vi "EM9636M系列_主VI.vi"() -> ()   [LabVIEW 2016]
uses:
  <vilib>/Modbus/subvis/Modbus API/Modbus API.lvclass/Modbus API.ctl
  <vilib>/Modbus/subvis/Transmission Data Unit (ADU)/Transmission Data Unit/Transmission Data Unit.lvclass/Transmission Data Unit.ctl
  <vilib>/Modbus/master/Data Access/Unit ID/Set Unit ID Property.vi
  <vilib>/Modbus/subvis/Transmission Data Unit (ADU)/Transmission Data Unit/Data Access/Unit ID/Write Unit ID.vi
  <vilib>/Modbus/subvis/Modbus API/Read Transmission Data Unit.vi
  <vilib>/Modbus/subvis/Modbus API/Write Transmission Data Unit.vi
  <vilib>/Modbus/master/Modbus Master.lvclass
  <vilib>/Utility/NIReport.llb/Append Text Table to Report (wrap).vi
  <vilib>/Modbus/master/Create Master Instance (Serial).vi
  <vilib>/Modbus/subvis/Transmission Data Unit (ADU)/Transmission Data Unit/Transmission Data Unit.lvclass
  <vilib>/Utility/NIReport.llb/NI_report.lvclass
  <vilib>/ptbypt/NI_PtbyPt.lvlib
  <vilib>/Utility/miscctls.llb/LVRectTypeDef.ctl
panel:
  out "ini_R3":bool
  out "ini_D6":bool
  out "ini_D5":bool
  out "表格名称":string
  out "车型":string
  in  "簇 3":T1
  out "R3":dbl format="%#.2g"
  out "R2":dbl format="%#.2g"
  out "R1":dbl format="%#.2g"
  out "D6":dbl format="%#.2g"
  out "D5":dbl format="%#.2g"
  out "D4":dbl format="%#.2g"
  out "D3":dbl format="%#.2g"
  out "D2":dbl format="%#.2g"
  out "D1":dbl format="%#.2g"
  in  "簇":T1
  out "数据":T2(array[cluster])
  out "comcnt":u16
  out "对话框":bool
  out "到期了":bool
  out "变频6":bool
  out "变频5":bool
  out "变频4":bool
  out "变频3":bool
  out "变频2":bool
  out "变频1":bool
  in  "加载电机右下正反转":bool
  out "加载右下转矩监控":i16 format="%#.0f"
  in  "加载电机右下启动":bool caption="停止"
  out "加载电机右下母线电流":dbl
  out "加载电机右下母线电压":dbl
  out "加载转速右下监控":dbl
  in  "加载电机右下转速给定":i32
  in  "加载电机右下停机":bool caption="停止"
  out "加载电机右下运行？":bool
  in  "加载电机右下转矩给定":i16
  out "加载电机左下运行？":bool
  in  "加载电机左下转速给定":i32
  out "加载左下转速监控":dbl
  out "加载电机左下母线电压":dbl
  out "加载电机左下母线电流":dbl
  out "加载左下转矩监控":i16
  in  "加载电机左下停机":bool caption="停止"
  in  "加载电机左下启动":bool caption="停止"
  in  "加载电机左下正反转":bool
  in  "加载电机左下转矩给定":i16
  in  "加载电机右上正反转":bool
  out "加载转矩右上监控":i16 format="%#.0f"
  in  "加载电机右上启动":bool caption="停止"
  out "加载电机右上母线电流":dbl
  out "加载电机右上母线电压":dbl
  out "加载右上转速监控":dbl
  in  "加载电机右上转速给定":i32
  in  "加载电机右上停机":bool caption="停止"
  out "加载电机右上运行？":bool
  in  "加载电机右上转矩给定":i16
  out "加载电机左上运行？":bool
  in  "加载电机左上转速给定":i32
  out "加载左上转速监控":dbl
  out "加载电机左上母线电压":dbl
  out "加载电机左上母线电流":dbl
  out "加载左上转矩监控":i16
  in  "加载电机左上停机":bool caption="停止"
  in  "加载电机左上启动":bool caption="停止"
  in  "加载电机左上正反转":bool
  in  "加载电机左上转矩给定":i16
  in  "驱动电机上正反转":bool
  out "驱动转矩上监控":i16 format="%#.0f"
  in  "驱动电机上转矩给定":i16
  in  "驱动电机上启动":bool caption="停止"
  out "驱动电机上母线电流":dbl
  out "驱动电机上母线电压":dbl
  out "驱动上转速监控":dbl
  in  "驱动电机上转速给定":i16
  in  "驱动电机上停机":bool caption="停止"
  out "驱动电机上运行？":bool
  in  "驱动电机下正反转":bool
  out "驱动转矩下监控":i16 format="%#.0f"
  in  "驱动电机下转矩给定":i16
  in  "驱动电机下启动":bool caption="停止"
  out "驱动电机下母线电流":dbl
  out "驱动电机下母线电压":dbl
  out "驱动转速下监控":dbl
  in  "驱动电机转速下给定":i16
  in  "驱动电机下停机":bool caption="停止"
  out "驱动电机下运行？":bool
  out "轮询耗时":u32
  out "数值":i32
  out "对话框传递":bool
  out "超温报警":bool
  out "遥控器通讯":bool
  out "变频串口":bool
  in  "加载电机复位":bool caption="停止"
  out "变频器":bool
  out "前右":bool[](array[boolean])
  out "前左":bool[](array[boolean])
  out "中右":bool[](array[boolean])
  out "中左":bool[](array[boolean])
  out "后右":bool[](array[boolean])
  out "后左":bool[](array[boolean])
  in  "倒计时间S":dbl=600.0
  out "错误输出 7":errorcluster caption="错误输出"
  out "确认输入布尔":bool
  out "等待进车布尔":bool
  out "Config":T9={"DevType"=2, "DevIndex"=0, "CanIndex"=0, "VCI_INIT_CONFIG"={"AccCode"=0, "AccMask"=0, "InitFlag"=0, "Fliter"=0, "Timing0"=0, "Timing1"=0, "Mode"=0}} {"DevType" items=["USB-CAN"=3, "USB-CAN2"=4]; "CanIndex" items=["通道1", "通道2"]; "VCI_INIT_CONFIG"."Fliter" items=["接收所有类型"=3, "只接收标准帧"=4, "只接收扩展帧"=7]; "VCI_INIT_CONFIG"."Mode" items=["正常工作", "自测模式（环回）", "仅侦听模式"]; "VCI_INIT_CONFIG"."InitFlag" items=["使用Flash参数", "使用界面设置参数"]}
  in  "D1扭矩给定":i16=500
  in  "D2扭矩给定":i16=1000
  in  "D3扭矩给定":i16=1500
  in  "D4扭矩给定":i16=2000
  in  "D5扭矩给定":i16=3500
  in  "D6扭矩给定":i16=4000
  in  "R1扭矩给定":i16=500
  in  "R2扭矩给定":i16=1000
  in  "R3扭矩给定":i16=1500
  out "发送左侧字符":bool
  in  "Close":bool
  in  "Open 2":bool
  in  "AD开始采集 2":bool
  in  "AD开始采集":bool
  out "输出数组右":dbl[][](array[numeric])
  out "输出数组左":dbl[][](array[numeric])
  out "采集卡右":bool
  out "采集卡左":bool
  out "Open":bool
  out "close2":bool
  out "close":bool
  out "当前实验时间":string
  out "元素 2":bool
  out "元素":bool
  out "元素 4":bool
  out "元素 3":bool
  in  "速度温度":string[][](array[string]) caption="文本数据"
  out "实验基本信息":string[][](array[string])
  out "字符布尔":bool
  in  "Reset 9":bool caption="重置"
  in  "Reset 8":bool caption="重置"
  in  "Reset 7":bool caption="重置"
  in  "Reset 6":bool caption="重置"
  in  "Reset 5":bool caption="重置"
  in  "Reset 4":bool caption="重置"
  in  "Reset 3":bool caption="重置"
  in  "Reset 2":bool caption="重置"
  in  "Reset":bool caption="重置"
  out "R3平均速度":dbl
  out "R2平均速度":dbl
  out "R1平均速度":dbl
  out "D6平均速度":dbl
  out "D5平均速度":dbl
  out "D4平均速度":dbl
  out "D3平均速度":dbl
  out "D2平均速度":dbl
  out "平均速度数组":dbl[](array[numeric])
  out "D1平均速度":dbl
  out "停止布尔 2":bool
  out "停止布尔":bool
  out "启动布尔":bool
  out "485启动给遥控器布尔":bool
  in  "左5字符":u8=85 format="%x"
  in  "左4字符":u8=85 format="%x"
  in  "左3字符":u8=85 format="%x"
  in  "左2字符":u8=85 format="%x"
  in  "左1字符":u8=85 format="%x"
  out "布尔数组 2":bool[](array[boolean])
  out "布尔数组":bool[](array[boolean])
  in  "kBaudRate":u8(ring)=10 caption="波特率" items=["5k bps"=1, "10k bps"=2, "20k bps"=3, "40k bps"=4, "50k bps"=5, "80k bps"=6, "100k bps"=7, "125k bps"=8, "200k bps"=9, "250k bps"=10, "400k bps"=11, "500k bps"=12, "666k bps"=13, "800k bps"=14, "1000k bps"=15, "33.33k bps"=16, "66.66k bps"=17, "83.33k bps"=18]
  in  "Channel":T4 caption="CAN通道" items=["通道1", "通道2"]
  in  "DevType":T3=2 caption="设备类型" items=["USB-CAN"=2, "USB-CAN2"=3]
  out "中间数组":string[](array[string])
  in  "数值 2":dbl
  out "系统时间 2":string="系统时间"
  in  "ID_VCU_MCU_1 8":u32=522 format="0x%x"
  in  "ID_VCU_MCU_2 5":u32=522 format="0x%x"
  in  "ID_VCU_MCU_33 4":u32=522 format="0x%x"
  in  "ID_VCU_MCU_1 7":u32=522 format="0x%x"
  in  "0byte 13":u8=64 format="%x"
  in  "1byte 13":u8=6 format="%x"
  in  "2byte 13":u8=80 format="%x"
  in  "3byte 13":u8=111 format="%x"
  in  "4byte 13":u8=119 format="%x"
  in  "5byte 13":u8=101 format="%x"
  in  "6byte 13":u8=114 format="%x"
  in  "7byte 13":u8=32 format="%x"
  in  "0byte 14":u8=70 format="%x"
  in  "1byte 14":u8=2 format="%x"
  in  "2byte 14":u8=32 format="%x"
  in  "3byte 14":u8=32 format="%x"
  in  "4byte 14":u8 format="%x"
  in  "5byte 14":u8 format="%x"
  in  "6byte 14":u8 format="%x"
  in  "7byte 14":u8 format="%x"
  in  "0byte 15":u8=96 format="%x"
  in  "1byte 15":u8=6 format="%x"
  in  "2byte 15":u8=84 format="%x"
  in  "3byte 15":u8=85 format="%x"
  in  "4byte 15":u8=114 format="%x"
  in  "5byte 15":u8=113 format="%x"
  in  "6byte 15":u8=117 format="%x"
  in  "7byte 15":u8=101 format="%x"
  in  "0byte 16":u8=102 format="%x"
  in  "1byte 16":u8=2 format="%x"
  in  "2byte 16":u8=32 format="%x"
  in  "3byte 16":u8=32 format="%x"
  in  "4byte 16":u8 format="%x"
  in  "5byte 16":u8 format="%x"
  in  "6byte 16":u8 format="%x"
  in  "7byte 16":u8 format="%x"
  in  "ID_VCU_MCU_1 6":u32=522 format="0x%x"
  in  "ID_VCU_MCU_2 4":u32=522 format="0x%x"
  in  "ID_VCU_MCU_33 3":u32=522 format="0x%x"
  in  "ID_VCU_MCU_1 5":u32=522 format="0x%x"
  in  "0byte 5":u8=16 format="%x"
  in  "1byte 5":u8=6 format="%x"
  in  "2byte 5":u8=85 format="%x"
  in  "3byte 5":u8=85 format="%x"
  in  "4byte 5":u8=85 format="%x"
  in  "5byte 5":u8=85 format="%x"
  in  "6byte 5":u8=85 format="%x"
  in  "7byte 5":u8=85 format="%x"
  in  "0byte 6":u8=86 format="%x"
  in  "1byte 6":u8=2 format="%x"
  in  "2byte 6":u8=75 format="%x"
  in  "3byte 6":u8=119 format="%x"
  in  "4byte 6":u8 format="%x"
  in  "5byte 6":u8 format="%x"
  in  "6byte 6":u8 format="%x"
  in  "7byte 6":u8 format="%x"
  in  "0byte 7":u8=48 format="%x"
  in  "1byte 7":u8=6 format="%x"
  in  "2byte 7":u8=85 format="%x"
  in  "3byte 7":u8=85 format="%x"
  in  "4byte 7":u8=85 format="%x"
  in  "5byte 7":u8=85 format="%x"
  in  "6byte 7":u8=85 format="%x"
  in  "7byte 7":u8=85 format="%x"
  in  "0byte 8":u8=118 format="%x"
  in  "1byte 8":u8=2 format="%x"
  in  "2byte 8":u8=78 format="%x"
  in  "3byte 8":u8=109 format="%x"
  in  "4byte 8":u8 format="%x"
  in  "5byte 8":u8 format="%x"
  in  "6byte 8":u8 format="%x"
  in  "7byte 8":u8 format="%x"
  in  "ID_VCU_MCU_1 2":u32=522 format="0x%x"
  in  "ID_VCU_MCU_33":u32=522 format="0x%x"
  in  "ID_VCU_MCU_2 2":u32=522 format="0x%x"
  in  "ID_VCU_MCU_1":u32=522 format="0x%x"
  in  "ID_VCU_MCU_1 4":u32=522 format="0x%x"
  in  "ID_VCU_MCU_2 3":u32=522 format="0x%x"
  in  "ID_VCU_MCU_33 2":u32=522 format="0x%x"
  in  "ID_VCU_MCU_1 3":u32=522 format="0x%x"
  in  "0byte 9":u8 format="%x"
  in  "1byte 9":u8=6 format="%x"
  in  "2byte 9":u8=71 format="%x"
  in  "3byte 9":u8=101 format="%x"
  in  "4byte 9":u8=97 format="%x"
  in  "5byte 9":u8=114 format="%x"
  in  "6byte 9":u8=32 format="%x"
  in  "7byte 9":u8=32 format="%x"
  in  "0byte 10":u8=6 format="%x"
  in  "1byte 10":u8=2 format="%x"
  in  "2byte 10":u8=32 format="%x"
  in  "3byte 10":u8=32 format="%x"
  in  "4byte 10":u8 format="%x"
  in  "5byte 10":u8 format="%x"
  in  "6byte 10":u8 format="%x"
  in  "7byte 10":u8 format="%x"
  in  "0byte 11":u8=32 format="%x"
  in  "1byte 11":u8=6 format="%x"
  in  "2byte 11":u8=83 format="%x"
  in  "3byte 11":u8=112 format="%x"
  in  "4byte 11":u8=101 format="%x"
  in  "5byte 11":u8=101 format="%x"
  in  "6byte 11":u8=100 format="%x"
  in  "7byte 11":u8=32 format="%x"
  in  "0byte 12":u8=38 format="%x"
  in  "1byte 12":u8=2 format="%x"
  in  "2byte 12":u8=32 format="%x"
  in  "3byte 12":u8=32 format="%x"
  in  "4byte 12":u8 format="%x"
  in  "5byte 12":u8 format="%x"
  in  "6byte 12":u8 format="%x"
  in  "7byte 12":u8 format="%x"
  in  "0byte 4":u8=54 format="%x"
  in  "1byte 4":u8=2 format="%x"
  in  "2byte 4":u8=80 format="%x"
  in  "3byte 4":u8=109 format="%x"
  in  "4byte 4":u8 format="%x"
  in  "5byte 4":u8 format="%x"
  in  "6byte 4":u8 format="%x"
  in  "7byte 4":u8 format="%x"
  in  "0byte 3":u8=48 format="%x"
  in  "1byte 3":u8=6 format="%x"
  in  "2byte 3":u8=85 format="%x"
  in  "3byte 3":u8=85 format="%x"
  in  "4byte 3":u8=85 format="%x"
  in  "5byte 3":u8=85 format="%x"
  in  "6byte 3":u8=85 format="%x"
  in  "7byte 3":u8=82 format="%x"
  in  "0byte 2":u8=22 format="%x"
  in  "1byte 2":u8=2 format="%x"
  in  "2byte 2":u8=32 format="%x"
  in  "3byte 2":u8=32 format="%x"
  in  "4byte 2":u8 format="%x"
  in  "5byte 2":u8 format="%x"
  in  "6byte 2":u8 format="%x"
  in  "7byte 2":u8 format="%x"
  out "选项卡控件 4":enum32{"VCU控制", "CAN基本操作"}(tab)
  in  "Clear":bool
  in  "Mode":T8 caption="工作模式" items=["正常工作", "仅侦听模式", "自测模式（环回）"]
  in  "Fliter":T7=1 items=["接收所有类型"=1, "只接收标准帧"=2, "只接收扩展帧"=3]
  in  "AccMask":u32=4294967295 caption="接收屏蔽码" format="%08x"
  in  "AccCode":u32 caption="接收过滤码" format="%08x"
  out "SendCnt":u32 caption="发送统计"
  out "RecvCnt":u32 caption="接收统计"
  in  "RcvEnable":bool=TRUE
  in  "list":i32(listbox)
  in  "Send":bool
  in  "ID":u32 format="0x%x"
  in  "Type":u8(ring) items=["数据帧", "远程帧"]
  in  "Format":u8(ring) items=["标准帧", "扩展帧"]
  in  "Data":string="01 00"
  in  "0byte":u8=16 format="%x"
  in  "1byte":u8=6 format="%x"
  in  "2byte":u8=85 format="%x"
  in  "3byte":u8=85 format="%x"
  in  "4byte":u8=85 format="%x"
  in  "5byte":u8=85 format="%x"
  in  "6byte":u8=85 format="%x"
  in  "7byte":u8=85 format="%x"
  in  "InitFlag":T6=1 caption="初始化参数" items=["使用Flash参数", "使用界面设置参数"]
  in  "选项卡控件 3":enum32{"数据监视", "查看数据"}(tab)
  in  "具体车型":string
  in  "确认换挡":bool
  in  "重新选档档位":T10(ring)
  out "前右":bool
  out "中右":bool
  out "后右":bool
  out "前左":bool
  out "中左":bool
  out "后左":bool
  out "R3S":dbl format="%#.2g"
  out "R2S":dbl format="%#.2g"
  out "R1S":dbl format="%#.2g"
  out "D6S":dbl format="%#.2g"
  out "D5S":dbl format="%#.2g"
  out "D4S":dbl format="%#.2g"
  out "D3S":dbl format="%#.2g"
  out "D2S":dbl format="%#.2g"
  out "D1S":dbl format="%#.2g"
  in  "刷新参数":bool
  out "LED屏幕信息":string
  in  "高级参数":bool
  in  "重新实验":bool
  in  "生成报表":bool
  in  "确认输入":bool
  in  "遥控器按钮确认":bool
  out "总实验时间":string
  out "前右":dbl format="%#.2g"
  out "前左":dbl format="%#.2g"
  out "中右":dbl
  out "中左":dbl format="%#.2g"
  out "后右":dbl format="%#.2g"
  out "后左":dbl format="%#.2g"
  out "后右":dbl format="%#.2g"
  out "后左":dbl format="%#.2g"
  out "中右":dbl format="%#.2g"
  out "中左":dbl format="%#.2g"
  out "前右":dbl format="%#.2g"
  out "前左":dbl format="%#.2g"
  out "环境温度标定":dbl format="%#.2g"
  out "波形图表":dynamicdata(graph)
  in  "操作者":string
  out "加载扭矩N.M(单个）":dbl
  out "当前试验档位":string
  in  "试验车型":u16(ring) items=["SG21", "SG14", "SG16", "SG18"]
  out "车速":dbl(knob) scale=-30.0..30.0
  in  "试验车编号":string
  in  "发动机编号":string
  out "加载功率":dbl(knob) scale=0.0..30.0
  in  "试验开始":bool caption="停止"
  in  "停止":bool
  out "液压油箱温度标定":dbl format="%#.2g"
  out "变矩器出口温度标定":dbl format="%#.2g"
  out "右前轮轴承温度标定":dbl format="%#.2g"
  out "左前轮轴承温度标定":dbl format="%#.2g"
  out "振动泵压力":dbl format="%#.2g"
  out "转向泵压力":dbl format="%#.2g"
  in  "密码输入":string
  out "SG14百分比":dbl
  out "SG16-3百分比":dbl
  out "SG18-3百分比":dbl
  out "D1 act":dbl format="%#.2g"
  out "D2 act":dbl format="%#.2g"
  out "R3 act":dbl format="%#.2g"
  out "R2 act":dbl format="%#.2g"
  out "R1 act":dbl format="%#.2g"
  out "D6 act":dbl format="%#.2g"
  out "D5 act":dbl format="%#.2g"
  out "D4 act":dbl format="%#.2g"
  out "D3 act":dbl format="%#.2g"
  out "数值 3":i32
  out "前右电机右轴承振动":dbl
  out "前右电机左轴承振动":dbl
  out "前右滚筒右轴承振动":dbl
  out "前右滚筒左轴承振动":dbl
  out "后左滚筒右振动":dbl
  out "后左滚筒左振动":dbl
  out "中右电机右振动":dbl
  out "中右电机左振动":dbl
  out "中右滚筒右振动":dbl
  out "中右滚筒左振动":dbl
  out "中左电机右轴承振动":dbl
  out "中左电机左轴承振动":dbl
  out "中左滚筒右轴承振动":dbl
  out "中左滚筒左轴承振动":dbl
  out "前左电机右轴承振动":dbl
  out "前左电机左轴承振动":dbl
  out "前左滚筒右轴承振动":dbl
  out "前左滚筒左轴承振动":dbl
  out "后右电机右振动":dbl
  out "后右电机左振动":dbl
  out "后右滚筒右振动":dbl
  out "后右滚筒左振动":dbl
  out "后左电机右振动":dbl
  out "后左电机左振动":dbl
  out "后右电机绕组":dbl
  out "后右电机右轴承":dbl
  out "后右滚筒左轴承":dbl
  out "后左滚筒右轴承":dbl
  out "后右滚筒左轴承":dbl
  out "后左电机绕组":dbl
  out "后左电机右轴承":dbl
  out "后左电机左轴承":dbl
  out "后左滚筒右轴承":dbl
  out "后左滚筒左轴承":dbl
  out "中右电机绕组":dbl
  out "中右电机右轴承":dbl
  out "中右电机左轴承":dbl
  out "中右滚筒右轴承":dbl
  out "中右滚筒左轴承":dbl
  out "中左电机绕组":dbl
  out "中左电机右轴承":dbl
  out "中左电机左轴承":dbl
  out "中左滚筒右轴承":dbl
  out "中左滚筒左轴承":dbl
  out "前右电机绕组":dbl
  out "前右电机右轴承":dbl
  out "前右滚筒左轴承":dbl
  out "前左滚筒右轴承":dbl
  out "前右滚筒左轴承":dbl
  out "前左电机绕组":dbl
  out "前左电机右轴承":dbl
  out "前左电机左轴承":dbl
  out "前左滚筒右轴承":dbl
  out "前左滚筒左轴承":dbl
  out "错误输出 6":errorcluster caption="错误输出"
  out "AD均值数据 2":dbl[](array[numeric])
  in  "M系列PWM停止 2":bool
  in  "编码器清零 2":bool
  in  "DA输出 2":bool
  in  "DA输出范围 2":i32(ring) items=["±10V", "±5V", "0~10V（默认）", "0~5V", "0~20mA"]
  in  "CH1 2":i16(slide) scale=0.0..10000.0
  in  "CH3 2":i16(slide) scale=0.0..10000.0
  in  "CH4 2":i16(slide) scale=0.0..10000.0
  in  "CH2 2":i16(slide) scale=0.0..10000.0
  in  "设定输出脉冲个数 2":u32
  in  "M系列PWM输出 2":bool
  in  "AD停止采集 2":bool
  out "布尔 2":bool
  in  "通道频率Hz 2":dbl=10000.0 min=1000.0 max=100000.0 step=10.0
  in  "组频率Hz 2":dbl=500.0
  in  "单双端 2":i32(ring) items=["单端", "双端"]
  in  "AD终止通道 2":i32=32
  in  "AD起始通道 2":i32=1
  in  "增益 2":i32(ring) items=["无增益", "2倍增益", "5倍增益", "10倍增益"]
  in  "伪同步 2":i32(ring) items=["非伪同步", "伪同步"]
  in  "时钟源 2":i32(ring) items=["内时钟", "外时钟"]
  out "每次总数据量 2":i32
  out "通道数量 2":i32
  in  "AD范围 2":enum16{"-10~+10V", "-5V~+5V", "0~10V", "0~5V"}(ring)=enum."0~10V"
  out "每通道数据量 2":i32
  out "编码器AB值 2":i32[](array[numeric])
  out "编码器过零值 2":i16[](array[numeric])
  out "错误输出 5":errorcluster caption="错误输出3"
  out "错误输出 4":errorcluster caption="错误输出2"
  out "设备句柄 2":i32=1
  in  "选项卡控件 2":enum32{"AD数值显示", "数字量I/O", "(标准)PWM", "计数器（测频）"}(tab)
  in  "设置开关量方向 3":bool
  out "数组 5":dbl[](array[numeric])=[1.0, 2.0, 3.0, 4.0, 5.0, 6.0, 7.0, 8.0]
  out "数组 6":dbl[](array[numeric])=[1.0, 2.0, 3.0, 4.0, 5.0, 6.0, 7.0, 8.0]
  in  "光隔离输出 2":bool[](array[boolean])=[FALSE, FALSE, FALSE, FALSE, FALSE, FALSE, FALSE, FALSE]
  out "光隔离输入 2":bool[](array[boolean])
  in  "设置开关量方向 2":cluster{"IO1~IO8":i8, "IO9~IO16":i8}={"IO1~IO8"=1, "IO9~IO16"=1} {"IO9~IO16" items=["输入", "输出"]; "IO1~IO8" items=["输入", "输出"]}
  out "数组 7":i8[](array[numeric])
  in  "可编程数字量I/O 2":T11
  out "可编程数字量I/O(映射控件)--得到所有通道开关量值 2":T11
  in  "PWM输出 2":bool
  in  "PWM停止 2":bool
  in  "频率1 2":dbl=1000.0
  in  "占空比(0~1) 6":dbl=0.5
  out "实际频率 6":dbl
  out "实际占空比 6":dbl
  in  "频率2 2":dbl=5000.0
  in  "占空比(0~1) 5":dbl=0.5
  out "实际频率 5":dbl
  out "实际占空比 5":dbl
  in  "频率3 2":dbl=100000.0
  in  "占空比(0~1) 4":dbl=0.5
  out "实际频率 4":dbl
  out "实际占空比 4":dbl
  in  "开启计数 2":bool
  in  "计数器清零 2":bool
  in  "工作方式 2":u16(ring)=1 items=["计数", "测频"]
  out "计数/测频（Hz）值 2":dbl[](array[numeric])
  in  "编码器清零":bool
  out "编码器AB值":i32[](array[numeric])
  out "编码器过零值":i16[](array[numeric])
  in  "设定输出脉冲个数":u32
  in  "M系列PWM输出":bool
  in  "M系列PWM停止":bool
  in  "CH4":i16(slide) scale=0.0..10000.0
  in  "CH3":i16(slide) scale=0.0..10000.0
  in  "CH2":i16(slide) scale=0.0..10000.0
  in  "CH1":i16(slide) scale=0.0..10000.0
  in  "DA输出":bool
  in  "DA输出范围":i32(ring) items=["±10V", "±5V", "0~10V（默认）", "0~5V", "0~20mA"]
  out "每通道数据量":i32
  out "AD均值数据":dbl[](array[numeric])
  out "布尔":bool
  in  "AD停止采集":bool
  out "错误输出 3":errorcluster caption="错误输出3"
  out "错误输出 2":errorcluster caption="错误输出2"
  in  "选项卡控件":enum32{"AD数值显示", "数字量I/O", "(标准)PWM", "计数器（测频）"}(tab)
  out "变频故障1":bool
  out "变频故障2":bool
  out "变频故障 3":bool
  out "变频故障 4":bool
  out "变频故障5":bool
  out "变频故障 6":bool
  in  "设置开关量方向":bool
  out "数组 3":dbl[](array[numeric])=[1.0, 2.0, 3.0, 4.0, 5.0, 6.0, 7.0, 8.0]
  out "数组 2":dbl[](array[numeric])=[1.0, 2.0, 3.0, 4.0, 5.0, 6.0, 7.0, 8.0]
  in  "光隔离输出":bool[](array[boolean])=[FALSE, FALSE, FALSE, FALSE, FALSE, FALSE, FALSE, FALSE]
  out "光隔离输入":bool[](array[boolean])
  in  "设置开关量方向":cluster{"IO1~IO8":i8, "IO9~IO16":i8}={"IO1~IO8"=1, "IO9~IO16"=1} {"IO9~IO16" items=["输入", "输出"]; "IO1~IO8" items=["输入", "输出"]}
  out "数组 4":i8[](array[numeric])
  in  "可编程数字量I/O":T11
  out "可编程数字量I/O(映射控件)--得到所有通道开关量值":T11
  in  "PWM输出":bool
  in  "PWM停止":bool
  in  "频率1":dbl=1000.0
  in  "占空比(0~1)":dbl=0.5
  out "实际频率":dbl
  out "实际占空比":dbl
  in  "频率2":dbl=5000.0
  in  "占空比(0~1) 2":dbl=0.5
  out "实际频率 2":dbl
  out "实际占空比 2":dbl
  in  "频率3":dbl=100000.0
  in  "占空比(0~1) 3":dbl=0.5
  out "实际频率 3":dbl
  out "实际占空比 3":dbl
  in  "开启计数":bool
  in  "计数器清零":bool
  in  "工作方式":u16(ring)=1 items=["计数", "测频"]
  out "计数/测频（Hz）值":dbl[](array[numeric])
  in  "AD范围":enum16{"-10~+10V", "-5V~+5V", "0~10V", "0~5V"}(ring)=enum."0~10V"
  out "通道数量":i32
  out "设备句柄":i32=1
  out "错误输出":errorcluster
  out "每次总数据量":i32
  in  "时钟源":i32(ring) items=["内时钟", "外时钟"]
  in  "伪同步":i32(ring) items=["非伪同步", "伪同步"]
  in  "增益":i32(ring) items=["无增益", "2倍增益", "5倍增益", "10倍增益"]
  in  "AD起始通道":i32=1
  in  "AD终止通道":i32=32
  in  "单双端":i32(ring) items=["单端", "双端"]
  in  "组频率Hz":dbl=500.0
  in  "通道频率Hz":dbl=10000.0 min=1000.0 max=100000.0 step=10.0
  in  "数据端口":i32=8001
  in  "命令端口":i32=8000
  in  "IP地址":string="192.168.1.125"
  # "加载电机右上"
  # "驱动电机上"
  # "加载电机左上"
  # "r/min"
  # "r/min"
  # "r/min"
  # "转速"
  # "给定"
  # "转速"
  # "给定"
  # "转速"
  # "给定"
  # "给定"
  # "Nm"
  # "Nm"
  # "Nm"
  # "转矩"
  # "转矩"
  # "给定"
  # "转矩"
  # "给定"
  # "山推平地机实验台"
  # "电压"
  # "电流"
  # "电压"
  # "电流"
  # "电压"
  # "V"
  # "电流"
  # "A"
  # "A"
  # "V"
  # "A"
  # "V"
  # "遥控器"
  # "变频器"
  # "采集卡左"
  # "采集卡右"
  # "超温报警"
  # "正转"
  # "反转"
  # "正转"
  # "正转"
  # "反转"
  # "反转"
  # "加载电机右下"
  # "驱动电机下"
  # "加载电机左下"
  # "r/min"
  # "r/min"
  # "r/min"
  # "转速"
  # "给定"
  # "转速"
  # "给定"
  # "转速"
  # "给定"
  # "给定"
  # "Nm"
  # "Nm"
  # "Nm"
  # "转矩"
  # "转矩"
  # "给定"
  # "转矩"
  # "给定"
  # "电压"
  # "电流"
  # "电压"
  # "电流"
  # "电压"
  # "V"
  # "电流"
  # "A"
  # "V"
  # "A"
  # "V"
  # "A"
  # "正转"
  # "反转"
  # "正转"
  # "正转"
  # "反转"
  # "反转"
  # "D1"
  # "D6扭矩给定"
  # "~"
  # "R1"
  # "R3扭矩给定"
  # "~"
  # "EM9636M系列--LabView例程"
  # "CH1"
  # "CH2"
  # "如果设为0，则表示连续输出"
  # "CH1"
  # "CH2"
  # "位置传感器故障"
  # "过流"
  # "控制器过温"
  # "电机过温"
  # "欠压报警"
  # "过压报警"
  # "通讯故障"
  # "控制器高温"
  # "短路保护"
  # "严重欠压"
  # "超过峰值功率"
  # "超过最高限速"
  # "VCU故障"
  # "跛行状态"
  # "堵转保护"
  # "致命故障"
  # "车辆参数"
  # "设备参数"
  # "环境温度"
  # "前左"
  # "℃"
  # "℃"
  # "r/min"
  # "r/min"
  # "r/min"
  # "液压油箱温度"
  # "℃"
  # "前右"
  # "℃"
  # "r/min"
  # "r/min"
  # "r/min"
  # "变速箱温度"
  # "℃"
  # "中左"
  # "℃"
  # "右前轮轴承温度"
  # "中右"
  # "℃"
  # "℃"
  # "左前轮轴承温度"
  # "~"
  # "D1   R3/%"
  # "℃"
  # "后左"
  # "℃"
  # "~"
  # "D1   R3/S"
  # "Mp"
  # "工作泵压力"
  # "后右"
  # "℃"
  # "转向泵压力"
  # "Mp"
  # "前左滚筒左轴承"
  # "后左滚筒左轴承"
  # "℃"
  # "℃"
  # "后左电机左振动"
  # "前右滚筒左振动"
  # "前左滚筒右轴承"
  # "后左滚筒右轴承"
  # "℃"
  # "℃"
  # "后左电机右振动"
  # "前右滚筒右振动"
  # "前左电机左轴承"
  # "后左电机左轴承"
  # "℃"
  # "后右滚筒左振动"
  # "℃"
  # "前右电机左振动"
  # "前左电机右轴承"
  # "后左电机右轴承"
  # "℃"
  # "℃"
  # "后右滚筒右振动"
  # "前右电机右振动"
  # "前左电机绕组"
  # "后左电机绕组"
  # "后右电机左振动"
  # "℃"
  # "℃"
  # "前右滚筒左轴承"
  # "后右滚筒左轴承"
  # "后右电机右振动"
  # "℃"
  # "℃"
  # "前右滚筒右轴承"
  # "后右滚筒右轴承"
  # "前左滚筒左振动"
  # "℃"
  # "℃"
  # "前右电机左轴承"
  # "后右电机左轴承"
  # "前右滚筒右振动"
  # "℃"
  # "℃"
  # "前右电机右轴承"
  # "后右电机右轴承"
  # "前左电机左振动"
  # "℃"
  # "℃"
  # "前右电机绕组"
  # "后右电机绕组"
  # "℃"
  # "℃"
  # "前左电机右振动"
  # "中左滚筒左轴承"
  # "℃"
  # "中左滚筒左振动"
  # "中左滚筒右轴承"
  # "℃"
  # "中左滚筒右振动"
  # "中左电机左轴承"
  # "中左电机左振动"
  # "℃"
  # "中左电机右轴承"
  # "℃"
  # "中左电机右振动"
  # "中左电机绕组"
  # "℃"
  # "中右滚筒左振动"
  # "中右滚筒左轴承"
  # "中右滚筒右振动"
  # "℃"
  # "中右滚筒右轴承"
  # "中右电机左振动"
  # "℃"
  # "中右电机左轴承"
  # "中右电机右振动"
  # "℃"
  # "中右电机右轴承"
  # "后左滚筒左振动"
  # "℃"
  # "中右电机绕组"
  # "℃"
  # "后左滚筒右振动"
  # "通道3"
  # "通道1"
  # "通道2"
  # "频率，250Hz~500KHz\n占空比，0~1"
  # "通道3"
  # "通道1"
  # "通道2"
  # "频率，250Hz~500KHz\n占空比，0~1"
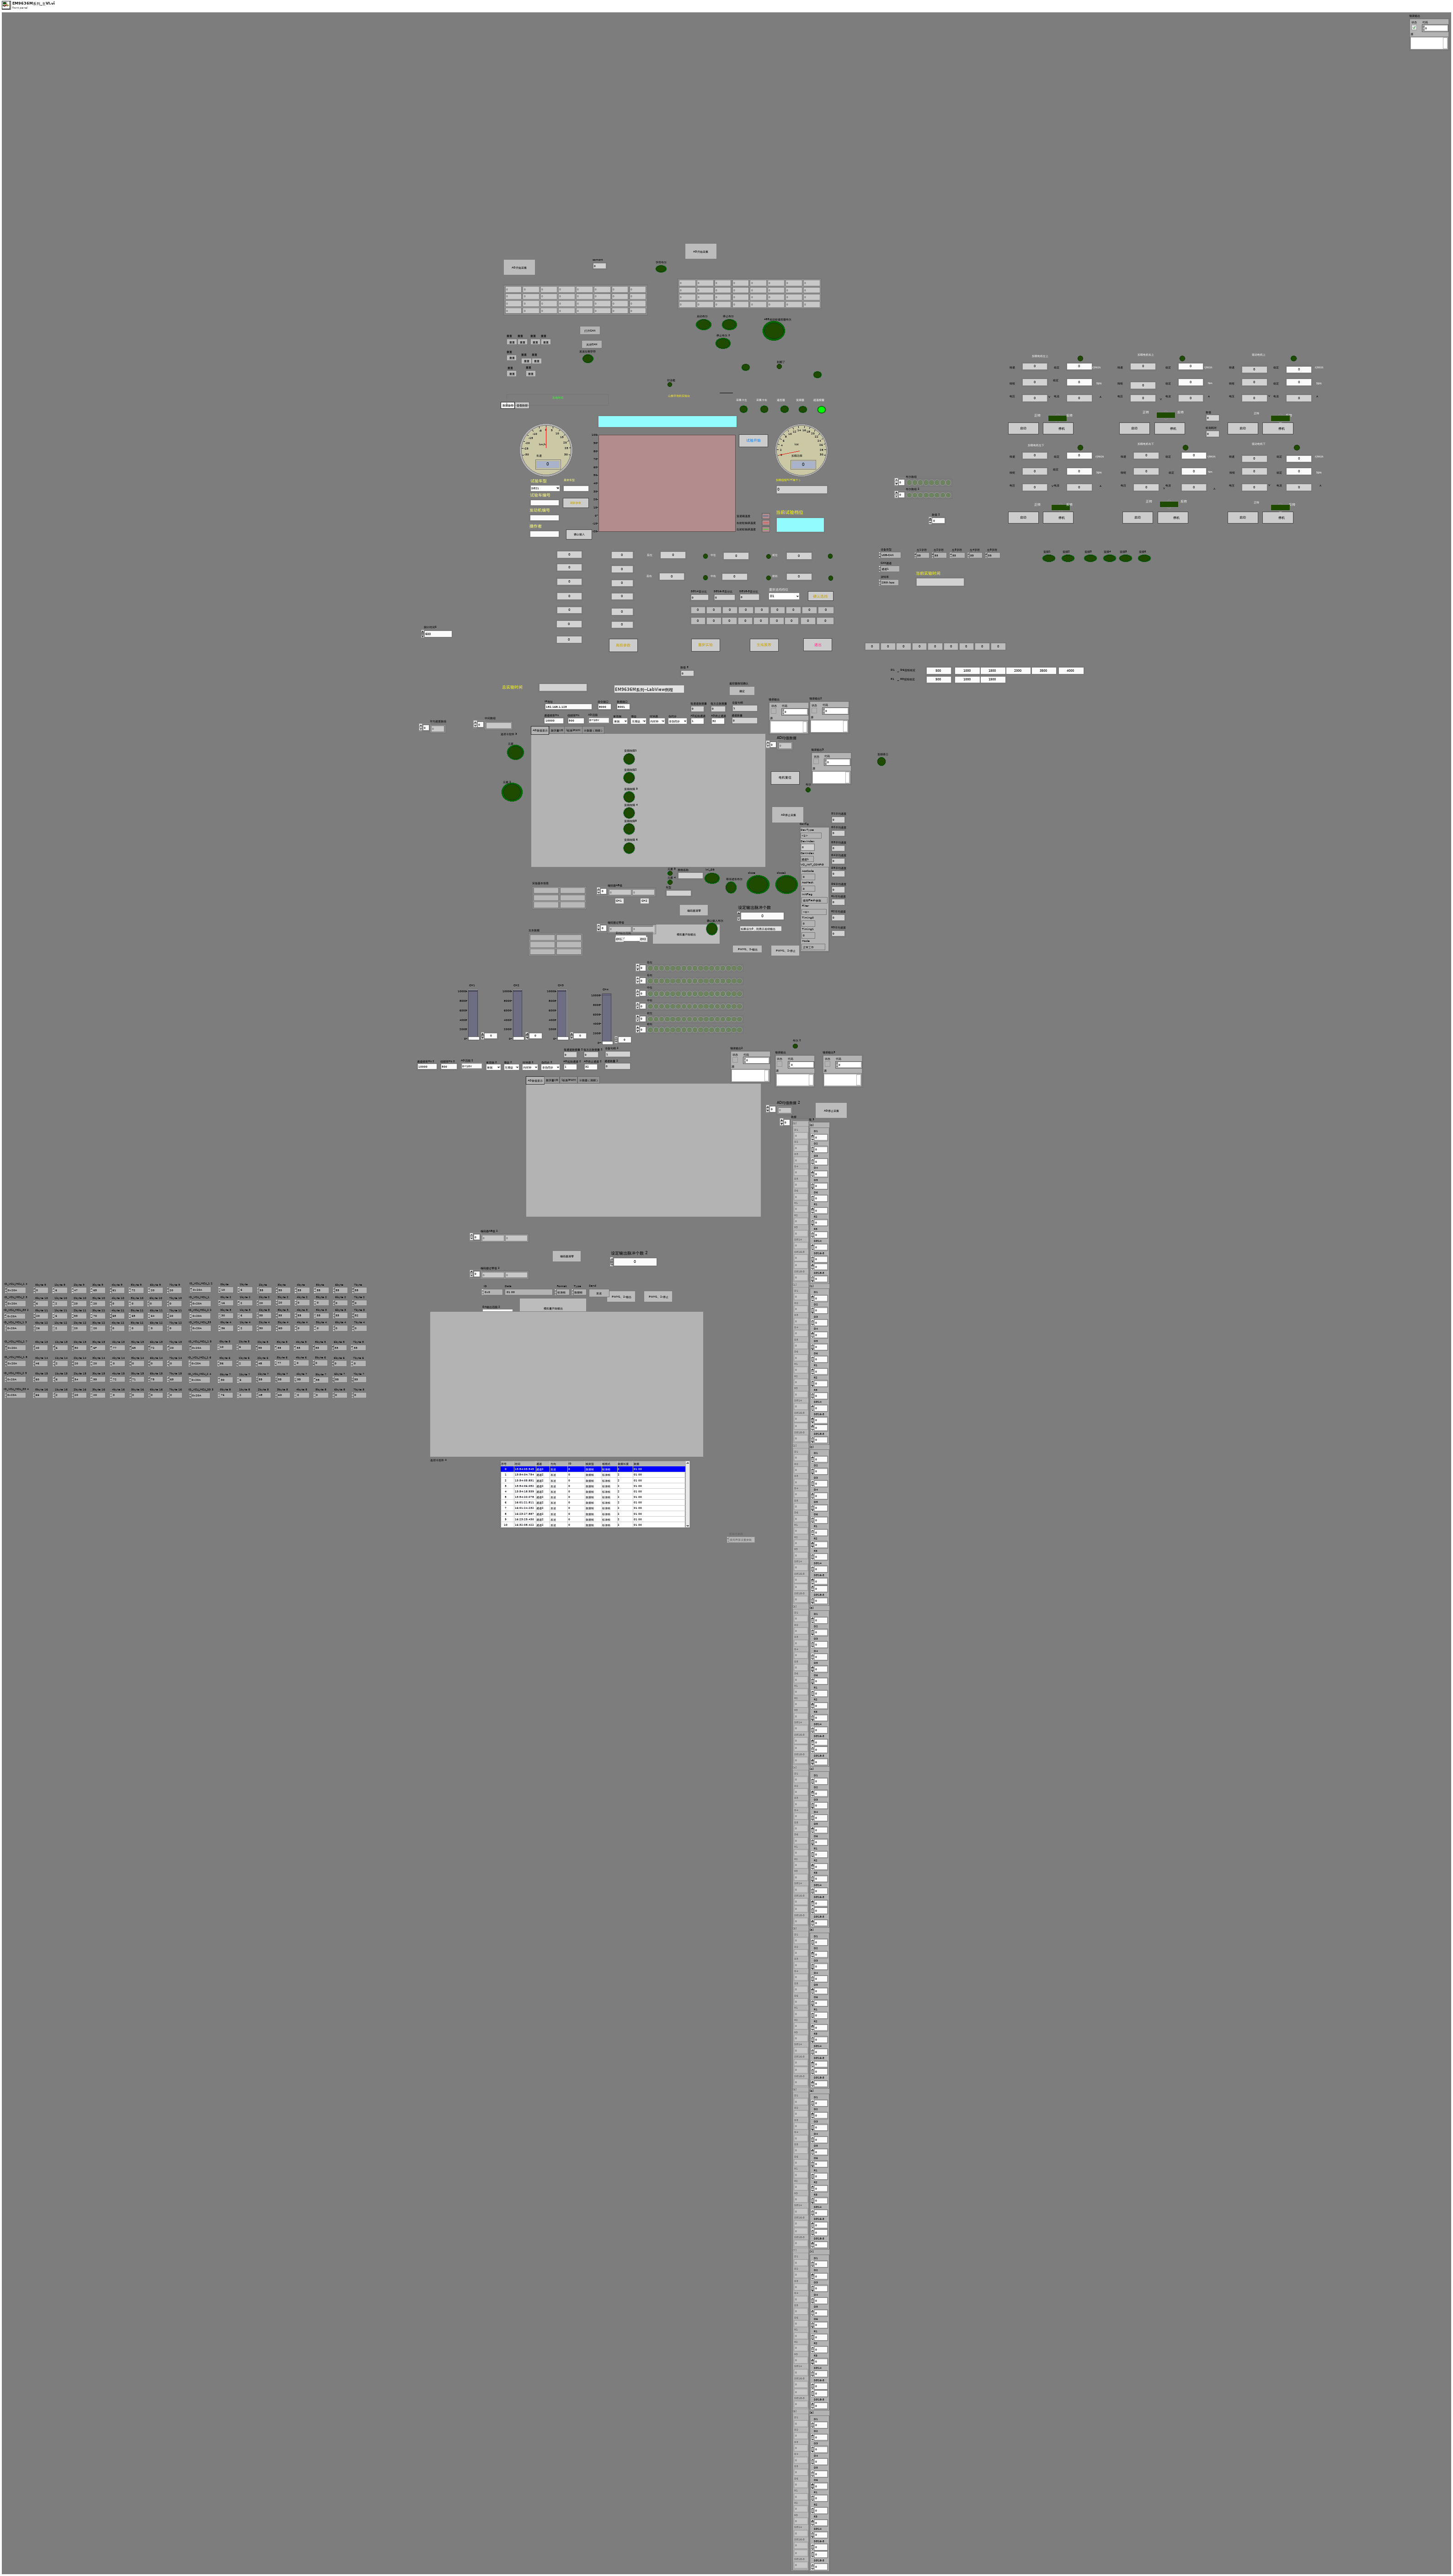
[diagram p1: front panel]
types:
  T1 = cluster{"[0]":cluster{"D1":dbl, "D2":dbl, "D3":dbl, "D4":dbl, "D5":dbl, "D6":dbl, "R1":dbl, "R2":dbl, "R3":dbl, "SG14":dbl, "SG16-3":dbl, dbl, "SG18-3 ":dbl}, "[1]":cluster{"D1":dbl, "D2":dbl, "D3":dbl, "D4":dbl, "D5":dbl, "D6":dbl, "R1":dbl, "R2":dbl, "R3":dbl, "SG14":dbl, "SG16-3":dbl, dbl, "SG18-3 ":dbl}, "[2]":cluster{"D1":dbl, "D2":dbl, "D3":dbl, "D4":dbl, "D5":dbl, "D6":dbl, "R1":dbl, "R2":dbl, "R3":dbl, "SG14":dbl, "SG16-3":dbl, dbl, "SG18-3 ":dbl}, "[3]":cluster{"D1":dbl, "D2":dbl, "D3":dbl, "D4":dbl, "D5":dbl, "D6":dbl, "R1":dbl, "R2":dbl, "R3":dbl, "SG14":dbl, "SG16-3":dbl, dbl, "SG18-3 ":dbl}, "[4]":cluster{"D1":dbl, "D2":dbl, "D3":dbl, "D4":dbl, "D5":dbl, "D6":dbl, "R1":dbl, "R2":dbl, "R3":dbl, "SG14":dbl, "SG16-3":dbl, dbl, "SG18-3 ":dbl}, "[5]":cluster{"D1":dbl, "D2":dbl, "D3":dbl, "D4":dbl, "D5":dbl, "D6":dbl, "R1":dbl, "R2":dbl, "R3":dbl, "SG14":dbl, "SG16-3":dbl, dbl, "SG18-3 ":dbl}, "[6]":cluster{"D1":dbl, "D2":dbl, "D3":dbl, "D4":dbl, "D5":dbl, "D6":dbl, "R1":dbl, "R2":dbl, "R3":dbl, "SG14":dbl, "SG16-3":dbl, dbl, "SG18-3 ":dbl}, "[7]":cluster{"D1":dbl, "D2":dbl, "D3":dbl, "D4":dbl, "D5":dbl, "D6":dbl, "R1":dbl, "R2":dbl, "R3":dbl, "SG14":dbl, "SG16-3":dbl, dbl, "SG18-3 ":dbl}, "[8]":cluster{"D1":dbl, "D2":dbl, "D3":dbl, "D4":dbl, "D5":dbl, "D6":dbl, "R1":dbl, "R2":dbl, "R3":dbl, "SG14":dbl, "SG16-3":dbl, dbl, "SG18-3 ":dbl}}
  T2 = cluster{"[0]":cluster{"D1":dbl, "D2":dbl, "D3":dbl, "D4":dbl, "D5":dbl, "D6":dbl, "R1":dbl, "R2":dbl, "R3":dbl, "SG14":dbl, "SG16-3":dbl, dbl, "SG18-3 ":dbl}, "[1]":cluster{"D1":dbl, "D2":dbl, "D3":dbl, "D4":dbl, "D5":dbl, "D6":dbl, "R1":dbl, "R2":dbl, "R3":dbl, "SG14":dbl, "SG16-3":dbl, dbl, "SG18-3 ":dbl}, "[2]":cluster{"D1":dbl, "D2":dbl, "D3":dbl, "D4":dbl, "D5":dbl, "D6":dbl, "R1":dbl, "R2":dbl, "R3":dbl, "SG14":dbl, "SG16-3":dbl, dbl, "SG18-3 ":dbl}, "[3]":cluster{"D1":dbl, "D2":dbl, "D3":dbl, "D4":dbl, "D5":dbl, "D6":dbl, "R1":dbl, "R2":dbl, "R3":dbl, "SG14":dbl, "SG16-3":dbl, dbl, "SG18-3 ":dbl}, "[4]":cluster{"D1":dbl, "D2":dbl, "D3":dbl, "D4":dbl, "D5":dbl, "D6":dbl, "R1":dbl, "R2":dbl, "R3":dbl, "SG14":dbl, "SG16-3":dbl, dbl, "SG18-3 ":dbl}, "[5]":cluster{"D1":dbl, "D2":dbl, "D3":dbl, "D4":dbl, "D5":dbl, "D6":dbl, "R1":dbl, "R2":dbl, "R3":dbl, "SG14":dbl, "SG16-3":dbl, dbl, "SG18-3 ":dbl}, "[6]":cluster{"D1":dbl, "D2":dbl, "D3":dbl, "D4":dbl, "D5":dbl, "D6":dbl, "R1":dbl, "R2":dbl, "R3":dbl, "SG14":dbl, "SG16-3":dbl, dbl, "SG18-3 ":dbl}, "[7]":cluster{"D1":dbl, "D2":dbl, "D3":dbl, "D4":dbl, "D5":dbl, "D6":dbl, "R1":dbl, "R2":dbl, "R3":dbl, "SG14":dbl, "SG16-3":dbl, dbl, "SG18-3 ":dbl}, "[8]":cluster{"D1":dbl, "D2":dbl, "D3":dbl, "D4":dbl, "D5":dbl, "D6":dbl, "R1":dbl, "R2":dbl, "R3":dbl, "SG14":dbl, "SG16-3":dbl, dbl, "SG18-3 ":dbl}}[]
  T3 = typedef "ControlCAN.lvlib/DevType.ctl" = u32
  T4 = typedef "ControlCAN.lvlib/CAN Channel.ctl" = u32
  T5 = typedef "ControlCAN.lvlib/VCI_INIT_CONFIG.ctl" = cluster{"AccCode":u32, "AccMask":u32, "InitFlag":T6, "Fliter":T7, "Timing0":u8, "Timing1":u8, "Mode":T8}
  T6 = typedef "ControlCAN.lvlib/InitFlag.ctl" = u32
  T7 = typedef "ControlCAN.lvlib/Fliter.ctl" = u8
  T8 = typedef "ControlCAN.lvlib/Mode.ctl" = u8
  T9 = cluster{"DevType":T3, "DevIndex":u32, "CanIndex":T4, "VCI_INIT_CONFIG":T5}
  T10 = enum16{"D1", "D2", "D3", "D4", "D5", "D6", "R1", "R2", "R3"}
  T11 = cluster{"CH1":bool, "CH2":bool, "CH3":bool, "CH4":bool, "CH5":bool, "CH6":bool, "CH7":bool, "CH8":bool, "CH9":bool, "CH10":bool, "CH11":bool, "CH12":bool, "CH13":bool, "CH14":bool, "CH15":bool, "CH16":bool}
  T12 = typedef "ControlCAN.lvlib/VCI_CAN_OBJ.ctl" = cluster{"ID":u32, "TimeStamp":u32, "TimeFlag":u8, "SendType":u8, "RemoteFlag":u8, "ExternFlag":u8, "DataLen":u8, "Data":u8[], "Reserved":u8[]}
  T13 = cluster{"Type":enum16{"接收", "发送"}, "Channel":T4, "Time":timestamp, "VCI_CAN_OBJ":T12}[]
  T14 = typedef "LVRectTypeDef.ctl" = cluster{"Left":i16, "Top":i16, "Right":i16, "Bottom":i16}
  T15 = cluster{"position (excel)":cluster{"row":i32, "column":i32}, "name (excel)":string, "bookmark (word)":string}
  T16 = enum16{"Standard Report", "HTML", "Word", "Excel"}
  T17 = enum32{"Invalid", "Standard", "Closed", "Hidden", "Minimized", "Maximized"}
  T18 = cluster{"D1":dbl, "D2":dbl, "D3":dbl, "D4":dbl, "D5":dbl, "D6":dbl, "R1":dbl, "R2":dbl, "R3":dbl, "SG14":dbl, "SG16-3":dbl, dbl, "SG18-3 ":dbl}
  T19 = enum32{"invalid app kind", "Development System", "Run Time System", "Student Edition", "Embedded LabVIEW", "Evaluation", "Custom"}
  T20 = cluster{"Type":enum16{"接收", "发送"}, "Channel":T4, "Time":timestamp, "VCI_CAN_OBJ":T12}
  T21 = typedef "ControlCAN.lvlib/Return Val.ctl" = i32
  T22 = cluster{"[0]":bool, "[1]":bool, "[2]":bool, "[3]":bool, "[4]":bool, "[5]":bool, "[6]":bool, "[7]":bool, "[8]":bool, "[9]":bool, "[10]":bool, "[11]":bool, "[12]":bool, "[13]":bool, "[14]":bool, "[15]":bool}
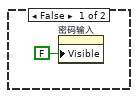
[diagram p4: hidden frame]
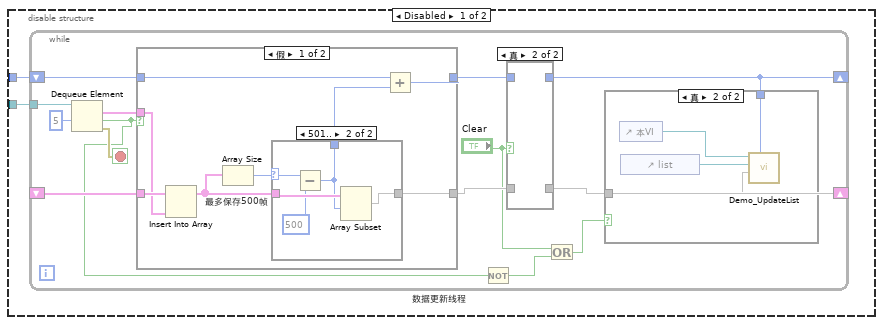
[diagram p8: hidden frame]
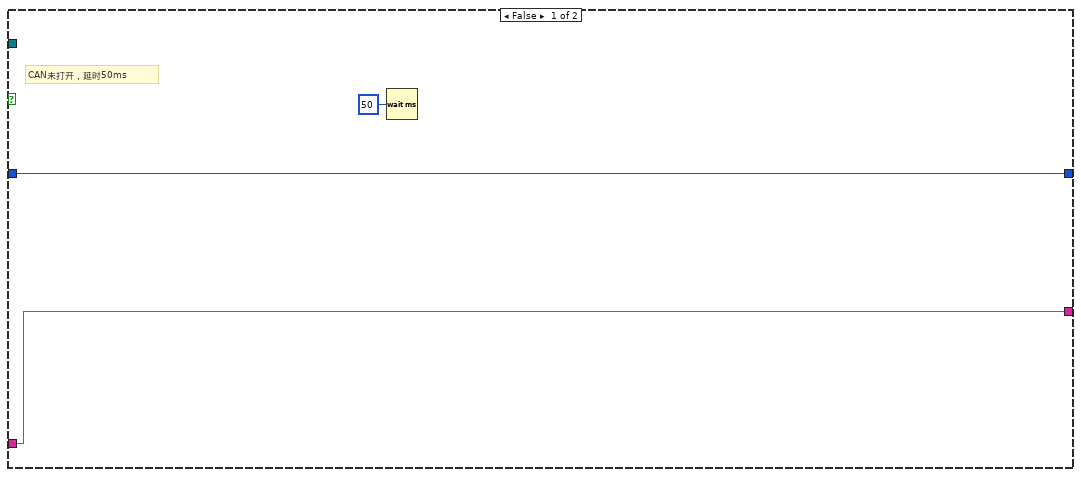
[diagram p13: hidden frame]
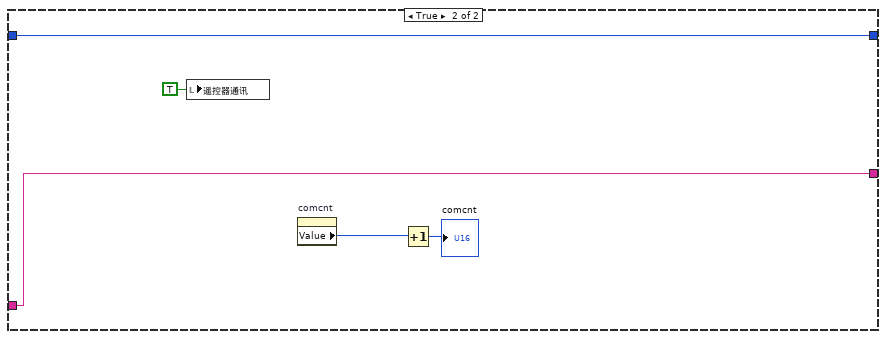
[diagram p16: hidden frame]
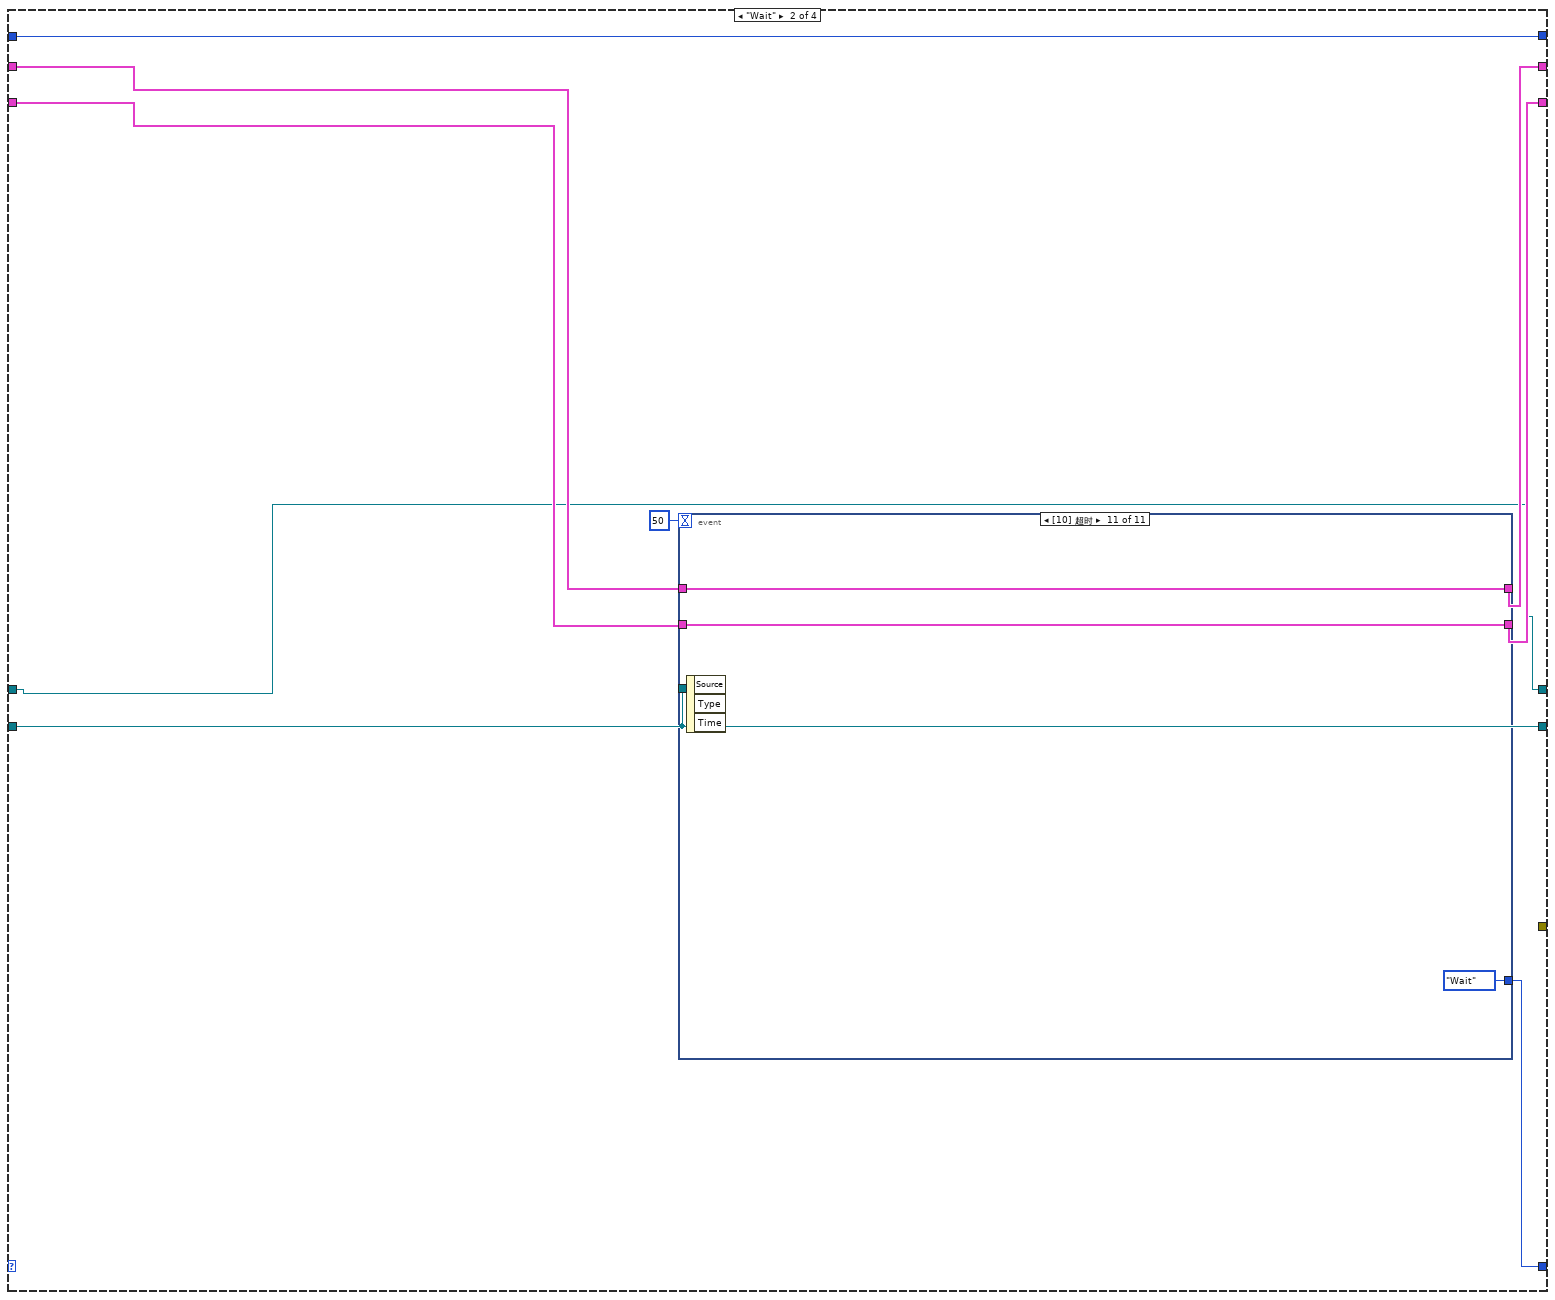
[diagram p17: hidden frame]
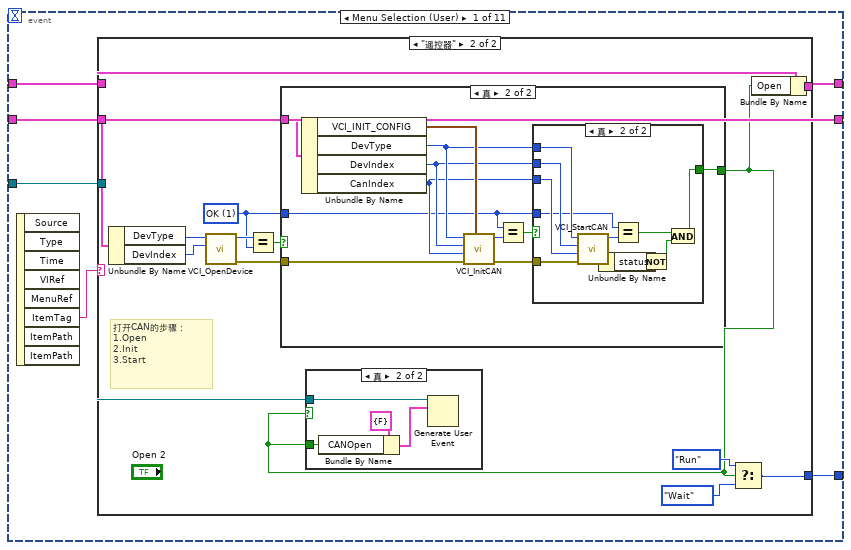
[diagram p18: hidden frame]
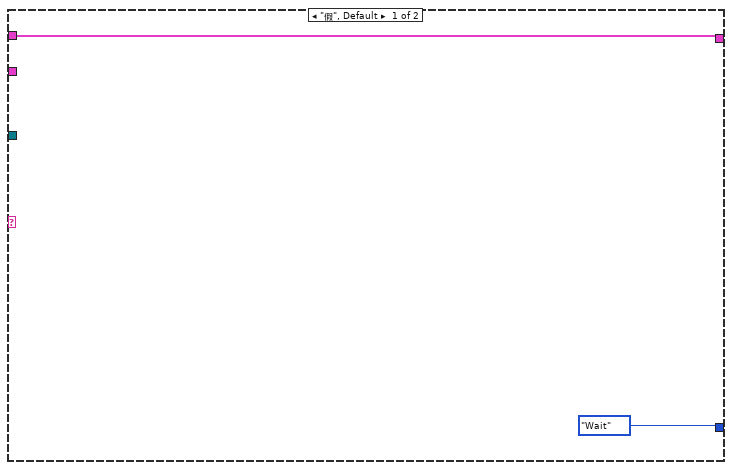
[diagram p19: hidden frame]
diagram:
  # "今天改了CAN"
  # "实验开始前平均速度要清零"
  n1 = disable-structure shown="启用" {
    disable-tunnel: [w29 _] -> w26
    frame Disabled {
      n2 = Obtain Queue(name (unnamed)="数据显示队列" ("名称（未命名）"), element data type=T13 []) -> (queue out=w29:refnum<queue>)  [unwired: 3 in, 2 out]
    }
    frame Enabled {
    }
  }
  n3 = disable-structure shown="禁用" {
    frame Disabled {
      n4 = property on="加载电机左下启动" class="Bool (严格)"("Val(Sgnl)"=FALSE ("值(信号)")) -> ()  [unwired: 2 in, 2 out]
      n5 = property on="驱动电机下启动" class="Bool (严格)"("Val(Sgnl)"=FALSE ("值(信号)")) -> ()  [unwired: 2 in, 2 out]
      n6 = property on="加载电机左上启动" class="Bool (严格)"("Val(Sgnl)"=FALSE ("值(信号)")) -> ()  [unwired: 2 in, 2 out]
      n7 = property on="加载电机右上启动" class="Bool (严格)"("Val(Sgnl)"=FALSE ("值(信号)")) -> ()  [unwired: 2 in, 2 out]
      n8 = property on="加载电机右下启动" class="Bool (严格)"("Val(Sgnl)"=FALSE ("值(信号)")) -> ()  [unwired: 2 in, 2 out]
      n9 = property on="驱动电机上启动" class="Bool (严格)"("Val(Sgnl)"=FALSE ("值(信号)")) -> ()  [unwired: 2 in, 2 out]
    }
    frame Enabled {
    }
  }
  n10 = flat-sequence {
    tunnel: [w45] -> w23
    tunnel: [w42] -> w22
    tunnel: [w49] -> w25
    tunnel: [w48] -> w24
    tunnel: w23 -> [w47]
    tunnel: w22 -> [w46]
    frame #0 {
      w37 = u16 0 items=["无", "奇", "偶"] ("parity (Even)")
      w44 = TRUE
      n11 = call-poly <vilib>:"Create Master Instance.vi"("serial type"=enum16{"RTU", "ASCII"}."RTU", "parity (Even)"=w37, "unit ID"=u8 1, "baud rate (9600)"=u32 9600, "VISA resource name"=refnum<visa-resource-name> "COM1") -> ("error out"=w42:errorcluster, "serial master instance"=w45:refnum<class "Modbus Master.lvclass">)  [unwired: 5 in]
      n12 = local write "停止"(FALSE ("停止")) -> ()
      n13 = Not(x=w42) -> (.not. x?=→"变频串口":bool)
      "变频1" <- w44
      "变频2" <- w44
      "变频3" <- w44
      "变频4" <- w44
      "变频5" <- w44
      "变频6" <- w44
    }
    frame #1 {
      n14 = while {
        shift-right: [w57] -> _
        shift-left: _ -> [w58]
        tunnel: [w55] -> w49
        shift-right: [w54] -> w48
        shift-left: w47 -> [w60]
        tunnel: w46 -> [w53]
        i -> [w52]
        stop <- w59 stop-if-true
        n15 = Tick Count (ms)() -> (millisecond timer value=w57:u32)
        n16 = Greater?(x=w52, y=2) -> (0:w50:bool)
        n17 = Subtract(x=w57, y=w58) -> (x-y=→"轮询耗时":u32)
        n18 = for {
          N: 6 -> [_]
          tunnel: w60 -> [w66]
          tunnel: [w65] -> w54
          shift-right: [w63] -> w55
          shift-left: w53 -> [w64]
          i -> [w68]
          n19 = Increment(x=w68) -> (x+1=w67:i32)
          n20 = case shown="1, 默认" w67 {
            tunnel: w66 -> [w145 w221 w326 w434 w547 w683]
            tunnel: [w111 w219 w324 w429 w548 w681] -> w65
            tunnel: w64 -> [w110 w220 w325 w433 w546 w682]
            tunnel: [w106 w214 w318 w428 w541 w676] -> w63
            frame 1, Default {
              w102 = 200 ("read operation timeout (ms)")
              n21 = local read "变频1"() -> (w140:bool)
              n22 = call <vilib>:"Set Unit ID.vi"("error in (no error)"=w110, "unit ID"=u8 1, "Modbus master in"=w145) -> ("error out"=w109:errorcluster, "Modbus master out"=w143:refnum<class "Modbus Master.lvclass">)  [unwired: 7 in]
              n23 = case shown="真" w140 {
                tunnel: w143 -> [w168 w173]
                tunnel: [w167 w172] -> w142
                tunnel: [w168 w171] -> w141
                tunnel: w109 -> [w167 _]
                frame False {
                }
                frame True {
                  n24 = for {
                    N: 2 -> [_]
                    tunnel: [w175] -> w172
                    shift-right: [w174] -> w171
                    shift-left: w173 -> [w178]
                    # "变频器初始化"
                    n25 = call-dynamic "Write Single Holding Register.vi"("holding register value"=u16 1142, "address"=u16 0, "Modbus master in"=w178) -> ("error out"=w175:errorcluster, "Modbus master out"=w174:refnum<class "Modbus Master.lvclass">)  [unwired: 7 in]
                  }
                  n26 = local write "变频1"(FALSE) -> ()
                }
              }
              n27 = flat-sequence {
                tunnel: w142 -> [w180]
                tunnel: [w180] -> w138
                tunnel: w141 -> [w179]
                tunnel: [w179] -> w139
                frame #0 {
                  n28 = Wait (ms)(milliseconds to wait=u32 10 ("等待时间（毫秒）")) -> ()  [unwired: 1 out]
                }
              }
              n29 = case shown="假" "加载电机左上启动" {
                tunnel: w139 -> [w156 w162]
                tunnel: [w155 w159] -> w87
                tunnel: [w151 w158] -> w89
                tunnel: w138 -> [w152 w157]
                frame False {
                  n30 = call-dynamic "Write Single Holding Register.vi"("error in (no error)"=w152, "holding register value"=u16 1143, "address"=u16 0, "Modbus master in"=w156) -> ("error out"=w151:errorcluster, "Modbus master out"=w155:refnum<class "Modbus Master.lvclass">)  [unwired: 6 in]
                }
                frame True {
                  n31 = call-dynamic "Write Single Holding Register.vi"("error in (no error)"=w157, "holding register value"=u16 1151, "address"=u16 0, "Modbus master in"=w162) -> ("error out"=w158:errorcluster, "Modbus master out"=w159:refnum<class "Modbus Master.lvclass">)  [unwired: 6 in]
                }
              }
              n32 = case shown="假" "加载电机左上正反转" {
                tunnel: [w163 w166] -> w135
                frame False {
                  n33 = local read "加载电机左上转矩给定"() -> (w163:i16)
                }
                frame True {
                  n34 = Multiply(x="加载电机左上转矩给定", y=i8 -1) -> (x*y=w166:i16)
                }
              }
              n35 = flat-sequence {
                tunnel: w89 -> [w147]
                tunnel: [w147] -> w88
                tunnel: w87 -> [w146]
                tunnel: [w146] -> _
                tunnel: [w146] -> w86
                frame #0 {
                  n36 = Wait (ms)(milliseconds to wait=u32 10 ("等待时间（毫秒）")) -> ()  [unwired: 1 out]
                }
              }
              n37 = call-dynamic "Write Single Holding Register.vi"("error in (no error)"=w88, "holding register value"=w135, "address"=u16 1, "Modbus master in"=w86) -> ("error out"=w104:errorcluster, "Modbus master out"=w105:refnum<class "Modbus Master.lvclass">)  [unwired: 6 in]
              n38 = local read "加载左上转矩监控"() -> (w69:i16)
              n39 = call-dynamic "Read Holding Registers.vi"("error in (no error)"=w104, "number of holding registers"=u16 2, "starting address"=u16 109, "Modbus master in"=w105) -> ("error out"=w108:errorcluster, "register values"=w123:u16[], "Modbus master out"=w116:refnum<class "Modbus Master.lvclass">)  [unwired: 5 in]
              n40 = Index Array(array=w123) -> (element #1=→"加载左上转矩监控":u16, element #2=w121:u16)  [unwired: 2 in]
              n41 = Divide(x=w121, y=u16 10) -> (x/y=→"加载电机左上母线电压":dbl)
              n42 = call-dynamic "Read Holding Registers.vi"("error in (no error)"=w108, "number of holding registers"=u16 1, "starting address"=u16 106, "Modbus master in"=w116) -> ("error out"=w103:errorcluster, "register values"=w115:u16[], "Modbus master out"=w90:refnum<class "Modbus Master.lvclass">)  [unwired: 5 in]
              n43 = Index Array(array=w115) -> (element #1=w114:u16)  [unwired: 2 in, 1 out]
              n44 = Multiply(x=w114, y=0.3) -> (x*y=→"加载电机左上母线电流":dbl)
              n45 = Divide(x=w69, y=u16 10000) -> (x/y=w72:dbl)
              n46 = Multiply(x=w72, y=800.0) -> (x*y=→"加载扭矩N.M(单个）":dbl)
              n47 = call-dynamic "Read Holding Registers.vi"("error in (no error)"=w103, "number of holding registers"=u16 2, "starting address"=u16 20200 ("address"), "Modbus master in"=w90) -> ("error out"=w85:errorcluster, "register values"=w132:u16[], "Modbus master out"=w98:refnum<class "Modbus Master.lvclass">)  [unwired: 5 in]
              n48 = Index Array(array=w132) -> (element #1=w129:u16, element #2=w131:u16)  [unwired: 2 in]
              n49 = Multiply(x=w131, y=u32 65536) -> (x*y=w128:u32)
              n50 = Add(x=w129, y=w128) -> (x+y=w127:u32)
              n51 = To Long Integer(number=w127) -> (32bit integer=w126:i32)
              n52 = Divide(x=w126, y=100) -> (x/y=→"加载左上转速监控" →"后左":dbl)
              n53 = call-dynamic "Read Holding Registers.vi"("error in (no error)"=w85, "number of holding registers"=u16 2, "starting address"=u16 420, "Modbus master in"=w98) -> ("error out"=w82:errorcluster, "register values"=w95:u16[], "Modbus master out"=w84:refnum<class "Modbus Master.lvclass">)  [unwired: 5 in]
              n54 = Index Array(array=w95) -> (element #1=w94:u16, element #2=w93:u16)  [unwired: 2 in]
              n55 = call-dynamic "Read Holding Registers.vi"("error in (no error)"=w82, "number of holding registers"=u16 1, "starting address"=u16 615, "Modbus master in"=w84) -> ("error out"=w81:errorcluster, "register values"=w79:u16[], "Modbus master out"=w83:refnum<class "Modbus Master.lvclass">)  [unwired: 5 in]
              n56 = Add(x=w94, y=w93) -> (x+y=w92:u16)
              n57 = Greater Than 0?(x=w92) -> (x > 0?=w91:bool)
              n58 = case shown="真" w91 {
                frame False {
                  n59 = local write "变频故障1"(FALSE ("变频故障1")) -> ()
                }
                frame True {
                  "变频故障1" <- TRUE ("变频故障1")
                }
              }
              n60 = call <vilib>:"Set Timeouts.vi"("error in (no error)"=w81, "write operation timeout (ms)"=w102, "read operation timeout (ms)"=w102, "Modbus master in"=w83) -> ("error out"=w106:errorcluster, "Modbus master out"=w111:refnum<class "Modbus Master.lvclass">)  [unwired: 6 in]
              n61 = Index Array(array=w79) -> (element=w78:u16)  [unwired: 1 in]
              n62 = Number To Boolean Array(number=w78) -> (Boolean array=w76:bool[])
              "后左" <- w76
              n63 = Index Array(array=w76, index=5 ("索引")) -> (element=→"后左":bool)
              n64 = Wait (ms)(milliseconds to wait=u32 50 ("等待时间（毫秒）")) -> ()  [unwired: 1 out]
            }
            frame 2 {
              w210 = 200 ("read operation timeout (ms)")
              n65 = local read "变频2"() -> (w249:bool)
              n66 = call <vilib>:"Set Unit ID.vi"("error in (no error)"=w220, "unit ID"=u8 2, "Modbus master in"=w221) -> ("error out"=w224:errorcluster, "Modbus master out"=w252:refnum<class "Modbus Master.lvclass">)  [unwired: 7 in]
              n67 = case shown="真" w249 {
                tunnel: w252 -> [w276 w282]
                tunnel: [w275 w279] -> w251
                tunnel: [w276 w278] -> w250
                tunnel: w224 -> [w275 _]
                frame False {
                }
                frame True {
                  # "变频器初始化"
                  n68 = call-dynamic "Write Single Holding Register.vi"("holding register value"=u16 1142, "address"=u16 0, "Modbus master in"=w282) -> ("error out"=w279:errorcluster, "Modbus master out"=w278:refnum<class "Modbus Master.lvclass">)  [unwired: 7 in]
                  n69 = local write "变频2"(FALSE) -> ()
                }
              }
              n70 = flat-sequence {
                tunnel: w251 -> [w284]
                tunnel: [w284] -> w247
                tunnel: w250 -> [w283]
                tunnel: [w283] -> w248
                frame #0 {
                  n71 = Wait (ms)(milliseconds to wait=u32 10 ("等待时间（毫秒）")) -> ()  [unwired: 1 out]
                }
              }
              n72 = case shown="假" "加载电机左下启动" {
                tunnel: w248 -> [w264 w270]
                tunnel: [w263 w267] -> w197
                tunnel: [w259 w266] -> w195
                tunnel: w247 -> [w260 w265]
                frame False {
                  n73 = call-dynamic "Write Single Holding Register.vi"("error in (no error)"=w260, "holding register value"=u16 1143, "address"=u16 0, "Modbus master in"=w264) -> ("error out"=w259:errorcluster, "Modbus master out"=w263:refnum<class "Modbus Master.lvclass">)  [unwired: 6 in]
                }
                frame True {
                  n74 = call-dynamic "Write Single Holding Register.vi"("error in (no error)"=w265, "holding register value"=u16 1151, "address"=u16 0, "Modbus master in"=w270) -> ("error out"=w266:errorcluster, "Modbus master out"=w267:refnum<class "Modbus Master.lvclass">)  [unwired: 6 in]
                }
              }
              n75 = flat-sequence {
                tunnel: w195 -> [w255]
                tunnel: [w255] -> w194
                tunnel: w197 -> [w254]
                tunnel: [w254] -> w196
                frame #0 {
                  n76 = Wait (ms)(milliseconds to wait=u32 10 ("等待时间（毫秒）")) -> ()  [unwired: 1 out]
                }
              }
              n77 = case shown="真" "加载电机左下正反转" {
                tunnel: [w271 w274] -> w245
                frame False {
                  n78 = local read "加载电机左下转矩给定"() -> (w271:i16)
                }
                frame True {
                  n79 = Multiply(x="加载电机左下转矩给定", y=i8 -1) -> (x*y=w274:i16)
                }
              }
              n80 = call-dynamic "Write Single Holding Register.vi"("error in (no error)"=w194, "holding register value"=w245, "address"=u16 1, "Modbus master in"=w196) -> ("error out"=w212:errorcluster, "Modbus master out"=w213:refnum<class "Modbus Master.lvclass">)  [unwired: 6 in]
              n81 = call-dynamic "Read Holding Registers.vi"("error in (no error)"=w212, "number of holding registers"=u16 2, "starting address"=u16 109, "Modbus master in"=w213) -> ("error out"=w223:errorcluster, "register values"=w233:u16[], "Modbus master out"=w228:refnum<class "Modbus Master.lvclass">)  [unwired: 5 in]
              n82 = Index Array(array=w233) -> (element #1=→"加载左下转矩监控":u16, element #2=w232:u16)  [unwired: 2 in]
              n83 = Divide(x=w232, y=u16 10) -> (x/y=→"加载电机左下母线电压":dbl)
              n84 = call-dynamic "Read Holding Registers.vi"("error in (no error)"=w223, "number of holding registers"=u16 1, "starting address"=u16 106, "Modbus master in"=w228) -> ("error out"=w211:errorcluster, "register values"=w227:u16[], "Modbus master out"=w198:refnum<class "Modbus Master.lvclass">)  [unwired: 5 in]
              n85 = Index Array(array=w227) -> (element #1=w226:u16)  [unwired: 2 in, 1 out]
              n86 = Multiply(x=w226, y=0.3) -> (x*y=→"加载电机左下母线电流":dbl)
              n87 = call-dynamic "Read Holding Registers.vi"("error in (no error)"=w211, "number of holding registers"=u16 2, "starting address"=u16 20200 ("address"), "Modbus master in"=w198) -> ("error out"=w193:errorcluster, "register values"=w242:u16[], "Modbus master out"=w199:refnum<class "Modbus Master.lvclass">)  [unwired: 5 in]
              n88 = Index Array(array=w242) -> (element #1=w239:u16, element #2=w241:u16)  [unwired: 2 in]
              n89 = Multiply(x=w241, y=u32 65536) -> (x*y=w238:u32)
              n90 = Add(x=w239, y=w238) -> (x+y=w237:u32)
              n91 = To Long Integer(number=w237) -> (32bit integer=w236:i32)
              n92 = Divide(x=w236, y=100) -> (x/y=→"加载左下转速监控" →"后右":dbl)
              n93 = call-dynamic "Read Holding Registers.vi"("error in (no error)"=w193, "number of holding registers"=u16 2, "starting address"=u16 420, "Modbus master in"=w199) -> ("error out"=w185:errorcluster, "register values"=w203:u16[], "Modbus master out"=w192:refnum<class "Modbus Master.lvclass">)  [unwired: 5 in]
              n94 = Index Array(array=w203) -> (element #1=w202:u16, element #2=w201:u16)  [unwired: 2 in]
              n95 = Add(x=w202, y=w201) -> (x+y=w206:u16)
              n96 = Greater Than 0?(x=w206) -> (x > 0?=w200:bool)
              n97 = case shown="真" w200 {
                frame False {
                  n98 = local write "变频故障2"(FALSE ("变频故障2")) -> ()
                }
                frame True {
                  "变频故障2" <- TRUE ("变频故障2")
                }
              }
              n99 = call-dynamic "Read Holding Registers.vi"("error in (no error)"=w185, "number of holding registers"=u16 1, "starting address"=u16 615, "Modbus master in"=w192) -> ("error out"=w188:errorcluster, "register values"=w187:u16[], "Modbus master out"=w191:refnum<class "Modbus Master.lvclass">)  [unwired: 5 in]
              n100 = Index Array(array=w187) -> (element=w186:u16)  [unwired: 1 in]
              n101 = call <vilib>:"Set Timeouts.vi"("error in (no error)"=w188, "write operation timeout (ms)"=w210, "read operation timeout (ms)"=w210, "Modbus master in"=w191) -> ("error out"=w214:errorcluster, "Modbus master out"=w219:refnum<class "Modbus Master.lvclass">)  [unwired: 6 in]
              n102 = Number To Boolean Array(number=w186) -> (Boolean array=w184:bool[])
              "后右" <- w184
              n103 = Index Array(array=w184, index=5 ("索引")) -> (element=→"后右":bool)
              n104 = Wait (ms)(milliseconds to wait=u32 50 ("等待时间（毫秒）")) -> ()  [unwired: 1 out]
            }
            frame 3 {
              w314 = 200 ("read operation timeout (ms)")
              n105 = local read "变频3"() -> (w323:bool)
              n106 = call <vilib>:"Set Unit ID.vi"("error in (no error)"=w325, "unit ID"=u8 3, "Modbus master in"=w326) -> ("error out"=w329:errorcluster, "Modbus master out"=w356:refnum<class "Modbus Master.lvclass">)  [unwired: 7 in]
              n107 = case shown="真" w323 {
                tunnel: w356 -> [w380 w385]
                tunnel: [w379 w384] -> w355
                tunnel: [w380 w383] -> w354
                tunnel: w329 -> [w379 _]
                frame False {
                }
                frame True {
                  n108 = for {
                    N: 2 -> [_]
                    tunnel: [w387] -> w384
                    shift-right: [w386] -> w383
                    shift-left: w385 -> [w390]
                    # "变频器初始化"
                    n109 = call-dynamic "Write Single Holding Register.vi"("holding register value"=u16 1142, "address"=u16 0, "Modbus master in"=w390) -> ("error out"=w387:errorcluster, "Modbus master out"=w386:refnum<class "Modbus Master.lvclass">)  [unwired: 7 in]
                  }
                  n110 = local write "变频3"(FALSE) -> ()
                }
              }
              n111 = flat-sequence {
                tunnel: w355 -> [w392]
                tunnel: [w392] -> w352
                tunnel: w354 -> [w391]
                tunnel: [w391] -> w353
                frame #0 {
                  n112 = Wait (ms)(milliseconds to wait=u32 10 ("等待时间（毫秒）")) -> ()  [unwired: 1 out]
                }
              }
              n113 = case shown="真" "加载电机右上启动" {
                tunnel: w353 -> [w368 w374]
                tunnel: [w367 w371] -> w302
                tunnel: [w363 w370] -> w300
                tunnel: w352 -> [w364 w369]
                frame False {
                  n114 = call-dynamic "Write Single Holding Register.vi"("error in (no error)"=w364, "holding register value"=u16 1143, "address"=u16 0, "Modbus master in"=w368) -> ("error out"=w363:errorcluster, "Modbus master out"=w367:refnum<class "Modbus Master.lvclass">)  [unwired: 6 in]
                }
                frame True {
                  n115 = call-dynamic "Write Single Holding Register.vi"("error in (no error)"=w369, "holding register value"=u16 1151, "address"=u16 0, "Modbus master in"=w374) -> ("error out"=w370:errorcluster, "Modbus master out"=w371:refnum<class "Modbus Master.lvclass">)  [unwired: 6 in]
                }
              }
              n116 = flat-sequence {
                tunnel: w300 -> [w359]
                tunnel: [w359] -> w299
                tunnel: w302 -> [w358]
                tunnel: [w358] -> w301
                frame #0 {
                  n117 = Wait (ms)(milliseconds to wait=u32 10 ("等待时间（毫秒）")) -> ()  [unwired: 1 out]
                }
              }
              n118 = case shown="真" "加载电机右上正反转" {
                tunnel: [w375 w378] -> w350
                frame False {
                  n119 = local read "加载电机右上转矩给定"() -> (w375:i16)
                }
                frame True {
                  n120 = Multiply(x="加载电机右上转矩给定", y=i8 -1) -> (x*y=w378:i16)
                }
              }
              n121 = call-dynamic "Write Single Holding Register.vi"("error in (no error)"=w299, "holding register value"=w350, "address"=u16 1, "Modbus master in"=w301) -> ("error out"=w316:errorcluster, "Modbus master out"=w317:refnum<class "Modbus Master.lvclass">)  [unwired: 6 in]
              n122 = call-dynamic "Read Holding Registers.vi"("error in (no error)"=w316, "number of holding registers"=u16 2, "starting address"=u16 109, "Modbus master in"=w317) -> ("error out"=w328:errorcluster, "register values"=w338:u16[], "Modbus master out"=w333:refnum<class "Modbus Master.lvclass">)  [unwired: 5 in]
              n123 = Index Array(array=w338) -> (element #1=→"加载转矩右上监控":u16, element #2=w337:u16)  [unwired: 2 in]
              n124 = Divide(x=w337, y=u16 10) -> (x/y=→"加载电机右上母线电压":dbl)
              n125 = call-dynamic "Read Holding Registers.vi"("error in (no error)"=w328, "number of holding registers"=u16 1, "starting address"=u16 106, "Modbus master in"=w333) -> ("error out"=w315:errorcluster, "register values"=w332:u16[], "Modbus master out"=w298:refnum<class "Modbus Master.lvclass">)  [unwired: 5 in]
              n126 = Index Array(array=w332) -> (element #1=w331:u16)  [unwired: 2 in, 1 out]
              n127 = Multiply(x=w331, y=0.3) -> (x*y=→"加载电机右上母线电流":dbl)
              n128 = call-dynamic "Read Holding Registers.vi"("error in (no error)"=w315, "number of holding registers"=u16 2, "starting address"=u16 20200 ("address"), "Modbus master in"=w298) -> ("error out"=w297:errorcluster, "register values"=w347:u16[], "Modbus master out"=w303:refnum<class "Modbus Master.lvclass">)  [unwired: 5 in]
              n129 = Index Array(array=w347) -> (element #1=w344:u16, element #2=w346:u16)  [unwired: 2 in]
              n130 = Multiply(x=w346, y=u32 65536) -> (x*y=w343:u32)
              n131 = Add(x=w344, y=w343) -> (x+y=w342:u32)
              n132 = To Long Integer(number=w342) -> (32bit integer=w341:i32)
              n133 = Divide(x=w341, y=100) -> (x/y=→"加载右上转速监控" →"中左":dbl)
              n134 = call-dynamic "Read Holding Registers.vi"("error in (no error)"=w297, "number of holding registers"=u16 2, "starting address"=u16 420, "Modbus master in"=w303) -> ("error out"=w294:errorcluster, "register values"=w307:u16[], "Modbus master out"=w296:refnum<class "Modbus Master.lvclass">)  [unwired: 5 in]
              n135 = Index Array(array=w307) -> (element #1=w306:u16, element #2=w305:u16)  [unwired: 2 in]
              n136 = call-dynamic "Read Holding Registers.vi"("error in (no error)"=w294, "number of holding registers"=u16 1, "starting address"=u16 615, "Modbus master in"=w296) -> ("error out"=w293:errorcluster, "register values"=w290:u16[], "Modbus master out"=w295:refnum<class "Modbus Master.lvclass">)  [unwired: 5 in]
              n137 = Wait (ms)(milliseconds to wait=u32 50 ("等待时间（毫秒）")) -> ()  [unwired: 1 out]
              n138 = Add(x=w306, y=w305) -> (x+y=w310:u16)
              n139 = Greater Than 0?(x=w310) -> (x > 0?=w304:bool)
              n140 = case shown="真" w304 {
                frame False {
                  n141 = local write "变频故障 3"(FALSE ("变频故障 3")) -> ()
                }
                frame True {
                  "变频故障 3" <- TRUE ("变频故障 3")
                }
              }
              n142 = Index Array(array=w290) -> (element=w289:u16)  [unwired: 1 in]
              n143 = Number To Boolean Array(number=w289) -> (Boolean array=w288:bool[])
              "中左" <- w288
              n144 = Index Array(array=w288, index=5 ("索引")) -> (element=→"中左":bool)
              n145 = call <vilib>:"Set Timeouts.vi"("error in (no error)"=w293, "write operation timeout (ms)"=w314, "read operation timeout (ms)"=w314, "Modbus master in"=w295) -> ("error out"=w318:errorcluster, "Modbus master out"=w324:refnum<class "Modbus Master.lvclass">)  [unwired: 6 in]
            }
            frame 4 {
              w424 = 200 ("read operation timeout (ms)")
              n146 = call <vilib>:"Set Unit ID.vi"("error in (no error)"=w433, "unit ID"=u8 4, "Modbus master in"=w434) -> ("error out"=w438:errorcluster, "Modbus master out"=w464:refnum<class "Modbus Master.lvclass">)  [unwired: 7 in]
              n147 = local read "变频4"() -> (w435:bool)
              n148 = case shown="真" w435 {
                tunnel: w464 -> [w488 w494]
                tunnel: [w487 w493] -> w463
                tunnel: [w488 w492] -> w462
                tunnel: w438 -> [w487 w490]
                frame False {
                }
                frame True {
                  n149 = for {
                    N: 2 -> [_]
                    shift-right: [w496] -> w492
                    shift-left: w494 -> [w500]
                    shift-right: [w497] -> w493
                    shift-left: w490 -> [w495]
                    # "变频器初始化"
                    n150 = call-dynamic "Write Single Holding Register.vi"("error in (no error)"=w495, "holding register value"=u16 1142, "address"=u16 0, "Modbus master in"=w500) -> ("error out"=w497:errorcluster, "Modbus master out"=w496:refnum<class "Modbus Master.lvclass">)  [unwired: 6 in]
                  }
                  n151 = local write "变频4"(FALSE) -> ()
                }
              }
              n152 = flat-sequence {
                tunnel: w463 -> [w502]
                tunnel: [w502] -> w460
                tunnel: w462 -> [w501]
                tunnel: [w501] -> w461
                frame #0 {
                  n153 = Wait (ms)(milliseconds to wait=u32 10 ("等待时间（毫秒）")) -> ()  [unwired: 1 out]
                }
              }
              n154 = case shown="假" "加载电机右下启动" {
                tunnel: w461 -> [w476 w482]
                tunnel: [w475 w479] -> w410
                tunnel: [w471 w478] -> w408
                tunnel: w460 -> [w472 w477]
                frame False {
                  n155 = call-dynamic "Write Single Holding Register.vi"("error in (no error)"=w472, "holding register value"=u16 1143, "address"=u16 0, "Modbus master in"=w476) -> ("error out"=w471:errorcluster, "Modbus master out"=w475:refnum<class "Modbus Master.lvclass">)  [unwired: 6 in]
                }
                frame True {
                  n156 = call-dynamic "Write Single Holding Register.vi"("error in (no error)"=w477, "holding register value"=u16 1151, "address"=u16 0, "Modbus master in"=w482) -> ("error out"=w478:errorcluster, "Modbus master out"=w479:refnum<class "Modbus Master.lvclass">)  [unwired: 6 in]
                }
              }
              n157 = flat-sequence {
                tunnel: w408 -> [w467]
                tunnel: [w467] -> w407
                tunnel: w410 -> [w466]
                tunnel: [w466] -> w409
                frame #0 {
                  n158 = Wait (ms)(milliseconds to wait=u32 10 ("等待时间（毫秒）")) -> ()  [unwired: 1 out]
                }
              }
              n159 = case shown="假" "加载电机右下正反转" {
                tunnel: [w483 w486] -> w394
                frame False {
                  n160 = local read "加载电机右下转矩给定"() -> (w483:i16)
                }
                frame True {
                  n161 = Multiply(x="加载电机右下转矩给定", y=i8 -1) -> (x*y=w486:i16)
                }
              }
              n162 = call-dynamic "Write Single Holding Register.vi"("error in (no error)"=w407, "holding register value"=w394, "address"=u16 1, "Modbus master in"=w409) -> ("error out"=w427:errorcluster, "Modbus master out"=w426:refnum<class "Modbus Master.lvclass">)  [unwired: 6 in]
              n163 = call-dynamic "Read Holding Registers.vi"("error in (no error)"=w427, "number of holding registers"=u16 2, "starting address"=u16 109, "Modbus master in"=w426) -> ("error out"=w437:errorcluster, "register values"=w447:u16[], "Modbus master out"=w442:refnum<class "Modbus Master.lvclass">)  [unwired: 5 in]
              n164 = Index Array(array=w447) -> (element #1=→"加载右下转矩监控":u16, element #2=w446:u16)  [unwired: 2 in]
              n165 = Divide(x=w446, y=u16 10) -> (x/y=→"加载电机右下母线电压":dbl)
              n166 = call-dynamic "Read Holding Registers.vi"("error in (no error)"=w437, "number of holding registers"=u16 1, "starting address"=u16 106, "Modbus master in"=w442) -> ("error out"=w425:errorcluster, "register values"=w441:u16[], "Modbus master out"=w411:refnum<class "Modbus Master.lvclass">)  [unwired: 5 in]
              n167 = Index Array(array=w441) -> (element #1=w440:u16)  [unwired: 2 in, 1 out]
              n168 = Multiply(x=w440, y=0.3) -> (x*y=→"加载电机右下母线电流":dbl)
              n169 = call-dynamic "Read Holding Registers.vi"("error in (no error)"=w425, "number of holding registers"=u16 2, "starting address"=u16 20200 ("address"), "Modbus master in"=w411) -> ("error out"=w406:errorcluster, "register values"=w456:u16[], "Modbus master out"=w412:refnum<class "Modbus Master.lvclass">)  [unwired: 5 in]
              n170 = Index Array(array=w456) -> (element #1=w453:u16, element #2=w455:u16)  [unwired: 2 in]
              n171 = Multiply(x=w455, y=u32 65536) -> (x*y=w452:u32)
              n172 = Add(x=w453, y=w452) -> (x+y=w451:u32)
              n173 = To Long Integer(number=w451) -> (32bit integer=w450:i32)
              n174 = Divide(x=w450, y=100) -> (x/y=→"加载转速右下监控" →"中右":dbl)
              n175 = call-dynamic "Read Holding Registers.vi"("error in (no error)"=w406, "number of holding registers"=u16 2, "starting address"=u16 420, "Modbus master in"=w412) -> ("error out"=w403:errorcluster, "register values"=w416:u16[], "Modbus master out"=w405:refnum<class "Modbus Master.lvclass">)  [unwired: 5 in]
              n176 = Wait (ms)(milliseconds to wait=u32 50 ("等待时间（毫秒）")) -> ()  [unwired: 1 out]
              n177 = call-dynamic "Read Holding Registers.vi"("error in (no error)"=w403, "number of holding registers"=u16 1, "starting address"=u16 615, "Modbus master in"=w405) -> ("error out"=w402:errorcluster, "register values"=w399:u16[], "Modbus master out"=w404:refnum<class "Modbus Master.lvclass">)  [unwired: 5 in]
              n178 = Index Array(array=w416) -> (element #1=w415:u16, element #2=w414:u16)  [unwired: 2 in]
              n179 = Add(x=w415, y=w414) -> (x+y=w419:u16)
              n180 = Greater Than 0?(x=w419) -> (x > 0?=w413:bool)
              n181 = case shown="真" w413 {
                frame False {
                  n182 = local write "变频故障 4"(FALSE ("变频故障 4")) -> ()
                }
                frame True {
                  "变频故障 4" <- TRUE ("变频故障 4")
                }
              }
              n183 = call <vilib>:"Set Timeouts.vi"("error in (no error)"=w402, "write operation timeout (ms)"=w424, "read operation timeout (ms)"=w424, "Modbus master in"=w404) -> ("error out"=w428:errorcluster, "Modbus master out"=w429:refnum<class "Modbus Master.lvclass">)  [unwired: 6 in]
              n184 = Index Array(array=w399) -> (element=w398:u16)  [unwired: 1 in]
              n185 = Number To Boolean Array(number=w398) -> (Boolean array=w397:bool[])
              "中右" <- w397
              n186 = Index Array(array=w397, index=5 ("索引")) -> (element=→"中右":bool)
            }
            frame 5 {
              w537 = 200 ("read operation timeout (ms)")
              n187 = local read "变频5"() -> (w549:bool)
              n188 = call <vilib>:"Set Unit ID.vi"("error in (no error)"=w546, "unit ID"=u8 5, "Modbus master in"=w547) -> ("error out"=w552:errorcluster, "Modbus master out"=w579:refnum<class "Modbus Master.lvclass">)  [unwired: 7 in]
              n189 = case shown="真" w549 {
                tunnel: w579 -> [w625 w631]
                tunnel: [w624 w630] -> w578
                tunnel: [w625 w629] -> w577
                tunnel: w552 -> [w624 w627]
                frame False {
                }
                frame True {
                  n190 = for {
                    N: 2 -> [_]
                    shift-right: [w633] -> w629
                    shift-left: w631 -> [w637]
                    shift-right: [w634] -> w630
                    shift-left: w627 -> [w632]
                    # "变频器初始化"
                    n191 = call-dynamic "Write Single Holding Register.vi"("error in (no error)"=w632, "holding register value"=u16 1142, "address"=u16 0, "Modbus master in"=w637) -> ("error out"=w634:errorcluster, "Modbus master out"=w633:refnum<class "Modbus Master.lvclass">)  [unwired: 6 in]
                  }
                  n192 = local write "变频5"(FALSE) -> ()
                }
              }
              n193 = flat-sequence {
                tunnel: w578 -> [w639]
                tunnel: [w639] -> w575
                tunnel: w577 -> [w638]
                tunnel: [w638] -> w576
                frame #0 {
                  n194 = Wait (ms)(milliseconds to wait=u32 10 ("等待时间（毫秒）")) -> ()  [unwired: 1 out]
                }
              }
              n195 = case shown="真" "驱动电机上启动" {
                tunnel: w576 -> [w613 w619]
                tunnel: [w612 w616] -> w524
                tunnel: [w608 w615] -> w522
                tunnel: w575 -> [w609 w614]
                frame False {
                  n196 = call-dynamic "Write Single Holding Register.vi"("error in (no error)"=w609, "holding register value"=u16 1143, "address"=u16 0, "Modbus master in"=w613) -> ("error out"=w608:errorcluster, "Modbus master out"=w612:refnum<class "Modbus Master.lvclass">)  [unwired: 6 in]
                }
                frame True {
                  n197 = call-dynamic "Write Single Holding Register.vi"("error in (no error)"=w614, "holding register value"=u16 1151, "address"=u16 0, "Modbus master in"=w619) -> ("error out"=w615:errorcluster, "Modbus master out"=w616:refnum<class "Modbus Master.lvclass">)  [unwired: 6 in]
                }
              }
              n198 = flat-sequence {
                tunnel: w522 -> [w604]
                tunnel: [w604] -> w521
                tunnel: w524 -> [w603]
                tunnel: [w603] -> w523
                frame #0 {
                  n199 = Wait (ms)(milliseconds to wait=u32 10 ("等待时间（毫秒）")) -> ()  [unwired: 1 out]
                }
              }
              n200 = case shown="假" "驱动电机上正反转" {
                tunnel: [w620 w623] -> w573
                frame False {
                  n201 = local read "驱动电机上转速给定"() -> (w620:i16)
                }
                frame True {
                  n202 = Multiply(x="驱动电机上转速给定", y=i16 -1) -> (x*y=w623:i16)
                }
              }
              n203 = call-dynamic "Write Single Holding Register.vi"("error in (no error)"=w521, "holding register value"=w573, "address"=u16 1, "Modbus master in"=w523) -> ("error out"=w539:errorcluster, "Modbus master out"=w540:refnum<class "Modbus Master.lvclass">)  [unwired: 6 in]
              n204 = call-dynamic "Read Holding Registers.vi"("error in (no error)"=w539, "number of holding registers"=u16 2, "starting address"=u16 109, "Modbus master in"=w540) -> ("error out"=w551:errorcluster, "register values"=w561:u16[], "Modbus master out"=w556:refnum<class "Modbus Master.lvclass">)  [unwired: 5 in]
              n205 = Index Array(array=w561) -> (element #1=→"驱动转矩上监控":u16, element #2=w560:u16)  [unwired: 2 in]
              n206 = Divide(x=w560, y=u16 10) -> (x/y=→"驱动电机上母线电压":dbl)
              n207 = local read "当前试验档位"() -> (w515:string)
              n208 = local read "当前试验档位"() -> (w516:string)
              n209 = local read "当前试验档位"() -> (w517:string)
              n210 = local read "当前试验档位"() -> (w518:string)
              n211 = call-dynamic "Read Holding Registers.vi"("error in (no error)"=w551, "number of holding registers"=u16 1, "starting address"=u16 106, "Modbus master in"=w556) -> ("error out"=w538:errorcluster, "register values"=w555:u16[], "Modbus master out"=w520:refnum<class "Modbus Master.lvclass">)  [unwired: 5 in]
              n212 = Index Array(array=w555) -> (element #1=w554:u16)  [unwired: 2 in, 1 out]
              n213 = Multiply(x=w554, y=0.3) -> (x*y=→"驱动电机上母线电流":dbl)
              n214 = case shown="\"D6\"" w515 {
                tunnel: [w581 w582 w583 w587] -> _
                frame "D5" {
                  n215 = local read "D4平均速度"() -> (w581:dbl)
                }
                frame "D6" {
                  n216 = local read "D4平均速度"() -> (w582:dbl)
                  n217 = local write "驱动电机上转速给定"(w582) -> ()
                }
                frame "N" {
                  n218 = local read "加载左上转速监控"() -> (w583:dbl)
                }
                frame "D1", "D2", "D3", "D4", Default {
                  n219 = local read "加载左上转速监控"() -> (w586:dbl)
                  n220 = Multiply(x=w586, y=1.0) -> (x*y=w584:dbl)
                  n221 = To Word Integer(number=w584) -> (16bit integer=w587:i16)
                }
              }
              n222 = case shown="\"D5\", \"D6 \"" w516 {
                tunnel: [w588 w592] -> _
                frame "D5", "D6 " {
                  n223 = local read "D4平均速度"() -> (w588:dbl)
                }
                frame "D1", "D2", "D3", "D4", Default {
                  n224 = local read "加载左上转速监控"() -> (w591:dbl)
                  n225 = Multiply(x=w591, y=1.0) -> (x*y=w589:dbl)
                  n226 = To Word Integer(number=w589) -> (16bit integer=w592:i16)
                }
              }
              n227 = case shown="\"D5\", \"D6 \"" w517 {
                tunnel: [w593 w597] -> _
                frame "D5", "D6 " {
                  n228 = local read "D4平均速度"() -> (w593:dbl)
                }
                frame "D1", "D2", "D3", "D4", Default {
                  n229 = local read "加载左上转速监控"() -> (w596:dbl)
                  n230 = Multiply(x=w596, y=1.0) -> (x*y=w594:dbl)
                  n231 = To Word Integer(number=w594) -> (16bit integer=w597:i16)
                }
              }
              n232 = case shown="\"D5\", \"D6 \"" w518 {
                tunnel: [w598 w602] -> w534
                frame "D5", "D6 " {
                  n233 = local read "D4平均速度"() -> (w598:dbl)
                }
                frame "D1", "D2", "D3", "D4", Default {
                  n234 = local read "加载左上转速监控"() -> (w601:dbl)
                  n235 = Multiply(x=w601, y=1.0) -> (x*y=w599:dbl)
                  n236 = To Word Integer(number=w599) -> (16bit integer=w602:i16)
                }
              }
              n237 = Wait (ms)(milliseconds to wait=u32 50 ("等待时间（毫秒）")) -> ()  [unwired: 1 out]
              n238 = call-dynamic "Read Holding Registers.vi"("error in (no error)"=w538, "number of holding registers"=u16 2, "starting address"=u16 20200 ("address"), "Modbus master in"=w520) -> ("error out"=w519:errorcluster, "register values"=w570:u16[], "Modbus master out"=w525:refnum<class "Modbus Master.lvclass">)  [unwired: 5 in]
              n239 = Index Array(array=w570) -> (element #1=w567:u16, element #2=w569:u16)  [unwired: 2 in]
              n240 = Multiply(x=w569, y=u32 65536) -> (x*y=w566:u32)
              n241 = Add(x=w567, y=w566) -> (x+y=w565:u32)
              n242 = To Long Integer(number=w565) -> (32bit integer=w564:i32)
              n243 = Divide(x=w564, y=100) -> (x/y=→"驱动上转速监控" →"前左":dbl)
              n244 = local write "驱动电机上转速给定"(w534) -> ()
              n245 = call-dynamic "Read Holding Registers.vi"("error in (no error)"=w519, "number of holding registers"=u16 2, "starting address"=u16 420, "Modbus master in"=w525) -> ("error out"=w514:errorcluster, "register values"=w529:u16[], "Modbus master out"=w513:refnum<class "Modbus Master.lvclass">)  [unwired: 5 in]
              n246 = Index Array(array=w529) -> (element #1=w528:u16, element #2=w527:u16)  [unwired: 2 in]
              n247 = call-dynamic "Read Holding Registers.vi"("error in (no error)"=w514, "number of holding registers"=u16 1, "starting address"=u16 615, "Modbus master in"=w513) -> ("error out"=w511:errorcluster, "register values"=w508:u16[], "Modbus master out"=w512:refnum<class "Modbus Master.lvclass">)  [unwired: 5 in]
              n248 = Add(x=w528, y=w527) -> (x+y=w532:u16)
              n249 = Greater Than 0?(x=w532) -> (x > 0?=w526:bool)
              n250 = case shown="真" w526 {
                frame False {
                  n251 = local write "变频故障5"(FALSE ("变频故障5")) -> ()
                }
                frame True {
                  "变频故障5" <- TRUE ("变频故障5")
                }
              }
              n252 = call <vilib>:"Set Timeouts.vi"("error in (no error)"=w511, "write operation timeout (ms)"=w537, "read operation timeout (ms)"=w537, "Modbus master in"=w512) -> ("error out"=w541:errorcluster, "Modbus master out"=w548:refnum<class "Modbus Master.lvclass">)  [unwired: 6 in]
              n253 = Index Array(array=w508) -> (element=w507:u16)  [unwired: 1 in]
              n254 = Number To Boolean Array(number=w507) -> (Boolean array=w506:bool[])
              "前左" <- w506
              n255 = Index Array(array=w506, index=5 ("索引")) -> (element=→"前左":bool)
            }
            frame 6 {
              w672 = 200 ("read operation timeout (ms)")
              n256 = local read "变频6"() -> (w715:bool)
              n257 = call <vilib>:"Set Unit ID.vi"("error in (no error)"=w682, "unit ID"=u8 6, "Modbus master in"=w683) -> ("error out"=w712:errorcluster, "Modbus master out"=w685:refnum<class "Modbus Master.lvclass">)  [unwired: 7 in]
              n258 = case shown="真" w715 {
                tunnel: w685 -> [w744 w750]
                tunnel: [w743 w749] -> w686
                tunnel: [w744 w748] -> w687
                tunnel: w712 -> [w743 w746]
                frame False {
                }
                frame True {
                  n259 = for {
                    N: 2 -> [_]
                    shift-right: [w752] -> w748
                    shift-left: w750 -> [w756]
                    shift-right: [w753] -> w749
                    shift-left: w746 -> [w751]
                    # "变频器初始化"
                    n260 = call-dynamic "Write Single Holding Register.vi"("error in (no error)"=w751, "holding register value"=u16 1142, "address"=u16 0, "Modbus master in"=w756) -> ("error out"=w753:errorcluster, "Modbus master out"=w752:refnum<class "Modbus Master.lvclass">)  [unwired: 6 in]
                  }
                  n261 = local write "变频6"(FALSE) -> ()
                }
              }
              n262 = flat-sequence {
                tunnel: w686 -> [w758]
                tunnel: [w758] -> w689
                tunnel: w687 -> [w757]
                tunnel: [w757] -> w688
                frame #0 {
                  n263 = Wait (ms)(milliseconds to wait=u32 10 ("等待时间（毫秒）")) -> ()  [unwired: 1 out]
                }
              }
              n264 = case shown="假" "驱动电机下启动" {
                tunnel: w688 -> [w732 w738]
                tunnel: [w731 w735] -> w659
                tunnel: [w727 w734] -> w657
                tunnel: w689 -> [w728 w733]
                frame False {
                  n265 = call-dynamic "Write Single Holding Register.vi"("error in (no error)"=w728, "holding register value"=u16 1143, "address"=u16 0, "Modbus master in"=w732) -> ("error out"=w727:errorcluster, "Modbus master out"=w731:refnum<class "Modbus Master.lvclass">)  [unwired: 6 in]
                }
                frame True {
                  n266 = call-dynamic "Write Single Holding Register.vi"("error in (no error)"=w733, "holding register value"=u16 1151, "address"=u16 0, "Modbus master in"=w738) -> ("error out"=w734:errorcluster, "Modbus master out"=w735:refnum<class "Modbus Master.lvclass">)  [unwired: 6 in]
                }
              }
              n267 = flat-sequence {
                tunnel: w657 -> [w723]
                tunnel: [w723] -> w656
                tunnel: w659 -> [w722]
                tunnel: [w722] -> w658
                frame #0 {
                  n268 = Wait (ms)(milliseconds to wait=u32 10 ("等待时间（毫秒）")) -> ()  [unwired: 1 out]
                }
              }
              n269 = case shown="真" "驱动电机下正反转" {
                tunnel: [w739 w742] -> w691
                frame False {
                  n270 = local read "驱动电机转速下给定"() -> (w739:i16)
                }
                frame True {
                  n271 = Multiply(x="驱动电机转速下给定", y=i8 -1) -> (x*y=w742:i16)
                }
              }
              n272 = call-dynamic "Write Single Holding Register.vi"("error in (no error)"=w656, "holding register value"=w691, "address"=u16 1, "Modbus master in"=w658) -> ("error out"=w674:errorcluster, "Modbus master out"=w675:refnum<class "Modbus Master.lvclass">)  [unwired: 6 in]
              n273 = call-dynamic "Read Holding Registers.vi"("error in (no error)"=w674, "number of holding registers"=u16 2, "starting address"=u16 109, "Modbus master in"=w675) -> ("error out"=w713:errorcluster, "register values"=w703:u16[], "Modbus master out"=w708:refnum<class "Modbus Master.lvclass">)  [unwired: 5 in]
              n274 = Index Array(array=w703) -> (element #1=→"驱动转矩下监控":u16, element #2=w704:u16)  [unwired: 2 in]
              n275 = Divide(x=w704, y=u16 10) -> (x/y=→"驱动电机下母线电压":dbl)
              n276 = local read "当前试验档位"() -> (w654:string)
              n277 = call-dynamic "Read Holding Registers.vi"("error in (no error)"=w713, "number of holding registers"=u16 1, "starting address"=u16 106, "Modbus master in"=w708) -> ("error out"=w673:errorcluster, "register values"=w709:u16[], "Modbus master out"=w660:refnum<class "Modbus Master.lvclass">)  [unwired: 5 in]
              n278 = Index Array(array=w709) -> (element #1=w710:u16)  [unwired: 2 in, 1 out]
              n279 = case shown="\"D5\", \"D6\"" w654 {
                tunnel: [w716 w717 w718] -> w653
                frame "D5", "D6" {
                  n280 = local read "D4平均速度"() -> (w716:dbl)
                }
                frame "N" {
                  n281 = local read "加载左上转速监控"() -> (w717:dbl)
                }
                frame "D1", "D2", "D3", "D4", Default {
                  n282 = local read "加载左上转速监控"() -> (w721:dbl)
                  n283 = Multiply(x=w721, y=1.0) -> (x*y=w719:dbl)
                  n284 = To Word Integer(number=w719) -> (16bit integer=w718:i16)
                }
              }
              n285 = Multiply(x=w710, y=0.3) -> (x*y=→"驱动电机下母线电流":dbl)
              n286 = local write "驱动电机转速下给定"(w653) -> ()
              n287 = call-dynamic "Read Holding Registers.vi"("error in (no error)"=w673, "number of holding registers"=u16 2, "starting address"=u16 20200 ("address"), "Modbus master in"=w660) -> ("error out"=w655:errorcluster, "register values"=w694:u16[], "Modbus master out"=w661:refnum<class "Modbus Master.lvclass">)  [unwired: 5 in]
              n288 = Index Array(array=w694) -> (element #1=w697:u16, element #2=w695:u16)  [unwired: 2 in]
              n289 = Multiply(x=w695, y=u32 65536) -> (x*y=w698:u32)
              n290 = Add(x=w697, y=w698) -> (x+y=w699:u32)
              n291 = To Long Integer(number=w699) -> (32bit integer=w700:i32)
              n292 = Divide(x=w700, y=100) -> (x/y=→"驱动转速下监控" →"前右":dbl)
              n293 = call-dynamic "Read Holding Registers.vi"("error in (no error)"=w655, "number of holding registers"=u16 2, "starting address"=u16 420, "Modbus master in"=w661) -> ("error out"=w651:errorcluster, "register values"=w665:u16[], "Modbus master out"=w652:refnum<class "Modbus Master.lvclass">)  [unwired: 5 in]
              n294 = call-dynamic "Read Holding Registers.vi"("error in (no error)"=w651, "number of holding registers"=u16 1, "starting address"=u16 615, "Modbus master in"=w652) -> ("error out"=w641:errorcluster, "register values"=w647:u16[], "Modbus master out"=w650:refnum<class "Modbus Master.lvclass">)  [unwired: 5 in]
              n295 = call <vilib>:"Set Timeouts.vi"("error in (no error)"=w641, "write operation timeout (ms)"=w672, "read operation timeout (ms)"=w672, "Modbus master in"=w650) -> ("error out"=w676:errorcluster, "Modbus master out"=w681:refnum<class "Modbus Master.lvclass">)  [unwired: 6 in]
              n296 = Wait (ms)(milliseconds to wait=u32 50 ("等待时间（毫秒）")) -> ()  [unwired: 1 out]
              n297 = Index Array(array=w665) -> (element #1=w664:u16, element #2=w663:u16)  [unwired: 2 in]
              n298 = Add(x=w664, y=w663) -> (x+y=w668:u16)
              n299 = Greater Than 0?(x=w668) -> (x > 0?=w662:bool)
              n300 = case shown="真" w662 {
                frame False {
                  n301 = local write "变频故障 6"(FALSE ("变频故障 6")) -> ()
                }
                frame True {
                  "变频故障 6" <- TRUE ("变频故障 6")
                }
              }
              n302 = Not(x=w641) -> (.not. x?=→"变频器":bool)
              n303 = Index Array(array=w647) -> (element=w646:u16)  [unwired: 1 in]
              n304 = Number To Boolean Array(number=w646) -> (Boolean array=w645:bool[])
              "前右" <- w645
              n305 = Index Array(array=w645, index=5 ("索引")) -> (element=→"前右":bool)
            }
          }
        }
        n306 = case shown="真" w50 {
          frame False {
          }
          frame True {
            "485启动给遥控器布尔" <- TRUE ("485启动给遥控器布尔")
          }
        }
        n307 = local read "停止"() -> (w59:bool)
        "数值" <- w52
      }
    }
  }
  n308 = Obtain Queue(name (unnamed)="LED" ("名称（未命名）"), element data type=0) -> (queue out=w20:refnum<queue>)  [unwired: 3 in, 2 out]
  n309 = TCP Open Connection(address="192.168.1.200" ("地址"), remote port or service name=u16 10001 ("远程端口或服务名称")) -> (connection ID=w18:refnum<k5>)  [unwired: 3 in, 1 out]
  n310 = Obtain Queue(name (unnamed)="LED" ("名称（未命名）"), element data type=0) -> (queue out=w10:refnum<queue>)  [unwired: 3 in, 2 out]
  n311 = while {
    shift-right: [w785] -> w11
    shift-left: w20 -> [w781]
    tunnel: w18 -> [w786]
    shift-right: [w783] -> _
    shift-left: dbl[] [] -> [w782]
    i -> [w760]
    stop <- w787 stop-if-true
    n312 = local read "comcnt"() -> (w763:u16)
    n313 = local read "变矩器出口温度标定"() -> (w770:dbl)
    n314 = local read "右前轮轴承温度标定"() -> (w769:dbl)
    n315 = local read "左前轮轴承温度标定"() -> (w768:dbl)
    n316 = Dequeue Element(queue=w781) -> (queue out=w767:refnum<queue>, element=w765:i32)  [unwired: 2 in, 2 out]
    n317 = Greater?(x=w763, y=u16 100) -> (0:w761:bool)
    n318 = case shown="真" w761 {
      tunnel: w767 -> [w789 w792]
      tunnel: [w789 w791] -> w766
      tunnel: w765 -> [w788 _]
      tunnel: [w788 45] -> w764
      frame False {
      }
      frame True {
        n319 = Flush Queue(queue=w792) -> (queue out=w791:refnum<queue>)  [unwired: 1 in, 2 out]
      }
    }
    n320 = Merge Signals(w770, w769, w768) -> (→"波形图表":dynamicdata)
    n321 = local read "变频故障1"() -> (w772:bool)
    n322 = local read "变频故障2"() -> (w773:bool)
    n323 = local read "变频故障 3"() -> (w774:bool)
    n324 = local read "变频故障 4"() -> (w775:bool)
    n325 = local read "变频故障5"() -> (w776:bool)
    n326 = local read "变频故障 6"() -> (w777:bool)
    n327 = Compound Arithmetic op=OR ("复合运算")(w772, w773, w774, w775, w776, w777) -> (w771:bool)
    n328 = case shown="假" w771 {
      tunnel: w764 -> [w794 _]
      tunnel: [w794 44] -> w779
      tunnel: w766 -> [w793 w797]
      tunnel: [w793 w796] -> w778
      frame False {
      }
      frame True {
        n329 = Flush Queue(queue=w797) -> (queue out=w796:refnum<queue>)  [unwired: 1 in, 2 out]
      }
    }
    n330 = case shown="43" w779 {
      tunnel: w778 -> [w805 w822 w837 w852 w876 w889 w905 w919 w944 w954 w972 w986 w1010 w1021 w1039 w1052 w1078 w1087 w1105 w1118 w1144 w1155 w1173 w1185 w1211 w1221 w1240 w1255 w1268 w1294 w1303 w1322 w1335 w1355 w1371 w1389 w1401 w1422 w1438 w1456 w1467 w1476 w1482 w1490 w1496]
      tunnel: w786 -> [w807 w823 w839 w853 w878 w890 w906 w920 w945 w956 w973 w987 w1012 w1024 w1040 w1054 w1079 w1090 w1107 w1121 w1146 w1158 w1174 w1188 w1213 w1224 w1241 w1257 w1271 w1295 w1306 w1323 w1337 w1362 w1374 w1390 w1404 w1429 w1440 w1457 w1468 w1477 w1485 w1492 w1499]
      tunnel: [w804 w821 w836 w850 w877 w888 w904 w917 w943 w953 w971 w985 w1009 w1020 w1038 w1053 w1077 w1086 w1104 w1117 w1143 w1154 w1172 w1184 w1210 w1220 w1239 w1254 w1267 w1293 w1302 w1321 w1334 w1354 w1370 w1388 w1400 w1423 w1437 w1455 w1467 w1476 w1481 w1489 w1496] -> w785
      tunnel: [dbl[] [] dbl[] [] dbl[] [] dbl[] [] w872 dbl[] [] dbl[] [] dbl[] [] w937 dbl[] [] dbl[] [] dbl[] [] w1004 dbl[] [] dbl[] [] dbl[] [] w1071 dbl[] [] dbl[] [] dbl[] [] w1138 dbl[] [] dbl[] [] dbl[] [] w1205 dbl[] [] dbl[] [] dbl[] [] dbl[] [] w1287 dbl[] [] dbl[] [] dbl[] [] w1357 dbl[] [] dbl[] [] dbl[] [] w1424 dbl[] [] dbl[] [] dbl[] [] dbl[] [] dbl[] [] w1491 dbl[] []] -> w783
      tunnel: w782 -> [_ _ _ _ w873 _ _ _ w938 _ _ _ w1005 _ _ _ w1072 _ _ _ w1139 _ _ _ w1206 _ _ _ _ w1288 _ _ _ w1358 _ _ _ w1425 _ _ _ _ _ w1491 _]
      frame 2 {
        n331 = local read "等待进车布尔"() -> (w798:bool)
        n332 = local read "遥控器按钮确认"() -> (w800:bool)
        n333 = case shown="真" w798 {
          tunnel: w807 -> [_ w812]
          frame False {
          }
          frame True {
            w808 = "等待进车"
            n334 = local write "等待进车布尔"(FALSE ("等待进车布尔")) -> ()
            n335 = call "led显示更新字符串山推.vi"("显示字符"=w808, "立显/保存"=TRUE) -> ("发送数据"=w811:string)  [unwired: 9 in]
            n336 = local write "LED屏幕信息"(w808) -> ()
            n337 = call "led发送数据并接收返回山推.vi"("发送数据"=w811, "TCP网络连接输入"=w812) -> ()  [unwired: 8 in, 2 out]
          }
        }
        n338 = call <vilib>:"Boolean Crossing PtByPt.vi"("direction"=enum16{"either", "false-true", "true-false"}."false-true", "input"=w800) -> ("crossing"=w801:bool)  [unwired: 1 in]
        n339 = case shown="假" w801 {
          tunnel: [2 3] -> w806
          frame False {
          }
          frame True {
          }
        }
        n340 = Enqueue Element(queue=w805, element=w806) -> (queue out=w804:refnum<queue>)  [unwired: 2 in, 2 out]
        "字符布尔" <- TRUE ("字符布尔")
      }
      frame 3 {
        n341 = local read "遥控器按钮确认"() -> (w816:bool)
        n342 = local read "字符布尔"() -> (w815:bool)
        n343 = case shown="真" w815 {
          tunnel: w823 -> [_ w828]
          frame False {
          }
          frame True {
            w824 = "请落下举升，油缸浮动，车辆系固，连接传感器"
            n344 = local write "字符布尔"(FALSE ("字符布尔")) -> ()
            n345 = call "led显示更新字符串山推.vi"("显示字符"=w824, "立显/保存"=TRUE) -> ("发送数据"=w827:string)  [unwired: 9 in]
            n346 = call "led发送数据并接收返回山推.vi"("发送数据"=w827, "TCP网络连接输入"=w828) -> ()  [unwired: 8 in, 2 out]
            n347 = local write "LED屏幕信息"(w824) -> ()
          }
        }
        n348 = call <vilib>:"Boolean Crossing PtByPt.vi"("direction"=enum16{"either", "false-true", "true-false"}."false-true", "input"=w816) -> ("crossing"=w817:bool)  [unwired: 1 in]
        n349 = case shown="真" w817 {
          tunnel: [3 4] -> w820
          frame False {
          }
          frame True {
          }
        }
        n350 = Enqueue Element(queue=w822, element=w820) -> (queue out=w821:refnum<queue>)  [unwired: 2 in, 2 out]
      }
      frame 4 {
        # "here need it to be true"
        n351 = local read "遥控器按钮确认"() -> (w832:bool)
        n352 = local read "字符布尔"() -> (w831:bool)
        n353 = call <vilib>:"Boolean Crossing PtByPt.vi"("direction"=enum16{"either", "false-true", "true-false"}."false-true", "input"=w832) -> ("crossing"=w833:bool)  [unwired: 1 in]
        n354 = case shown="假" w831 {
          tunnel: w839 -> [w844 _]
          frame False {
            w840 = "车挂一档，转速在2000转"
            n355 = local write "字符布尔"(TRUE ("字符布尔")) -> ()
            n356 = call "led显示更新字符串山推.vi"("显示字符"=w840, "立显/保存"=TRUE) -> ("发送数据"=w843:string)  [unwired: 9 in]
            n357 = local write "LED屏幕信息"(w840) -> ()
            n358 = call "led发送数据并接收返回山推.vi"("发送数据"=w843, "TCP网络连接输入"=w844) -> ()  [unwired: 8 in, 2 out]
          }
          frame True {
          }
        }
        n359 = case shown="真" w833 {
          tunnel: [4 5] -> w838
          frame False {
          }
          frame True {
          }
        }
        n360 = Enqueue Element(queue=w837, element=w838) -> (queue out=w836:refnum<queue>)  [unwired: 2 in, 2 out]
      }
      frame 5 {
        n361 = local read "当前试验档位"() -> (w849:string)
        n362 = local read "字符布尔"() -> (w847:bool)
        n363 = case shown="\"假\", 默认" w849 {
          tunnel: [5 6] -> w851
          frame "假", Default {
          }
          frame "D1" {
          }
        }
        n364 = case shown="真" w847 {
          tunnel: w853 -> [_ w856]
          frame False {
          }
          frame True {
            w854 = "遥控器请选择D1档"
            n365 = local write "字符布尔"(FALSE ("字符布尔")) -> ()
            n366 = call "led显示更新字符串山推.vi"("显示字符"=w854, "立显/保存"=TRUE) -> ("发送数据"=w858:string)  [unwired: 9 in]
            n367 = call "led发送数据并接收返回山推.vi"("发送数据"=w858, "TCP网络连接输入"=w856) -> ()  [unwired: 8 in, 2 out]
            n368 = local write "LED屏幕信息"(w854) -> ()
          }
        }
        n369 = Enqueue Element(queue=w852, element=w851) -> (queue out=w850:refnum<queue>)  [unwired: 2 in, 2 out]
      }
      frame 6 {
        n370 = local read "D1S"() -> (w863:dbl)
        n371 = local write "字符布尔"(TRUE ("字符布尔")) -> ()
        n372 = call "已用时间"("Time Target (s)"=w863, "Reset"="Reset") -> ("Time has Elapsed"=w869:bool, "Elapsed Time Text"=w867:string)  [unwired: 10 in, 6 out]
        n373 = local read "加载左上转速监控"() -> (w874:dbl)
        n374 = call "输出文本.vi"("当前档位"="D1" ("字符串"), "字符串"=w867) -> ("输出文本"=w862:string)  [unwired: 9 in]
        n375 = local write "Reset"(FALSE ("Reset")) -> ()
        n376 = call "led显示更新字符串山推.vi"("显示字符"=w862, "立显/保存"=FALSE) -> ("发送数据"=w880:string)  [unwired: 9 in]
        n377 = local write "LED屏幕信息"(w862) -> ()
        n378 = case shown="真" w869 {
          tunnel: [6 7] -> w875
          frame False {
          }
          frame True {
            n379 = local write "Reset"(TRUE ("Reset")) -> ()
          }
        }
        n380 = call "led发送数据并接收返回山推.vi"("发送数据"=w880, "TCP网络连接输入"=w878) -> ()  [unwired: 8 in, 2 out]
        n381 = Build Array (concatenate)(w873, w874) -> (w872:dbl[])
        n382 = Array Size(array=w872) -> (size(s)=w861:i32)
        n383 = Add Array Elements(numeric array=w872) -> (sum=w871:dbl)
        n384 = Divide(x=w871, y=w861) -> (x/y=→"D1平均速度":dbl)
        n385 = Enqueue Element(queue=w876, element=w875) -> (queue out=w877:refnum<queue>)  [unwired: 2 in, 2 out]
      }
      frame 7 {
        n386 = local read "字符布尔"() -> (w884:bool)
        n387 = local read "当前试验档位"() -> (w885:string)
        n388 = case shown="真" w884 {
          tunnel: w890 -> [_ w893]
          frame False {
          }
          frame True {
            w891 = "遥控器请挂空挡" ("显示字符")
            n389 = local write "字符布尔"(FALSE ("字符布尔 2")) -> ()
            n390 = call "led显示更新字符串山推.vi"("显示字符"=w891, "立显/保存"=TRUE) -> ("发送数据"=w895:string)  [unwired: 9 in]
            n391 = local write "LED屏幕信息"(w891) -> ()
            n392 = call "led发送数据并接收返回山推.vi"("发送数据"=w895, "TCP网络连接输入"=w893) -> ()  [unwired: 8 in, 2 out]
          }
        }
        n393 = case shown="\"假\", 默认" w885 {
          tunnel: [7 8] -> w887
          frame "假", Default {
          }
          frame "N" {
          }
        }
        n394 = Enqueue Element(queue=w889, element=w887) -> (queue out=w888:refnum<queue>)  [unwired: 2 in, 2 out]
      }
      frame 8 {
        n395 = local read "字符布尔"() -> (w898:bool)
        n396 = local read "遥控器按钮确认"() -> (w901:bool)
        n397 = case shown="假" w898 {
          tunnel: w906 -> [w909 _]
          frame False {
            w907 = "请车挂二档，转速在2000转"
            n398 = local write "字符布尔"(TRUE ("字符布尔")) -> ()
            n399 = call "led显示更新字符串山推.vi"("显示字符"=w907, "立显/保存"=TRUE) -> ("发送数据"=w911:string)  [unwired: 9 in]
            n400 = local write "LED屏幕信息"(w907) -> ()
            n401 = call "led发送数据并接收返回山推.vi"("发送数据"=w911, "TCP网络连接输入"=w909) -> ()  [unwired: 8 in, 2 out]
          }
          frame True {
          }
        }
        n402 = call <vilib>:"Boolean Crossing PtByPt.vi"("direction"=enum16{"either", "false-true", "true-false"}."false-true", "input"=w901) -> ("crossing"=w900:bool)  [unwired: 1 in]
        n403 = case shown="假" w900 {
          tunnel: [8 9] -> w899
          frame False {
          }
          frame True {
          }
        }
        n404 = Enqueue Element(queue=w905, element=w899) -> (queue out=w904:refnum<queue>)  [unwired: 2 in, 2 out]
      }
      frame 9 {
        n405 = local read "字符布尔"() -> (w914:bool)
        n406 = local read "当前试验档位"() -> (w916:string)
        n407 = case shown="真" w914 {
          tunnel: w920 -> [_ w923]
          frame False {
          }
          frame True {
            w921 = "请将遥控器挂D2档"
            n408 = local write "LED屏幕信息"(w921) -> ()
            n409 = call "led显示更新字符串山推.vi"("显示字符"=w921, "立显/保存"=TRUE) -> ("发送数据"=w925:string)  [unwired: 9 in]
            n410 = local write "字符布尔"(FALSE ("字符布尔")) -> ()
            n411 = call "led发送数据并接收返回山推.vi"("发送数据"=w925, "TCP网络连接输入"=w923) -> ()  [unwired: 8 in, 2 out]
          }
        }
        n412 = case shown="\"假\", 默认" w916 {
          tunnel: [9 10] -> w918
          frame "假", Default {
          }
          frame "D2" {
          }
        }
        n413 = Enqueue Element(queue=w919, element=w918) -> (queue out=w917:refnum<queue>)  [unwired: 2 in, 2 out]
      }
      frame 10 {
        n414 = local read "D2S"() -> (w930:dbl)
        n415 = call "已用时间2"("Time Target (s)"=w930, "Reset"="Reset 2") -> ("Time has Elapsed"=w934:bool, "Elapsed Time Text"=w935:string)  [unwired: 10 in, 6 out]
        n416 = local read "加载左上转速监控"() -> (w941:dbl)
        n417 = call "输出文本.vi"("当前档位"="D2" ("字符串"), "字符串"=w935) -> ("输出文本"=w929:string)  [unwired: 9 in]
        n418 = local write "Reset 2"(FALSE ("Reset 2")) -> ()
        n419 = local write "字符布尔"(TRUE ("字符布尔")) -> ()
        n420 = case shown="真" w934 {
          tunnel: [10 11] -> w942
          frame False {
          }
          frame True {
            n421 = local write "Reset 2"(TRUE ("Reset 2")) -> ()
          }
        }
        n422 = Build Array (concatenate)(w938, w941) -> (w937:dbl[])
        n423 = Array Size(array=w937) -> (size(s)=w928:i32)
        n424 = Add Array Elements(numeric array=w937) -> (sum=w940:dbl)
        n425 = call "led显示更新字符串山推.vi"("显示字符"=w929, "立显/保存"=FALSE) -> ("发送数据"=w947:string)  [unwired: 9 in]
        n426 = local write "LED屏幕信息"(w929) -> ()
        n427 = call "led发送数据并接收返回山推.vi"("发送数据"=w947, "TCP网络连接输入"=w945) -> ()  [unwired: 8 in, 2 out]
        n428 = Divide(x=w940, y=w928) -> (x/y=→"D2平均速度":dbl)
        n429 = Enqueue Element(queue=w944, element=w942) -> (queue out=w943:refnum<queue>)  [unwired: 2 in, 2 out]
      }
      frame 11 {
        n430 = local read "当前试验档位"() -> (w955:string)
        n431 = local read "字符布尔"() -> (w951:bool)
        n432 = case shown="真" w951 {
          tunnel: w956 -> [_ w960]
          frame False {
          }
          frame True {
            w958 = "遥控器挂空挡"
            n433 = local write "字符布尔"(FALSE ("字符布尔")) -> ()
            n434 = local write "LED屏幕信息"(w958) -> ()
            n435 = call "led显示更新字符串山推.vi"("显示字符"=w958, "立显/保存"=TRUE) -> ("发送数据"=w962:string)  [unwired: 9 in]
            n436 = call "led发送数据并接收返回山推.vi"("发送数据"=w962, "TCP网络连接输入"=w960) -> ()  [unwired: 8 in, 2 out]
          }
        }
        n437 = case shown="\"N\"" w955 {
          tunnel: [11 12] -> w952
          frame "假", Default {
          }
          frame "N" {
          }
        }
        n438 = Enqueue Element(queue=w954, element=w952) -> (queue out=w953:refnum<queue>)  [unwired: 2 in, 2 out]
      }
      frame 12 {
        n439 = local read "遥控器按钮确认"() -> (w967:bool)
        n440 = local read "字符布尔"() -> (w965:bool)
        n441 = case shown="假" w965 {
          tunnel: w973 -> [w976 _]
          frame False {
            w974 = "请车挂三档，转速在2000转"
            n442 = local write "字符布尔"(TRUE ("字符布尔")) -> ()
            n443 = call "led显示更新字符串山推.vi"("显示字符"=w974, "立显/保存"=TRUE) -> ("发送数据"=w978:string)  [unwired: 9 in]
            n444 = local write "LED屏幕信息"(w974) -> ()
            n445 = call "led发送数据并接收返回山推.vi"("发送数据"=w978, "TCP网络连接输入"=w976) -> ()  [unwired: 8 in, 2 out]
          }
          frame True {
          }
        }
        n446 = call <vilib>:"Boolean Crossing PtByPt.vi"("direction"=enum16{"either", "false-true", "true-false"}."false-true", "input"=w967) -> ("crossing"=w966:bool)  [unwired: 1 in]
        n447 = case shown="假" w966 {
          tunnel: [12 13] -> w970
          frame False {
          }
          frame True {
          }
        }
        n448 = Enqueue Element(queue=w972, element=w970) -> (queue out=w971:refnum<queue>)  [unwired: 2 in, 2 out]
      }
      frame 13 {
        n449 = local read "当前试验档位"() -> (w983:string)
        n450 = local read "字符布尔"() -> (w981:bool)
        n451 = case shown="\"D3\"" w983 {
          tunnel: [13 14] -> w984
          frame "假", Default {
          }
          frame "D3" {
          }
        }
        n452 = case shown="真" w981 {
          tunnel: w987 -> [_ w990]
          frame False {
          }
          frame True {
            w988 = "遥控器挂三档"
            n453 = local write "字符布尔"(FALSE ("字符布尔")) -> ()
            n454 = local write "LED屏幕信息"(w988) -> ()
            n455 = call "led显示更新字符串山推.vi"("显示字符"=w988, "立显/保存"=TRUE) -> ("发送数据"=w992:string)  [unwired: 9 in]
            n456 = call "led发送数据并接收返回山推.vi"("发送数据"=w992, "TCP网络连接输入"=w990) -> ()  [unwired: 8 in, 2 out]
          }
        }
        n457 = Enqueue Element(queue=w986, element=w984) -> (queue out=w985:refnum<queue>)  [unwired: 2 in, 2 out]
      }
      frame 14 {
        n458 = local read "D3S"() -> (w997:dbl)
        n459 = local write "字符布尔"(TRUE ("字符布尔")) -> ()
        n460 = call "已用时间3"("Time Target (s)"=w997, "Reset"="Reset 3") -> ("Time has Elapsed"=w1001:bool, "Elapsed Time Text"=w1002:string)  [unwired: 10 in, 6 out]
        n461 = local write "Reset 3"(FALSE ("Reset 3")) -> ()
        n462 = local read "加载左上转速监控"() -> (w1008:dbl)
        n463 = call "输出文本.vi"("当前档位"="D3" ("字符串"), "字符串"=w1002) -> ("输出文本"=w996:string)  [unwired: 9 in]
        n464 = case shown="真" w1001 {
          tunnel: [14 15] -> w1011
          frame False {
          }
          frame True {
            n465 = local write "Reset 3"(TRUE ("Reset 3")) -> ()
          }
        }
        n466 = Build Array (concatenate)(w1005, w1008) -> (w1004:dbl[])
        n467 = Array Size(array=w1004) -> (size(s)=w995:i32)
        n468 = Add Array Elements(numeric array=w1004) -> (sum=w1007:dbl)
        n469 = call "led显示更新字符串山推.vi"("显示字符"=w996, "立显/保存"=FALSE) -> ("发送数据"=w1014:string)  [unwired: 9 in]
        n470 = local write "LED屏幕信息"(w996) -> ()
        n471 = call "led发送数据并接收返回山推.vi"("发送数据"=w1014, "TCP网络连接输入"=w1012) -> ()  [unwired: 8 in, 2 out]
        n472 = Divide(x=w1007, y=w995) -> (x/y=→"D3平均速度":dbl)
        n473 = Enqueue Element(queue=w1010, element=w1011) -> (queue out=w1009:refnum<queue>)  [unwired: 2 in, 2 out]
      }
      frame 15 {
        n474 = local read "当前试验档位"() -> (w1023:string)
        n475 = local read "字符布尔"() -> (w1018:bool)
        n476 = case shown="\"N\"" w1023 {
          tunnel: [15 16] -> w1022
          frame "假", Default {
          }
          frame "N" {
          }
        }
        n477 = case shown="真" w1018 {
          tunnel: w1024 -> [_ w1027]
          frame False {
          }
          frame True {
            w1025 = "遥控器挂空挡"
            n478 = local write "LED屏幕信息"(w1025) -> ()
            n479 = local write "字符布尔"(FALSE ("字符布尔")) -> ()
            n480 = call "led显示更新字符串山推.vi"("显示字符"=w1025, "立显/保存"=TRUE) -> ("发送数据"=w1029:string)  [unwired: 9 in]
            n481 = call "led发送数据并接收返回山推.vi"("发送数据"=w1029, "TCP网络连接输入"=w1027) -> ()  [unwired: 8 in, 2 out]
          }
        }
        n482 = Enqueue Element(queue=w1021, element=w1022) -> (queue out=w1020:refnum<queue>)  [unwired: 2 in, 2 out]
      }
      frame 16 {
        n483 = local read "遥控器按钮确认"() -> (w1034:bool)
        n484 = local read "字符布尔"() -> (w1032:bool)
        n485 = case shown="假" w1032 {
          tunnel: w1040 -> [w1043 _]
          frame False {
            w1041 = "车挂四档，转速在2000转"
            n486 = local write "字符布尔"(TRUE ("字符布尔")) -> ()
            n487 = local write "LED屏幕信息"(w1041) -> ()
            n488 = call "led显示更新字符串山推.vi"("显示字符"=w1041, "立显/保存"=TRUE) -> ("发送数据"=w1045:string)  [unwired: 9 in]
            n489 = call "led发送数据并接收返回山推.vi"("发送数据"=w1045, "TCP网络连接输入"=w1043) -> ()  [unwired: 8 in, 2 out]
          }
          frame True {
          }
        }
        n490 = call <vilib>:"Boolean Crossing PtByPt.vi"("direction"=enum16{"either", "false-true", "true-false"}."false-true", "input"=w1034) -> ("crossing"=w1033:bool)  [unwired: 1 in]
        n491 = case shown="真" w1033 {
          tunnel: [16 17] -> w1037
          frame False {
          }
          frame True {
          }
        }
        n492 = Enqueue Element(queue=w1039, element=w1037) -> (queue out=w1038:refnum<queue>)  [unwired: 2 in, 2 out]
      }
      frame 17 {
        n493 = local read "当前试验档位"() -> (w1050:string)
        n494 = local read "字符布尔"() -> (w1048:bool)
        n495 = case shown="\"D4\"" w1050 {
          tunnel: [17 ("等待时间（毫秒）") 18 ("等待时间（毫秒）")] -> w1051
          frame "假", Default {
          }
          frame "D4" {
          }
        }
        n496 = case shown="真" w1048 {
          tunnel: w1054 -> [_ w1057]
          frame False {
          }
          frame True {
            w1055 = "遥控器挂D4档"
            n497 = local write "LED屏幕信息"(w1055) -> ()
            n498 = local write "字符布尔"(FALSE ("字符布尔")) -> ()
            n499 = call "led显示更新字符串山推.vi"("显示字符"=w1055, "立显/保存"=TRUE) -> ("发送数据"=w1059:string)  [unwired: 9 in]
            n500 = call "led发送数据并接收返回山推.vi"("发送数据"=w1059, "TCP网络连接输入"=w1057) -> ()  [unwired: 8 in, 2 out]
          }
        }
        n501 = Enqueue Element(queue=w1052, element=w1051) -> (queue out=w1053:refnum<queue>)  [unwired: 2 in, 2 out]
      }
      frame 18 {
        n502 = local read "D4S"() -> (w1064:dbl)
        n503 = local write "字符布尔"(TRUE ("字符布尔")) -> ()
        n504 = call "已用时间4"("Time Target (s)"=w1064, "Reset"="Reset 4") -> ("Time has Elapsed"=w1068:bool, "Elapsed Time Text"=w1069:string)  [unwired: 10 in, 6 out]
        n505 = call "输出文本.vi"("当前档位"="D4" ("字符串"), "字符串"=w1069) -> ("输出文本"=w1063:string)  [unwired: 9 in]
        n506 = local write "Reset 4"(FALSE ("Reset 4")) -> ()
        n507 = local read "加载左上转速监控"() -> (w1075:dbl)
        n508 = case shown="真" w1068 {
          tunnel: [18 19] -> w1076
          frame False {
          }
          frame True {
            n509 = local write "Reset 4"(TRUE ("Reset 4")) -> ()
          }
        }
        n510 = Build Array (concatenate)(w1072, w1075) -> (w1071:dbl[])
        n511 = Array Size(array=w1071) -> (size(s)=w1062:i32)
        n512 = Add Array Elements(numeric array=w1071) -> (sum=w1074:dbl)
        n513 = call "led显示更新字符串山推.vi"("显示字符"=w1063, "立显/保存"=FALSE) -> ("发送数据"=w1081:string)  [unwired: 9 in]
        n514 = local write "LED屏幕信息"(w1063) -> ()
        n515 = Divide(x=w1074, y=w1062) -> (x/y=→"D4平均速度":dbl)
        n516 = call "led发送数据并接收返回山推.vi"("发送数据"=w1081, "TCP网络连接输入"=w1079) -> ()  [unwired: 8 in, 2 out]
        n517 = Enqueue Element(queue=w1078, element=w1076) -> (queue out=w1077:refnum<queue>)  [unwired: 2 in, 2 out]
      }
      frame 19 {
        n518 = local read "当前试验档位"() -> (w1089:string)
        n519 = local read "字符布尔"() -> (w1085:bool)
        n520 = case shown="\"N\"" w1089 {
          tunnel: [19 20] -> w1088
          frame "假", Default {
          }
          frame "N" {
          }
        }
        n521 = case shown="真" w1085 {
          tunnel: w1090 -> [_ w1094]
          frame False {
          }
          frame True {
            w1092 = "遥控器挂空挡"
            n522 = local write "LED屏幕信息"(w1092) -> ()
            n523 = call "led显示更新字符串山推.vi"("显示字符"=w1092, "立显/保存"=TRUE) -> ("发送数据"=w1096:string)  [unwired: 9 in]
            n524 = local write "字符布尔"(FALSE ("字符布尔")) -> ()
            n525 = call "led发送数据并接收返回山推.vi"("发送数据"=w1096, "TCP网络连接输入"=w1094) -> ()  [unwired: 8 in, 2 out]
          }
        }
        n526 = Enqueue Element(queue=w1087, element=w1088) -> (queue out=w1086:refnum<queue>)  [unwired: 2 in, 2 out]
      }
      frame 20 {
        n527 = local read "遥控器按钮确认"() -> (w1101:bool)
        n528 = local read "字符布尔"() -> (w1099:bool)
        n529 = case shown="假" w1099 {
          tunnel: w1107 -> [w1110 _]
          frame False {
            w1108 = "车挂五档，转速在2000转"
            n530 = local write "字符布尔"(TRUE ("字符布尔")) -> ()
            n531 = local write "LED屏幕信息"(w1108) -> ()
            n532 = call "led显示更新字符串山推.vi"("显示字符"=w1108, "立显/保存"=TRUE) -> ("发送数据"=w1112:string)  [unwired: 9 in]
            n533 = call "led发送数据并接收返回山推.vi"("发送数据"=w1112, "TCP网络连接输入"=w1110) -> ()  [unwired: 8 in, 2 out]
          }
          frame True {
          }
        }
        n534 = call <vilib>:"Boolean Crossing PtByPt.vi"("direction"=enum16{"either", "false-true", "true-false"}."false-true", "input"=w1101) -> ("crossing"=w1100:bool)  [unwired: 1 in]
        n535 = case shown="真" w1100 {
          tunnel: [20 21] -> w1106
          frame False {
          }
          frame True {
          }
        }
        n536 = Enqueue Element(queue=w1105, element=w1106) -> (queue out=w1104:refnum<queue>)  [unwired: 2 in, 2 out]
      }
      frame 21 {
        n537 = local read "当前试验档位"() -> (w1120:string)
        n538 = local read "字符布尔"() -> (w1115:bool)
        n539 = case shown="真" w1115 {
          tunnel: w1121 -> [_ w1124]
          frame False {
          }
          frame True {
            w1122 = "遥控器挂D5档"
            n540 = local write "字符布尔"(FALSE ("字符布尔")) -> ()
            n541 = call "led显示更新字符串山推.vi"("显示字符"=w1122, "立显/保存"=TRUE) -> ("发送数据"=w1126:string)  [unwired: 9 in]
            n542 = local write "LED屏幕信息"(w1122) -> ()
            n543 = call "led发送数据并接收返回山推.vi"("发送数据"=w1126, "TCP网络连接输入"=w1124) -> ()  [unwired: 8 in, 2 out]
          }
        }
        n544 = case shown="\"D5\"" w1120 {
          tunnel: [21 22] -> w1119
          frame "假", Default {
          }
          frame "D5" {
          }
        }
        n545 = Enqueue Element(queue=w1118, element=w1119) -> (queue out=w1117:refnum<queue>)  [unwired: 2 in, 2 out]
      }
      frame 22 {
        n546 = local read "D5S"() -> (w1131:dbl)
        n547 = call "已用时间5"("Time Target (s)"=w1131, "Reset"="Reset 5") -> ("Time has Elapsed"=w1135:bool, "Elapsed Time Text"=w1136:string)  [unwired: 10 in, 6 out]
        n548 = call "输出文本.vi"("当前档位"="D5" ("字符串"), "字符串"=w1136) -> ("输出文本"=w1130:string)  [unwired: 9 in]
        n549 = local read "加载左上转速监控"() -> (w1142:dbl)
        n550 = local write "字符布尔"(TRUE ("字符布尔")) -> ()
        n551 = local write "Reset 5"(FALSE ("Reset 5")) -> ()
        n552 = case shown="真" w1135 {
          tunnel: [22 23] -> w1145
          frame False {
          }
          frame True {
            n553 = local write "Reset 5"(TRUE ("Reset 5")) -> ()
          }
        }
        n554 = Build Array (concatenate)(w1139, w1142) -> (w1138:dbl[])
        n555 = Array Size(array=w1138) -> (size(s)=w1129:i32)
        n556 = call "led显示更新字符串山推.vi"("显示字符"=w1130, "立显/保存"=FALSE) -> ("发送数据"=w1148:string)  [unwired: 9 in]
        n557 = Add Array Elements(numeric array=w1138) -> (sum=w1141:dbl)
        n558 = call "led发送数据并接收返回山推.vi"("发送数据"=w1148, "TCP网络连接输入"=w1146) -> ()  [unwired: 8 in, 2 out]
        n559 = Divide(x=w1141, y=w1129) -> (x/y=→"D5平均速度":dbl)
        n560 = local write "LED屏幕信息"(w1130) -> ()
        n561 = Enqueue Element(queue=w1144, element=w1145) -> (queue out=w1143:refnum<queue>)  [unwired: 2 in, 2 out]
      }
      frame 23 {
        n562 = local read "当前试验档位"() -> (w1156:string)
        n563 = local read "字符布尔"() -> (w1152:bool)
        n564 = case shown="\"N\"" w1156 {
          tunnel: [23 24] -> w1153
          frame "假", Default {
          }
          frame "N" {
          }
        }
        n565 = case shown="真" w1152 {
          tunnel: w1158 -> [_ w1161]
          frame False {
          }
          frame True {
            w1159 = "遥控器挂空挡"
            n566 = local write "LED屏幕信息"(w1159) -> ()
            n567 = call "led显示更新字符串山推.vi"("显示字符"=w1159, "立显/保存"=TRUE) -> ("发送数据"=w1163:string)  [unwired: 9 in]
            n568 = call "led发送数据并接收返回山推.vi"("发送数据"=w1163, "TCP网络连接输入"=w1161) -> ()  [unwired: 8 in, 2 out]
            n569 = local write "字符布尔"(FALSE ("字符布尔")) -> ()
          }
        }
        n570 = Enqueue Element(queue=w1155, element=w1153) -> (queue out=w1154:refnum<queue>)  [unwired: 2 in, 2 out]
      }
      frame 24 {
        n571 = local read "遥控器按钮确认"() -> (w1168:bool)
        n572 = local read "字符布尔"() -> (w1166:bool)
        n573 = case shown="假" w1166 {
          tunnel: w1174 -> [w1177 _]
          frame False {
            w1175 = "车挂六档，转速在2000转"
            n574 = local write "字符布尔"(TRUE ("字符布尔")) -> ()
            n575 = local write "LED屏幕信息"(w1175) -> ()
            n576 = call "led显示更新字符串山推.vi"("显示字符"=w1175, "立显/保存"=TRUE) -> ("发送数据"=w1179:string)  [unwired: 9 in]
            n577 = call "led发送数据并接收返回山推.vi"("发送数据"=w1179, "TCP网络连接输入"=w1177) -> ()  [unwired: 8 in, 2 out]
          }
          frame True {
          }
        }
        n578 = call <vilib>:"Boolean Crossing PtByPt.vi"("direction"=enum16{"either", "false-true", "true-false"}."false-true", "input"=w1168) -> ("crossing"=w1167:bool)  [unwired: 1 in]
        n579 = case shown="假" w1167 {
          tunnel: [24 25] -> w1171
          frame False {
          }
          frame True {
          }
        }
        n580 = Enqueue Element(queue=w1173, element=w1171) -> (queue out=w1172:refnum<queue>)  [unwired: 2 in, 2 out]
      }
      frame 25 {
        n581 = local read "当前试验档位"() -> (w1187:string)
        n582 = local read "字符布尔"() -> (w1182:bool)
        n583 = case shown="\"D6\"" w1187 {
          tunnel: [25 26] -> w1186
          frame "假", Default {
          }
          frame "D6" {
          }
        }
        n584 = case shown="真" w1182 {
          tunnel: w1188 -> [_ w1191]
          frame False {
          }
          frame True {
            w1189 = "遥控器挂D6档"
            n585 = local write "字符布尔"(FALSE ("字符布尔")) -> ()
            n586 = call "led显示更新字符串山推.vi"("显示字符"=w1189, "立显/保存"=TRUE) -> ("发送数据"=w1193:string)  [unwired: 9 in]
            n587 = local write "LED屏幕信息"(w1189) -> ()
            n588 = call "led发送数据并接收返回山推.vi"("发送数据"=w1193, "TCP网络连接输入"=w1191) -> ()  [unwired: 8 in, 2 out]
          }
        }
        n589 = Enqueue Element(queue=w1185, element=w1186) -> (queue out=w1184:refnum<queue>)  [unwired: 2 in, 2 out]
      }
      frame 26 {
        n590 = local read "D6S"() -> (w1198:dbl)
        n591 = call "已用时间6"("Time Target (s)"=w1198, "Reset"="Reset 6") -> ("Time has Elapsed"=w1202:bool, "Elapsed Time Text"=w1203:string)  [unwired: 10 in, 6 out]
        n592 = local read "加载左上转速监控"() -> (w1209:dbl)
        n593 = call "输出文本.vi"("当前档位"="D6" ("字符串"), "字符串"=w1203) -> ("输出文本"=w1197:string)  [unwired: 9 in]
        n594 = local write "字符布尔"(TRUE ("字符布尔")) -> ()
        n595 = local write "Reset 6"(FALSE ("Reset 6")) -> ()
        n596 = case shown="真" w1202 {
          tunnel: [26 27] -> w1212
          frame False {
          }
          frame True {
            n597 = local write "Reset 6"(TRUE ("Reset 6")) -> ()
          }
        }
        n598 = Build Array (concatenate)(w1206, w1209) -> (w1205:dbl[])
        n599 = Array Size(array=w1205) -> (size(s)=w1196:i32)
        n600 = call "led显示更新字符串山推.vi"("显示字符"=w1197, "立显/保存"=FALSE) -> ("发送数据"=w1215:string)  [unwired: 9 in]
        n601 = Add Array Elements(numeric array=w1205) -> (sum=w1208:dbl)
        n602 = call "led发送数据并接收返回山推.vi"("发送数据"=w1215, "TCP网络连接输入"=w1213) -> ()  [unwired: 8 in, 2 out]
        n603 = local write "LED屏幕信息"(w1197) -> ()
        n604 = Divide(x=w1208, y=w1196) -> (x/y=→"D6平均速度":dbl)
        n605 = Enqueue Element(queue=w1211, element=w1212) -> (queue out=w1210:refnum<queue>)  [unwired: 2 in, 2 out]
      }
      frame 27 {
        n606 = local read "当前试验档位"() -> (w1223:string)
        n607 = local read "字符布尔"() -> (w1219:bool)
        n608 = case shown="\"N\"" w1223 {
          tunnel: [27 28] -> w1222
          frame "假", Default {
          }
          frame "N" {
          }
        }
        n609 = case shown="真" w1219 {
          tunnel: w1224 -> [_ w1228]
          frame False {
          }
          frame True {
            w1226 = "遥控器挂空挡"
            n610 = local write "字符布尔"(FALSE ("字符布尔")) -> ()
            n611 = call "led显示更新字符串山推.vi"("显示字符"=w1226, "立显/保存"=TRUE) -> ("发送数据"=w1230:string)  [unwired: 9 in]
            n612 = local write "LED屏幕信息"(w1226) -> ()
            n613 = call "led发送数据并接收返回山推.vi"("发送数据"=w1230, "TCP网络连接输入"=w1228) -> ()  [unwired: 8 in, 2 out]
          }
        }
        n614 = Enqueue Element(queue=w1221, element=w1222) -> (queue out=w1220:refnum<queue>)  [unwired: 2 in, 2 out]
      }
      frame 28 {
        n615 = local read "遥控器按钮确认"() -> (w1234:bool)
        n616 = local read "字符布尔"() -> (w1233:bool)
        n617 = call <vilib>:"Boolean Crossing PtByPt.vi"("direction"=enum16{"either", "false-true", "true-false"}."false-true", "input"=w1234) -> ("crossing"=w1235:bool)  [unwired: 1 in]
        n618 = case shown="假" w1233 {
          tunnel: w1241 -> [w1244 _]
          frame False {
            w1242 = "车辆请挂空挡"
            n619 = local write "字符布尔"(TRUE ("字符布尔")) -> ()
            n620 = local write "LED屏幕信息"(w1242) -> ()
            n621 = call "led显示更新字符串山推.vi"("显示字符"=w1242, "立显/保存"=TRUE) -> ("发送数据"=w1246:string)  [unwired: 9 in]
            n622 = call "led发送数据并接收返回山推.vi"("发送数据"=w1246, "TCP网络连接输入"=w1244) -> ()  [unwired: 8 in, 2 out]
          }
          frame True {
          }
        }
        n623 = case shown="真" w1235 {
          tunnel: [28 29] -> w1238
          frame False {
          }
          frame True {
          }
        }
        n624 = Enqueue Element(queue=w1240, element=w1238) -> (queue out=w1239:refnum<queue>)  [unwired: 2 in, 2 out]
      }
      frame 29 {
        n625 = local read "遥控器按钮确认"() -> (w1251:bool)
        n626 = local read "字符布尔"() -> (w1249:bool)
        n627 = case shown="真" w1249 {
          tunnel: w1257 -> [_ w1260]
          frame False {
          }
          frame True {
            w1258 = "车挂负一档，转速在2000转"
            n628 = local write "字符布尔"(FALSE ("字符布尔")) -> ()
            n629 = call "led显示更新字符串山推.vi"("显示字符"=w1258, "立显/保存"=TRUE) -> ("发送数据"=w1262:string)  [unwired: 9 in]
            n630 = local write "LED屏幕信息"(w1258) -> ()
            n631 = call "led发送数据并接收返回山推.vi"("发送数据"=w1262, "TCP网络连接输入"=w1260) -> ()  [unwired: 8 in, 2 out]
          }
        }
        n632 = call <vilib>:"Boolean Crossing PtByPt.vi"("direction"=enum16{"either", "false-true", "true-false"}."false-true", "input"=w1251) -> ("crossing"=w1250:bool)  [unwired: 1 in]
        n633 = case shown="真" w1250 {
          tunnel: [29 30] -> w1256
          frame False {
          }
          frame True {
          }
        }
        n634 = Enqueue Element(queue=w1255, element=w1256) -> (queue out=w1254:refnum<queue>)  [unwired: 2 in, 2 out]
      }
      frame 30 {
        n635 = local read "字符布尔"() -> (w1265:bool)
        n636 = local read "当前试验档位"() -> (w1270:string)
        n637 = case shown="假" w1265 {
          tunnel: w1271 -> [w1274 _]
          frame False {
            w1272 = "遥控器挂F1档"
            n638 = local write "字符布尔"(TRUE ("字符布尔")) -> ()
            n639 = call "led显示更新字符串山推.vi"("显示字符"=w1272, "立显/保存"=TRUE) -> ("发送数据"=w1276:string)  [unwired: 9 in]
            n640 = local write "LED屏幕信息"(w1272) -> ()
            n641 = call "led发送数据并接收返回山推.vi"("发送数据"=w1276, "TCP网络连接输入"=w1274) -> ()  [unwired: 8 in, 2 out]
          }
          frame True {
          }
        }
        n642 = case shown="\"R1\"" w1270 {
          tunnel: [30 31] -> w1269
          frame "假", Default {
          }
          frame "R1" {
          }
        }
        n643 = Enqueue Element(queue=w1268, element=w1269) -> (queue out=w1267:refnum<queue>)  [unwired: 2 in, 2 out]
      }
      frame 31 {
        n644 = local read "R1S"() -> (w1281:dbl)
        n645 = call "已用时间7"("Time Target (s)"=w1281, "Reset"="Reset 7") -> ("Time has Elapsed"=w1284:bool, "Elapsed Time Text"=w1286:string)  [unwired: 10 in, 6 out]
        n646 = call "输出文本.vi"("当前档位"="F1" ("字符串"), "字符串"=w1286) -> ("输出文本"=w1280:string)  [unwired: 9 in]
        n647 = local read "加载左上转速监控"() -> (w1291:dbl)
        n648 = local write "Reset 7"(FALSE ("Reset 7")) -> ()
        n649 = case shown="真" w1284 {
          tunnel: [31 32] -> w1292
          frame False {
          }
          frame True {
            n650 = local write "Reset 7"(TRUE ("Reset 7")) -> ()
          }
        }
        n651 = Build Array (concatenate)(w1288, w1291) -> (w1287:dbl[])
        n652 = Array Size(array=w1287) -> (size(s)=w1279:i32)
        n653 = local write "LED屏幕信息"(w1280) -> ()
        n654 = call "led显示更新字符串山推.vi"("显示字符"=w1280, "立显/保存"=FALSE) -> ("发送数据"=w1297:string)  [unwired: 9 in]
        n655 = Add Array Elements(numeric array=w1287) -> (sum=w1290:dbl)
        n656 = call "led发送数据并接收返回山推.vi"("发送数据"=w1297, "TCP网络连接输入"=w1295) -> ()  [unwired: 8 in, 2 out]
        n657 = Divide(x=w1290, y=w1279) -> (x/y=→"R1平均速度":dbl)
        n658 = Enqueue Element(queue=w1294, element=w1292) -> (queue out=w1293:refnum<queue>)  [unwired: 2 in, 2 out]
      }
      frame 32 {
        n659 = local read "当前试验档位"() -> (w1305:string)
        n660 = local read "字符布尔"() -> (w1301:bool)
        n661 = case shown="\"N\"" w1305 {
          tunnel: [32 33] -> w1304
          frame "假", Default {
          }
          frame "N" {
          }
        }
        n662 = case shown="真" w1301 {
          tunnel: w1306 -> [_ w1310]
          frame False {
          }
          frame True {
            w1308 = "遥控器挂空挡"
            n663 = local write "字符布尔"(FALSE ("字符布尔")) -> ()
            n664 = call "led显示更新字符串山推.vi"("显示字符"=w1308, "立显/保存"=TRUE) -> ("发送数据"=w1312:string)  [unwired: 9 in]
            n665 = local write "LED屏幕信息"(w1308) -> ()
            n666 = call "led发送数据并接收返回山推.vi"("发送数据"=w1312, "TCP网络连接输入"=w1310) -> ()  [unwired: 8 in, 2 out]
          }
        }
        n667 = Enqueue Element(queue=w1303, element=w1304) -> (queue out=w1302:refnum<queue>)  [unwired: 2 in, 2 out]
      }
      frame 33 {
        n668 = local read "遥控器按钮确认"() -> (w1317:bool)
        n669 = local read "字符布尔"() -> (w1315:bool)
        n670 = case shown="假" w1315 {
          tunnel: w1323 -> [w1326 _]
          frame False {
            w1324 = "车挂负二档，转速在2000转"
            n671 = local write "字符布尔"(TRUE ("字符布尔")) -> ()
            n672 = local write "LED屏幕信息"(w1324) -> ()
            n673 = call "led显示更新字符串山推.vi"("显示字符"=w1324, "立显/保存"=TRUE) -> ("发送数据"=w1328:string)  [unwired: 9 in]
            n674 = call "led发送数据并接收返回山推.vi"("发送数据"=w1328, "TCP网络连接输入"=w1326) -> ()  [unwired: 8 in, 2 out]
          }
          frame True {
          }
        }
        n675 = call <vilib>:"Boolean Crossing PtByPt.vi"("direction"=enum16{"either", "false-true", "true-false"}."false-true", "input"=w1317) -> ("crossing"=w1316:bool)  [unwired: 1 in]
        n676 = case shown="真" w1316 {
          tunnel: [33 34] -> w1320
          frame False {
          }
          frame True {
          }
        }
        n677 = Enqueue Element(queue=w1322, element=w1320) -> (queue out=w1321:refnum<queue>)  [unwired: 2 in, 2 out]
      }
      frame 34 {
        n678 = local read "当前试验档位"() -> (w1336:string)
        n679 = local read "字符布尔"() -> (w1331:bool)
        n680 = case shown="\"假\", 默认" w1336 {
          tunnel: [34 35] -> w1333
          frame "假", Default {
          }
          frame "R2" {
          }
        }
        n681 = case shown="真" w1331 {
          tunnel: w1337 -> [_ w1340]
          frame False {
          }
          frame True {
            w1338 = "遥控器挂F2档"
            n682 = local write "字符布尔"(FALSE ("字符布尔")) -> ()
            n683 = call "led显示更新字符串山推.vi"("显示字符"=w1338, "立显/保存"=TRUE) -> ("发送数据"=w1342:string)  [unwired: 9 in]
            n684 = local write "LED屏幕信息"(w1338) -> ()
            n685 = call "led发送数据并接收返回山推.vi"("发送数据"=w1342, "TCP网络连接输入"=w1340) -> ()  [unwired: 8 in, 2 out]
          }
        }
        n686 = Enqueue Element(queue=w1335, element=w1333) -> (queue out=w1334:refnum<queue>)  [unwired: 2 in, 2 out]
      }
      frame 35 {
        n687 = local read "R2S"() -> (w1347:dbl)
        n688 = call "已用时间8"("Time Target (s)"=w1347, "Reset"="Reset 8") -> ("Time has Elapsed"=w1353:bool, "Elapsed Time Text"=w1352:string)  [unwired: 10 in, 6 out]
        n689 = local read "加载左上转速监控"() -> (w1361:dbl)
        n690 = call "输出文本.vi"("当前档位"="F2" ("字符串"), "字符串"=w1352) -> ("输出文本"=w1346:string)  [unwired: 9 in]
        n691 = local write "Reset 8"(FALSE ("Reset 8")) -> ()
        n692 = local write "字符布尔"(TRUE ("字符布尔")) -> ()
        n693 = case shown="真" w1353 {
          tunnel: [35 36] -> w1356
          frame False {
          }
          frame True {
            n694 = local write "Reset 8"(TRUE ("Reset 8")) -> ()
          }
        }
        n695 = Build Array (concatenate)(w1358, w1361) -> (w1357:dbl[])
        n696 = Array Size(array=w1357) -> (size(s)=w1345:i32)
        n697 = call "led显示更新字符串山推.vi"("显示字符"=w1346, "立显/保存"=FALSE) -> ("发送数据"=w1364:string)  [unwired: 9 in]
        n698 = Add Array Elements(numeric array=w1357) -> (sum=w1360:dbl)
        n699 = call "led发送数据并接收返回山推.vi"("发送数据"=w1364, "TCP网络连接输入"=w1362) -> ()  [unwired: 8 in, 2 out]
        n700 = local write "LED屏幕信息"(w1346) -> ()
        n701 = Divide(x=w1360, y=w1345) -> (x/y=→"R2平均速度":dbl)
        n702 = Enqueue Element(queue=w1355, element=w1356) -> (queue out=w1354:refnum<queue>)  [unwired: 2 in, 2 out]
      }
      frame 36 {
        n703 = local read "当前试验档位"() -> (w1373:string)
        n704 = local read "字符布尔"() -> (w1368:bool)
        n705 = case shown="\"N\"" w1373 {
          tunnel: [36 37] -> w1372
          frame "假", Default {
          }
          frame "N" {
          }
        }
        n706 = case shown="真" w1368 {
          tunnel: w1374 -> [_ w1377]
          frame False {
          }
          frame True {
            w1375 = "遥控器挂空挡"
            n707 = local write "字符布尔"(FALSE ("字符布尔")) -> ()
            n708 = local write "LED屏幕信息"(w1375) -> ()
            n709 = call "led显示更新字符串山推.vi"("显示字符"=w1375, "立显/保存"=TRUE) -> ("发送数据"=w1379:string)  [unwired: 9 in]
            n710 = call "led发送数据并接收返回山推.vi"("发送数据"=w1379, "TCP网络连接输入"=w1377) -> ()  [unwired: 8 in, 2 out]
          }
        }
        n711 = Enqueue Element(queue=w1371, element=w1372) -> (queue out=w1370:refnum<queue>)  [unwired: 2 in, 2 out]
      }
      frame 37 {
        n712 = local read "遥控器按钮确认"() -> (w1384:bool)
        n713 = local read "字符布尔"() -> (w1382:bool)
        n714 = case shown="假" w1382 {
          tunnel: w1390 -> [w1393 _]
          frame False {
            w1391 = "车挂负三档，转速在2000转"
            n715 = local write "字符布尔"(TRUE ("字符布尔")) -> ()
            n716 = call "led显示更新字符串山推.vi"("显示字符"=w1391, "立显/保存"=TRUE) -> ("发送数据"=w1395:string)  [unwired: 9 in]
            n717 = local write "LED屏幕信息"(w1391) -> ()
            n718 = call "led发送数据并接收返回山推.vi"("发送数据"=w1395, "TCP网络连接输入"=w1393) -> ()  [unwired: 8 in, 2 out]
          }
          frame True {
          }
        }
        n719 = call <vilib>:"Boolean Crossing PtByPt.vi"("direction"=enum16{"either", "false-true", "true-false"}."false-true", "input"=w1384) -> ("crossing"=w1383:bool)  [unwired: 1 in]
        n720 = case shown="真" w1383 {
          tunnel: [37 38] -> w1387
          frame False {
          }
          frame True {
          }
        }
        n721 = Enqueue Element(queue=w1389, element=w1387) -> (queue out=w1388:refnum<queue>)  [unwired: 2 in, 2 out]
      }
      frame 38 {
        n722 = local read "当前试验档位"() -> (w1403:string)
        n723 = local read "字符布尔"() -> (w1398:bool)
        n724 = case shown="\"R3\"" w1403 {
          tunnel: [38 39] -> w1402
          frame "假", Default {
          }
          frame "R3" {
          }
        }
        n725 = case shown="真" w1398 {
          tunnel: w1404 -> [_ w1407]
          frame False {
          }
          frame True {
            w1405 = "遥控器挂F3档"
            n726 = local write "字符布尔"(FALSE ("字符布尔")) -> ()
            n727 = call "led显示更新字符串山推.vi"("显示字符"=w1405, "立显/保存"=TRUE) -> ("发送数据"=w1409:string)  [unwired: 9 in]
            n728 = local write "LED屏幕信息"(w1405) -> ()
            n729 = call "led发送数据并接收返回山推.vi"("发送数据"=w1409, "TCP网络连接输入"=w1407) -> ()  [unwired: 8 in, 2 out]
          }
        }
        n730 = Enqueue Element(queue=w1401, element=w1402) -> (queue out=w1400:refnum<queue>)  [unwired: 2 in, 2 out]
      }
      frame 39 {
        n731 = local read "R3S"() -> (w1414:dbl)
        n732 = call "已用时间9"("Time Target (s)"=w1414, "Reset"="Reset 9") -> ("Time has Elapsed"=w1418:bool, "Elapsed Time Text"=w1420:string)  [unwired: 10 in, 6 out]
        n733 = call "输出文本.vi"("当前档位"="F3" ("字符串"), "字符串"=w1420) -> ("输出文本"=w1413:string)  [unwired: 9 in]
        n734 = local read "加载左上转速监控"() -> (w1428:dbl)
        n735 = local write "Reset 9"(FALSE ("Reset 9")) -> ()
        n736 = local write "字符布尔"(TRUE ("字符布尔")) -> ()
        n737 = case shown="真" w1418 {
          tunnel: [39 40] -> w1421
          frame False {
          }
          frame True {
            n738 = local write "Reset 9"(TRUE ("Reset 9")) -> ()
          }
        }
        n739 = Build Array (concatenate)(w1425, w1428) -> (w1424:dbl[])
        n740 = call "led显示更新字符串山推.vi"("显示字符"=w1413, "立显/保存"=FALSE) -> ("发送数据"=w1431:string)  [unwired: 9 in]
        n741 = Array Size(array=w1424) -> (size(s)=w1412:i32)
        n742 = Add Array Elements(numeric array=w1424) -> (sum=w1427:dbl)
        n743 = call "led发送数据并接收返回山推.vi"("发送数据"=w1431, "TCP网络连接输入"=w1429) -> ()  [unwired: 8 in, 2 out]
        n744 = local write "LED屏幕信息"(w1413) -> ()
        n745 = Divide(x=w1427, y=w1412) -> (x/y=→"R3平均速度":dbl)
        n746 = Enqueue Element(queue=w1422, element=w1421) -> (queue out=w1423:refnum<queue>)  [unwired: 2 in, 2 out]
      }
      frame 40 {
        n747 = local read "当前试验档位"() -> (w1439:string)
        n748 = local read "字符布尔"() -> (w1435:bool)
        n749 = case shown="\"N\"" w1439 {
          tunnel: [40 41] -> w1436
          frame "假", Default {
          }
          frame "N" {
          }
        }
        n750 = case shown="真" w1435 {
          tunnel: w1440 -> [_ w1444]
          frame False {
          }
          frame True {
            w1442 = "遥控器挂空挡"
            n751 = local write "字符布尔"(FALSE ("字符布尔")) -> ()
            n752 = call "led显示更新字符串山推.vi"("显示字符"=w1442, "立显/保存"=TRUE) -> ("发送数据"=w1446:string)  [unwired: 9 in]
            n753 = local write "LED屏幕信息"(w1442) -> ()
            n754 = call "led发送数据并接收返回山推.vi"("发送数据"=w1446, "TCP网络连接输入"=w1444) -> ()  [unwired: 8 in, 2 out]
          }
        }
        n755 = Enqueue Element(queue=w1438, element=w1436) -> (queue out=w1437:refnum<queue>)  [unwired: 2 in, 2 out]
      }
      frame 41 {
        n756 = local read "遥控器按钮确认"() -> (w1451:bool)
        n757 = local read "字符布尔"() -> (w1449:bool)
        n758 = call <vilib>:"Boolean Crossing PtByPt.vi"("direction"=enum16{"either", "false-true", "true-false"}."false-true", "input"=w1451) -> ("crossing"=w1450:bool)  [unwired: 1 in]
        n759 = case shown="假" w1449 {
          tunnel: w1457 -> [w1460 _]
          frame False {
            w1458 = "车辆挂空挡"
            n760 = local write "字符布尔"(TRUE ("字符布尔")) -> ()
            n761 = call "led显示更新字符串山推.vi"("显示字符"=w1458, "立显/保存"=TRUE) -> ("发送数据"=w1462:string)  [unwired: 9 in]
            n762 = local write "LED屏幕信息"(w1458) -> ()
            n763 = call "led发送数据并接收返回山推.vi"("发送数据"=w1462, "TCP网络连接输入"=w1460) -> ()  [unwired: 8 in, 2 out]
          }
          frame True {
          }
        }
        n764 = case shown="真" w1450 {
          tunnel: [41 42] -> w1453
          frame False {
          }
          frame True {
          }
        }
        n765 = Enqueue Element(queue=w1456, element=w1453) -> (queue out=w1455:refnum<queue>)  [unwired: 2 in, 2 out]
      }
      frame 42 {
        # "由别的线程入队列"
        n766 = local read "字符布尔"() -> (w1465:bool)
        n767 = case shown="真" w1465 {
          tunnel: w1468 -> [_ w1471]
          frame False {
          }
          frame True {
            w1469 = "解开系固系统，浮动油缸，抬起举升，拆除连接，锁紧制动。"
            n768 = local write "字符布尔"(FALSE ("字符布尔")) -> ()
            n769 = local write "LED屏幕信息"(w1469) -> ()
            n770 = call "led显示更新字符串山推.vi"("显示字符"=w1469, "立显/保存"=TRUE) -> ("发送数据"=w1473:string)  [unwired: 9 in]
            n771 = call "led发送数据并接收返回山推.vi"("发送数据"=w1473, "TCP网络连接输入"=w1471) -> ()  [unwired: 8 in, 2 out]
          }
        }
      }
      frame 43 {
        w1474 = "实验完成，请出车"
        n772 = local write "LED屏幕信息"(w1474) -> ()
        n773 = call "led显示更新字符串山推.vi"("显示字符"=w1474, "立显/保存"=TRUE) -> ("发送数据"=w1479:string)  [unwired: 9 in]
        n774 = call "led发送数据并接收返回山推.vi"("发送数据"=w1479, "TCP网络连接输入"=w1477) -> ()  [unwired: 8 in, 2 out]
      }
      frame 44 {
        w1483 = "变频器故障！"
        n775 = local write "LED屏幕信息"(w1483) -> ()
        n776 = Enqueue Element(queue=w1482, element=44 ("元素")) -> (queue out=w1481:refnum<queue>)  [unwired: 2 in, 2 out]
        n777 = call "led显示更新字符串山推.vi"("显示字符"=w1483, "立显/保存"=FALSE) -> ("发送数据"=w1487:string)  [unwired: 9 in]
        n778 = call "led发送数据并接收返回山推.vi"("发送数据"=w1487, "TCP网络连接输入"=w1485) -> ()  [unwired: 8 in, 2 out]
      }
      frame 45 {
        w1493 = "遥控器中断！"
        n779 = local write "LED屏幕信息"(w1493) -> ()
        n780 = Enqueue Element(queue=w1490, element=45 ("元素")) -> (queue out=w1489:refnum<queue>)  [unwired: 2 in, 2 out]
        n781 = call "led显示更新字符串山推.vi"("显示字符"=w1493, "立显/保存"=FALSE) -> ("发送数据"=w1495:string)  [unwired: 9 in]
        n782 = call "led发送数据并接收返回山推.vi"("发送数据"=w1495, "TCP网络连接输入"=w1492) -> ()  [unwired: 8 in, 2 out]
      }
      frame 1, Default {
        n783 = local read "字符布尔"() -> (w1497:bool)
        n784 = case shown="假" w1497 {
          tunnel: w1499 -> [w1502 _]
          frame False {
            w1500 = "选择车型，输入编号，油缸调距。"
            n785 = local write "字符布尔"(TRUE ("字符布尔")) -> ()
            n786 = local write "LED屏幕信息"(w1500) -> ()
            n787 = call "led显示更新字符串山推.vi"("显示字符"=w1500, "立显/保存"=TRUE) -> ("发送数据"=w1504:string)  [unwired: 9 in]
            n788 = call "led发送数据并接收返回山推.vi"("发送数据"=w1504, "TCP网络连接输入"=w1502) -> ()  [unwired: 8 in, 2 out]
          }
          frame True {
          }
        }
      }
    }
    n789 = local read "停止"() -> (w787:bool)
    n790 = Wait (ms)(milliseconds to wait=u32 200 ("等待时间（毫秒）")) -> ()  [unwired: 1 out]
    "数值 3" <- w760
  }
  n791 = stacked-sequence {
    tunnel: w10 -> [_ w1539 _]
    frame #0 {
      w1536 = 0.0 ("D1平均速度")
      n792 = disable-structure shown="禁用" {
        frame Disabled {
          n793 = control-ref of="本VI"() -> (w1537:refnum<vi>)
          n794 = property class="VI"(reference=w1537, "Front Panel.PanelBounds"=T14 {"Left"=0, "Top"=0, "Right"=1280, "Bottom"=1024} ("前面板窗口:前面板边界")) -> ()  [unwired: 1 in, 2 out]
        }
        frame Enabled {
        }
      }
      n795 = call <vilib>:"Application Directory.vi"() -> ("Application Directory"=w1534:path)
      n796 = Build Path(base path=w1534, name or relative path="data\\参数配置.txt" ("名称或相对路径")) -> (appended path=w1532:path)
      n797 = Read from Binary File(5:"簇", 10:1 ("总数(1)"), 11:w1532) -> (2:w1531:T2)  [unwired: 3 in, 3 out]
      n798 = Index Array(array=w1531) -> (element=w1530:T1)  [unwired: 1 in]
      n799 = local write "停止"(FALSE ("停止")) -> ()
      n800 = Unbundle By Name(w1530) -> ("[0]"=w1529:T18, "[1]"=w1519:T18)
      n801 = Unbundle By Name(w1529) -> ("D1"=w1528:dbl, "D2"=w1527:dbl, "D3"=w1526:dbl, "D4"=w1525:dbl, "D5"=w1524:dbl, "D6"=w1523:dbl, "R1"=w1522:dbl, "R2"=w1521:dbl, "R3"=w1520:dbl, "SG14"=w1507:dbl, "SG16-3"=w1506:dbl, "SG18-3"=w1505:dbl)
      n802 = Unbundle By Name(w1519) -> ("D1"=w1518:dbl, "D2"=w1517:dbl, "D3"=w1516:dbl, "D4"=w1515:dbl, "D5"=w1514:dbl, "D6"=w1513:dbl, "R1"=w1512:dbl, "R2"=w1511:dbl, "R3"=w1510:dbl)
      n803 = local write "R1平均速度"(w1536) -> ()
      n804 = local write "R3平均速度"(w1536) -> ()
      n805 = local write "D4平均速度"(w1536) -> ()
      n806 = local write "D5平均速度"(w1536) -> ()
      n807 = local write "D6平均速度"(w1536) -> ()
      n808 = local write "R2平均速度"(w1536) -> ()
      n809 = local write "D3平均速度"(w1536) -> ()
      n810 = local write "D1平均速度"(w1536) -> ()
      n811 = local write "D2平均速度"(w1536) -> ()
      n812 = local write "D1S"(w1518) -> ()
      n813 = local write "D2S"(w1517) -> ()
      n814 = local write "D3S"(w1516) -> ()
      n815 = local write "D4S"(w1515) -> ()
      n816 = local write "D5S"(w1514) -> ()
      n817 = local write "D6S"(w1513) -> ()
      n818 = local write "R1S"(w1512) -> ()
      n819 = local write "R2S"(w1511) -> ()
      n820 = local write "R3S"(w1510) -> ()
      n821 = local write "D1"(w1528) -> ()
      n822 = local write "D2"(w1527) -> ()
      n823 = local write "D3"(w1526) -> ()
      n824 = local write "D4"(w1525) -> ()
      n825 = local write "D5"(w1524) -> ()
      n826 = local write "D6"(w1523) -> ()
      n827 = local write "R1"(w1522) -> ()
      n828 = local write "R2"(w1521) -> ()
      n829 = local write "R3"(w1520) -> ()
      n830 = local write "SG16-3百分比"(w1506) -> ()
      n831 = local write "SG18-3百分比"(w1505) -> ()
      n832 = local write "SG14百分比"(w1507) -> ()
    }
    frame #1 {
      n833 = while {
        shift-right: [w1543] -> _
        shift-left: enum16{"初始化", "事件结构", "退出"}."初始化" -> [w1544]
        tunnel: w1539 -> [w1541]
        stop <- w1542 stop-if-true
        n834 = case shown="\"事件结构\"" w1544 {
          tunnel: [enum16{"初始化", "事件结构", "退出"}."事件结构" w1761 enum16{"初始化", "事件结构", "退出"}."退出"] -> w1543
          tunnel: [FALSE FALSE TRUE] -> w1542
          tunnel: w1541 -> [_ w1757 _]
          frame "初始化", Default {
          }
          frame "事件结构" {
            # "AD25-AD31"
            # "AD17-AD24"
            # "AD9-AD16"
            # "中左在EM9636通道前，此模块为右模块"
            n835 = local read "输出数组左"() -> (w1756:dbl[][])
            n836 = local read "试验车型"() -> (w1758:u16)
            n837 = event shown="[6] \"刷新参数\": 值改变" {
              selector: _ -> [_ _ _ _ _ _ _ _ _]
              dyn-events: _ -> [_ _ _ _ _ _ _ _ _]
              timeout: 100 -> [_ _ _ _ _ _ _ _ _]
              tunnel: [enum16{"初始化", "事件结构", "退出"}."事件结构" enum16{"初始化", "事件结构", "退出"}."事件结构" enum16{"初始化", "事件结构", "退出"}."事件结构" enum16{"初始化", "事件结构", "退出"}."事件结构" enum16{"初始化", "事件结构", "退出"}."事件结构" enum16{"初始化", "事件结构", "退出"}."事件结构" enum16{"初始化", "事件结构", "退出"}."事件结构" enum16{"初始化", "事件结构", "退出"}."事件结构" enum16{"初始化", "事件结构", "退出"}."退出"] -> w1761
              tunnel: w1757 -> [_ w1884 w1899 _ w1999 _ _ w2170 _]
              event Timeout {
                n838 = event-data() -> ()  [unwired: 1 in, 3 out]
                n839 = Format Date/Time String(time format string (%c)="%Y年%m月%d日 %H:%M:%S" ("时间格式字符串(%c)")) -> (date/time string=→"系统时间 2":string)  [unwired: 2 in]
              }
              event "确认输入": Value Change {
                # "D1档速度"
                n840 = event-data() -> ()  [unwired: 1 in, 6 out]
                n841 = Flush Queue(queue=w1884) -> (queue out=w1883:refnum<queue>)  [unwired: 1 in, 2 out]
                n842 = Enqueue Element(queue=w1883, element=2 ("元素")) -> ()  [unwired: 2 in, 3 out]
                n843 = case shown="3" "试验车型" {
                  tunnel: ["SG21" "SG14" "SG16" "SG18"] -> w1891
                  frame 0, Default {
                  }
                  frame 1 {
                  }
                  frame 2 {
                  }
                  frame 3 {
                  }
                }
                "车型" <- w1891
                n844 = Concatenate Strings("试验车编号", "（", "具体车型", "）") -> (w1877:string)
                "表格名称" <- w1877
                n845 = local write "等待进车布尔"(TRUE ("等待进车布尔")) -> ()
                n846 = Build Array(w1891, w1877, "发动机编号", "操作者") -> (w1887:string[])
                "中间数组" <- w1887
                n847 = Build Array (concatenate)(string[][] [], w1887) -> (→"实验基本信息":string[][])
              }
              event "试验开始": Value Change {
                n848 = event-data() -> ("NewVal"=w1900:bool)  [unwired: 1 in, 5 out]
                n849 = case shown="真" w1900 {
                  tunnel: w1899 -> [w1902 w1918]
                  frame False {
                    n850 = Flush Queue(queue=w1902) -> (queue out=w1901:refnum<queue>)  [unwired: 1 in, 2 out]
                    n851 = Enqueue Element(queue=w1901, element=43 ("元素")) -> ()  [unwired: 2 in, 3 out]
                    n852 = property on="加载电机右上启动" class="Bool (严格)"("Val(Sgnl)"=FALSE ("值(信号)")) -> ()  [unwired: 2 in, 2 out]
                    n853 = property on="加载电机左上启动" class="Bool (严格)"("Val(Sgnl)"=FALSE ("值(信号)")) -> ()  [unwired: 2 in, 2 out]
                    n854 = property on="加载电机左下启动" class="Bool (严格)"("Val(Sgnl)"=FALSE ("值(信号)")) -> ()  [unwired: 2 in, 2 out]
                    n855 = property on="驱动电机下启动" class="Bool (严格)"("Val(Sgnl)"=FALSE ("值(信号)")) -> ()  [unwired: 2 in, 2 out]
                    n856 = property on="加载电机右下启动" class="Bool (严格)"("Val(Sgnl)"=FALSE ("值(信号)")) -> ()  [unwired: 2 in, 2 out]
                    n857 = property on="驱动电机上启动" class="Bool (严格)"("Val(Sgnl)"=FALSE ("值(信号)")) -> ()  [unwired: 2 in, 2 out]
                  }
                  frame True {
                    w1910 = TRUE
                    n858 = Flush Queue(queue=w1918) -> (queue out=w1917:refnum<queue>)  [unwired: 1 in, 2 out]
                    n859 = Enqueue Element(queue=w1917, element=1 ("元素")) -> ()  [unwired: 2 in, 3 out]
                    n860 = local write "变频6"(w1910) -> ()
                    n861 = local write "变频5"(w1910) -> ()
                    n862 = local write "变频4"(w1910) -> ()
                    n863 = local write "字符布尔"(FALSE ("字符布尔")) -> ()
                    n864 = local write "变频3"(w1910) -> ()
                    n865 = local write "变频2"(w1910) -> ()
                    n866 = local write "变频1"(w1910) -> ()
                    n867 = property on="加载电机右上启动" class="Bool (严格)"("Val(Sgnl)"=TRUE ("值(信号)")) -> ()  [unwired: 2 in, 2 out]
                    n868 = property on="加载电机左上启动" class="Bool (严格)"("Val(Sgnl)"=TRUE ("值(信号)")) -> ()  [unwired: 2 in, 2 out]
                    n869 = property on="加载电机左下启动" class="Bool (严格)"("Val(Sgnl)"=TRUE ("值(信号)")) -> ()  [unwired: 2 in, 2 out]
                    n870 = property on="驱动电机下启动" class="Bool (严格)"("Val(Sgnl)"=TRUE ("值(信号)")) -> ()  [unwired: 2 in, 2 out]
                    n871 = property on="加载电机右下启动" class="Bool (严格)"("Val(Sgnl)"=TRUE ("值(信号)")) -> ()  [unwired: 2 in, 2 out]
                    n872 = property on="驱动电机上启动" class="Bool (严格)"("Val(Sgnl)"=TRUE ("值(信号)")) -> ()  [unwired: 2 in, 2 out]
                  }
                }
              }
              event "生成报表": Value Change {
                n873 = event-data() -> ()  [unwired: 1 in, 6 out]
                n874 = flat-sequence {
                  frame #0 {
                    w1926 = u16 2 items=["US", "公制", "默认"] ("measurement system")
                    w1927 = u16 2 items=["US", "公制", "默认"] ("measurement system")
                    w1928 = u16 2 items=["US", "公制", "默认"] ("measurement system")
                    w1930 = -1.0 ("column width (1)")
                    n875 = local read "实验基本信息"() -> (w1984:string[][])
                    n876 = local read "R1平均速度"() -> (w1953:dbl)
                    n877 = local read "R3平均速度"() -> (w1951:dbl)
                    n878 = local read "D4平均速度"() -> (w1956:dbl)
                    n879 = local read "D5平均速度"() -> (w1955:dbl)
                    n880 = local read "D6平均速度"() -> (w1954:dbl)
                    n881 = local read "R2平均速度"() -> (w1952:dbl)
                    n882 = local read "D3平均速度"() -> (w1957:dbl)
                    n883 = local read "D1平均速度"() -> (w1959:dbl)
                    n884 = local read "D2平均速度"() -> (w1958:dbl)
                    n885 = local read "系统时间 2"() -> (w1934:string)
                    n886 = call <vilib>:"New Report.vi"("report type"=T16."Excel", "template (empty)"=path "E:/模板/输出数据表格.xlsx") -> ("report out"=w1985:refnum<class "NI_report.lvclass">, "error out"=w1966:errorcluster)  [unwired: 12 in]
                    n887 = Build Array(w1959, w1958, w1957, w1956, w1955, w1954, w1953, w1952, w1951) -> (w1950:dbl[])
                    n888 = call-poly <vilib>:"Append Table to Report.vi"("report in"=w1985, "column width (1)"=w1930, "measurement system"=w1927, "MS Office parameters"=T15 {"position (excel)"={"row"=5, "column"=2}, "name (excel)"="", "bookmark (word)"=""}, "text data"=w1984, "error in (no error)"=w1966) -> ("report out"=w1938:refnum<class "NI_report.lvclass">, "error out"=w1939:errorcluster)  [unwired: 6 in, 2 out]
                    n889 = for {
                      tunnel: w1950 -> [w1991] mode=indexing
                      tunnel: [w1992] -> w1949 mode=indexing
                      n890 = Multiply(x=w1991, y=-1.0) -> (x*y=w1988:dbl)
                      n891 = Absolute Value(x=w1988) -> (abs(x)=w1989:dbl)
                      n892 = call "speed.vi"("rmp"=w1989) -> ("km/h"=w1992:dbl)  [unwired: 10 in]
                    }
                    n893 = Initialize Array(w1934, 1 ("维数大小"), 1 ("维数大小")) -> (w1931:string[][])
                    n894 = call-poly <vilib>:"Append Table to Report.vi"("report in"=w1938, "column width (1)"=w1930, "measurement system"=w1928, "MS Office parameters"=T15 {"position (excel)"={"row"=3, "column"=3}, "name (excel)"="", "bookmark (word)"=""}, "text data"=w1931, "error in (no error)"=w1939) -> ("report out"=w1937:refnum<class "NI_report.lvclass">, "error out"=w1936:errorcluster)  [unwired: 6 in, 2 out]
                    n895 = local read "环境温度标定"() -> (w1974:dbl)
                    n896 = local read "液压油箱温度标定"() -> (w1975:dbl)
                    n897 = local read "变矩器出口温度标定"() -> (w1976:dbl)
                    n898 = local read "左前轮轴承温度标定"() -> (w1977:dbl)
                    n899 = local read "右前轮轴承温度标定"() -> (w1978:dbl)
                    n900 = local read "振动泵压力"() -> (w1979:dbl)
                    n901 = local read "转向泵压力"() -> (w1980:dbl)
                    n902 = Index Array(array=w1949) -> (element #1=w1948:dbl, element #2=w1947:dbl, element #3=w1946:dbl, element #4=w1945:dbl, element #5=w1944:dbl, element #6=w1943:dbl, element #7=w1942:dbl, element #8=w1941:dbl, element #9=w1940:dbl)  [unwired: 9 in]
                    n903 = Build Array(w1974, w1975, w1976, w1977, w1978, w1979, w1980, w1948, w1947, w1946, w1945, w1944, w1943, w1942, w1941, w1940) -> (w1981:dbl[])
                    n904 = local read "表格名称"() -> (w1922:string)
                    n905 = for {
                      tunnel: w1981 -> [w1994] mode=indexing
                      tunnel: [w1993] -> w1982 mode=indexing
                      n906 = Number To Fractional String(number=w1994, precision (6)=i16 2 ("宽度(-)")) -> (F-format string=w1993:string)  [unwired: 2 in]
                    }
                    n907 = Build Array (concatenate)("速度温度", w1982) -> (w1972:string[][])
                    n908 = local read "试验车编号"() -> (w1925:string)
                    n909 = Transpose 2D Array(2D array=w1972) -> (transposed array=w1971:string[][])
                    n910 = call-poly <vilib>:"Append Table to Report.vi"("report in"=w1937, "column width (1)"=-1.0, "measurement system"=w1926, "MS Office parameters"=T15 {"position (excel)"={"row"=7, "column"=5}, "name (excel)"="", "bookmark (word)"=""}, "text data"=w1971, "error in (no error)"=w1936) -> ("report out"=w1969:refnum<class "NI_report.lvclass">, "error out"=w1964:errorcluster)  [unwired: 6 in, 2 out]
                    n911 = Concatenate Strings(w1922, "_" ("字符串"), w1925) -> (w1924:string)
                    n912 = Build Path(base path=path "E:/数据保存" ("基路径"), name or relative path=w1924) -> (appended path=w1961:path)
                    n913 = call-dynamic "Save Report to File.vi"("report in"=w1969, "report file path"=w1961, "prompt to replace? (F)"=FALSE, "error in (no error)"=w1964) -> ("report out"=w1968:refnum<class "NI_report.lvclass">, "error out"=w1963:errorcluster)  [unwired: 10 in]
                    n914 = call-dynamic "Dispose Report.vi"("report in"=w1968, "wait until printing completed? (T)"=TRUE, "error in (no error)"=w1963) -> ("error out"=w1960:errorcluster)  [unwired: 12 in]
                    n915 = call <vilib>:"Clear Errors.vi"("error in (no error)"=w1960) -> ()  [unwired: 5 in, 2 out]
                  }
                  frame #1 {
                    w1996 = string[][] []
                    n916 = local write "实验基本信息"(w1996) -> ()
                    n917 = local write "速度温度"(w1996) -> ()
                  }
                }
              }
              event "重新实验": Value Change {
                n918 = event-data() -> ()  [unwired: 1 in, 6 out]
                n919 = Flush Queue(queue=w1999) -> (queue out=w1998:refnum<queue>)  [unwired: 1 in, 2 out]
                n920 = Enqueue Element(queue=w1998, element=2 ("元素")) -> ()  [unwired: 2 in, 3 out]
                n921 = local write "速度温度"(string[][] []) -> ()
                "等待进车布尔" <- TRUE ("重新实验布尔")
              }
              event "高级参数": Value Change {
                n922 = event-data() -> ()  [unwired: 1 in, 6 out]
                n923 = property class="App"() -> ("App.Kind"=w2015:T19)  [unwired: 2 in, 2 out]
                n924 = case shown="\"Run Time System\"" w2015 {
                  tunnel: ["授权文件\\登录界面.vi" ("名称或相对路径") "..\\授权文件\\登录界面.vi" ("名称或相对路径")] -> w2016
                  tunnel: [w2018 w2021] -> w2017
                  frame "Development System", Default {
                    n925 = call <vilib>:"Application Directory.vi"() -> ("Application Directory"=w2018:path)
                  }
                  frame "Run Time System" {
                    n926 = Current VI's Path() -> (path=w2021:path)
                  }
                }
                n927 = Build Path(base path=w2017, name or relative path=w2016) -> (appended path=w2004:path)
                n928 = Open VI Reference(vi path=w2004) -> (vi reference=w2008:refnum<vi>, error out=w2011:errorcluster)  [unwired: 5 in]
                n929 = invoke class="VI" method="FP.Open"(reference=w2008, error in=w2011, "Activate"=TRUE ("激活？"), "State"=T17."Standard" ("状态")) -> (reference out=w2005:refnum<vi>, error out=w2012:errorcluster)  [unwired: 1 in, 3 out]
                n930 = invoke class="VI" method="Run VI"(reference=w2005, error in=w2012, "Wait until done"=FALSE ("结束前等待")) -> (reference out=w2007:refnum<vi>, error out=w2013:errorcluster)  [unwired: 2 in, 3 out]
                n931 = Close Reference(reference=w2007, error in (no error)=w2013) -> (error out=→"错误输出 7":errorcluster)
              }
              event "刷新参数": Value Change {
                n932 = event-data() -> ()  [unwired: 1 in, 6 out]
                n933 = call <vilib>:"Application Directory.vi"() -> ("Application Directory"=w2064:path)
                n934 = Build Path(base path=w2064, name or relative path="data\\参数配置.txt" ("名称或相对路径")) -> (appended path=w2062:path)
                n935 = Read from Binary File(5:"簇 3", 10:1 ("总数(1)"), 11:w2062) -> (2:w2059:T2)  [unwired: 3 in, 3 out]
                "数据" <- w2059
                n936 = Index Array(array=w2059) -> (element=w2061:T1)  [unwired: 1 in]
                n937 = Unbundle By Name(w2061) -> ("[0]"=w2060:T18, "[1]"=w2035:T18, "[2]"=w2034:T18, "[3]"=w2033:T18, "[4]"=w2032:T18)
                n938 = Unbundle By Name(w2060) -> ("D1"=w2057:dbl, "D2"=w2056:dbl, "D3"=w2055:dbl, "D4"=w2054:dbl, "D5"=w2053:dbl, "D6"=w2052:dbl, "R1"=w2051:dbl, "R2"=w2050:dbl, "R3"=w2049:dbl, "SG14"=w2048:dbl, "SG16-3"=w2047:dbl, "SG18-3"=w2046:dbl)
                "D3" <- w2055
                "D4" <- w2054
                "D5" <- w2053
                "D6" <- w2052
                "R1" <- w2051
                "R2" <- w2050
                "R3" <- w2049
                "D2" <- w2056
                "D1" <- w2057
                "SG14百分比" <- w2048
                "SG16-3百分比" <- w2047
                "SG18-3百分比" <- w2046
                n939 = local read "试验车型"() -> (w2058:u16)
                n940 = case shown="0, 默认" w2058 {
                  tunnel: w2057 -> [w2087 w2112 w2137 w2162]
                  tunnel: w2056 -> [w2086 w2111 w2136 w2161]
                  tunnel: w2055 -> [w2085 w2110 w2135 w2160]
                  tunnel: w2054 -> [w2084 w2109 w2134 w2159]
                  tunnel: w2053 -> [w2083 w2108 w2133 w2158]
                  tunnel: w2052 -> [w2082 w2107 w2132 w2157]
                  tunnel: w2051 -> [w2081 w2106 w2131 w2156]
                  tunnel: w2050 -> [w2080 w2105 w2130 w2155]
                  tunnel: w2049 -> [w2079 w2104 w2129 w2154]
                  tunnel: w2048 -> [_ w2102 _ _]
                  tunnel: w2047 -> [_ _ w2127 _]
                  tunnel: w2046 -> [_ _ _ w2152]
                  tunnel: [w2076 w2100 w2125 w2150] -> w2045
                  tunnel: [w2075 w2099 w2124 w2149] -> w2044
                  tunnel: [w2074 w2098 w2123 w2148] -> w2043
                  tunnel: [w2073 w2097 w2122 w2147] -> w2042
                  tunnel: [w2072 w2096 w2121 w2146] -> w2041
                  tunnel: [w2071 w2095 w2120 w2145] -> w2040
                  tunnel: [w2070 w2094 w2119 w2144] -> w2039
                  tunnel: [w2069 w2093 w2118 w2143] -> w2038
                  tunnel: [w2068 w2092 w2117 w2142] -> w2037
                  tunnel: w2035 -> [w2067 _ _ _]
                  tunnel: w2034 -> [_ w2091 _ _]
                  tunnel: w2033 -> [_ _ w2116 _]
                  tunnel: w2032 -> [_ _ _ w2141]
                  tunnel: [w2067 w2091 w2116 w2141] -> w2031
                  frame 0, Default {
                    n941 = Build Array(w2087, w2086, w2085, w2084, w2083, w2082, w2081, w2080, w2079) -> (w2078:dbl[])
                    n942 = for {
                      tunnel: w2078 -> [w2090] mode=indexing
                      tunnel: [w2088] -> w2077 mode=indexing
                      n943 = call "实验车型选择比例 (子VI).vi"("SG14百分比"=100.0, "D1"=w2090) -> ("数值"=w2088:dbl)  [unwired: 9 in]
                    }
                    n944 = Index Array(array=w2077) -> (element #1=w2076:dbl, element #2=w2075:dbl, element #3=w2074:dbl, element #4=w2073:dbl, element #5=w2072:dbl, element #6=w2071:dbl, element #7=w2070:dbl, element #8=w2069:dbl, element #9=w2068:dbl)  [unwired: 9 in]
                  }
                  frame 1 {
                    n945 = Build Array(w2112, w2111, w2110, w2109, w2108, w2107, w2106, w2105, w2104) -> (w2103:dbl[])
                    n946 = for {
                      tunnel: w2103 -> [w2115] mode=indexing
                      tunnel: w2102 -> [w2114]
                      tunnel: [w2113] -> w2101 mode=indexing
                      n947 = call "实验车型选择比例 (子VI).vi"("SG14百分比"=w2114, "D1"=w2115) -> ("数值"=w2113:dbl)  [unwired: 9 in]
                    }
                    n948 = Index Array(array=w2101) -> (element #1=w2100:dbl, element #2=w2099:dbl, element #3=w2098:dbl, element #4=w2097:dbl, element #5=w2096:dbl, element #6=w2095:dbl, element #7=w2094:dbl, element #8=w2093:dbl, element #9=w2092:dbl)  [unwired: 9 in]
                  }
                  frame 2 {
                    n949 = Build Array(w2137, w2136, w2135, w2134, w2133, w2132, w2131, w2130, w2129) -> (w2128:dbl[])
                    n950 = for {
                      tunnel: w2128 -> [w2140] mode=indexing
                      tunnel: w2127 -> [w2139]
                      tunnel: [w2138] -> w2126 mode=indexing
                      n951 = call "实验车型选择比例 (子VI).vi"("SG14百分比"=w2139, "D1"=w2140) -> ("数值"=w2138:dbl)  [unwired: 9 in]
                    }
                    n952 = Index Array(array=w2126) -> (element #1=w2125:dbl, element #2=w2124:dbl, element #3=w2123:dbl, element #4=w2122:dbl, element #5=w2121:dbl, element #6=w2120:dbl, element #7=w2119:dbl, element #8=w2118:dbl, element #9=w2117:dbl)  [unwired: 9 in]
                  }
                  frame 3 {
                    n953 = Build Array(w2162, w2161, w2160, w2159, w2158, w2157, w2156, w2155, w2154) -> (w2153:dbl[])
                    n954 = for {
                      tunnel: w2153 -> [w2165] mode=indexing
                      tunnel: w2152 -> [w2164]
                      tunnel: [w2163] -> w2151 mode=indexing
                      n955 = call "实验车型选择比例 (子VI).vi"("SG14百分比"=w2164, "D1"=w2165) -> ("数值"=w2163:dbl)  [unwired: 9 in]
                    }
                    n956 = Index Array(array=w2151) -> (element #1=w2150:dbl, element #2=w2149:dbl, element #3=w2148:dbl, element #4=w2147:dbl, element #5=w2146:dbl, element #6=w2145:dbl, element #7=w2144:dbl, element #8=w2143:dbl, element #9=w2142:dbl)  [unwired: 9 in]
                  }
                }
                "D3 act" <- w2043
                "D4 act" <- w2042
                "D5 act" <- w2041
                "D6 act" <- w2040
                "R1 act" <- w2039
                "R2 act" <- w2038
                "R3 act" <- w2037
                "D2 act" <- w2044
                "D1 act" <- w2045
                n957 = Unbundle By Name(w2031) -> ("D1"=→"D1S":dbl, "D2"=→"D2S":dbl, "D3"=→"D3S":dbl, "D4"=→"D4S":dbl, "D5"=→"D5S":dbl, "D6"=→"D6S":dbl, "R1"=→"R1S":dbl, "R2"=→"R2S":dbl, "R3"=→"R3S":dbl)
              }
              event "确认换挡": Value Change {
                w2166 = TRUE ("Reset")
                w2168 = TRUE
                n958 = event-data() -> ()  [unwired: 1 in, 6 out]
                n959 = Flush Queue(queue=w2170) -> (queue out=w2169:refnum<queue>)  [unwired: 1 in, 2 out]
                n960 = case shown="\"D5\"" "重新选档档位" {
                  tunnel: w2169 -> [w2175 w2178 w2181 w2184 w2188 w2192 w2195 w2198 w2202]
                  frame "D1", Default {
                    n961 = Enqueue Element(queue=w2175, element=4 ("元素")) -> ()  [unwired: 2 in, 3 out]
                    n962 = local write "字符布尔"(FALSE ("字符布尔")) -> ()
                  }
                  frame "D2" {
                    n963 = local write "字符布尔"(FALSE ("字符布尔")) -> ()
                    n964 = Enqueue Element(queue=w2178, element=8 ("元素")) -> ()  [unwired: 2 in, 3 out]
                  }
                  frame "D3" {
                    n965 = local write "字符布尔"(FALSE ("字符布尔")) -> ()
                    n966 = Enqueue Element(queue=w2181, element=12 ("元素")) -> ()  [unwired: 2 in, 3 out]
                  }
                  frame "D4" {
                    n967 = local write "字符布尔"(FALSE ("字符布尔")) -> ()
                    n968 = Enqueue Element(queue=w2184, element=16 ("元素")) -> ()  [unwired: 2 in, 3 out]
                  }
                  frame "D5" {
                    n969 = Enqueue Element(queue=w2188, element=20 ("元素")) -> ()  [unwired: 2 in, 3 out]
                    n970 = local write "字符布尔"(FALSE ("字符布尔")) -> ()
                    n971 = local write "ini_D5"(TRUE ("ini_D5")) -> ()
                  }
                  frame "D6" {
                    n972 = Enqueue Element(queue=w2192, element=24 ("元素")) -> ()  [unwired: 2 in, 3 out]
                    n973 = local write "字符布尔"(FALSE ("字符布尔")) -> ()
                    n974 = local write "ini_D6"(TRUE ("ini_D6")) -> ()
                  }
                  frame "R1" {
                    n975 = local write "字符布尔"(TRUE ("字符布尔")) -> ()
                    n976 = Enqueue Element(queue=w2195, element=29 ("元素")) -> ()  [unwired: 2 in, 3 out]
                  }
                  frame "R2" {
                    n977 = local write "字符布尔"(FALSE ("字符布尔")) -> ()
                    n978 = Enqueue Element(queue=w2198, element=33 ("元素")) -> ()  [unwired: 2 in, 3 out]
                  }
                  frame "R3" {
                    n979 = local write "字符布尔"(FALSE ("字符布尔")) -> ()
                    n980 = Enqueue Element(queue=w2202, element=37 ("元素")) -> ()  [unwired: 2 in, 3 out]
                    n981 = local write "ini_R3"(TRUE ("ini_R3")) -> ()
                  }
                }
                n982 = local write "Reset 7"(w2166) -> ()
                n983 = local write "Reset 9"(w2166) -> ()
                n984 = local write "Reset 8"(w2166) -> ()
                n985 = local write "Reset"(w2166) -> ()
                n986 = local write "Reset 2"(w2166) -> ()
                n987 = local write "Reset 3"(w2166) -> ()
                n988 = local write "Reset 4"(w2166) -> ()
                n989 = local write "Reset 5"(w2166) -> ()
                n990 = local write "Reset 6"(w2166) -> ()
                n991 = local write "变频6"(w2168) -> ()
                n992 = local write "变频5"(w2168) -> ()
                n993 = local write "变频4"(w2168) -> ()
                n994 = local write "变频3"(w2168) -> ()
                n995 = local write "变频2"(w2168) -> ()
                n996 = local write "变频1"(w2168) -> ()
                n997 = local write "comcnt"(u16 0 ("comcnt")) -> ()
              }
              event "停止": Value Change {
                n998 = event-data() -> ()  [unwired: 1 in, 6 out]
              }
            }
            n999 = Index Array(array=w1756) -> (element #1=w1754:dbl[], element #2=w1743:dbl[], element #3=w1734:dbl[], element #4=w1724:dbl[])  [unwired: 8 in]
            n1000 = case shown="0, 默认" w1758 {
              frame 0, Default {
                n1001 = local read "D1"() -> (w1798:dbl)
                n1002 = local read "D2"() -> (w1797:dbl)
                n1003 = local read "D3"() -> (w1796:dbl)
                n1004 = local read "D4"() -> (w1795:dbl)
                n1005 = local read "D5"() -> (w1794:dbl)
                n1006 = local read "D6"() -> (w1793:dbl)
                n1007 = local read "R1"() -> (w1792:dbl)
                n1008 = local read "R2"() -> (w1791:dbl)
                n1009 = local read "R3"() -> (w1790:dbl)
                n1010 = Build Array(w1798, w1797, w1796, w1795, w1794, w1793, w1792, w1791, w1790) -> (w1789:dbl[])
                n1011 = for {
                  tunnel: w1789 -> [w1801] mode=indexing
                  tunnel: [w1800] -> w1788 mode=indexing
                  tunnel: 100.0 -> [w1799]
                  n1012 = call "档位加载比例 (子VI).vi"("更换车型加载比例"=w1799, "D1-D3/R1/R2加载比例"=w1801) -> ("数值"=w1800:dbl)  [unwired: 9 in]
                }
                n1013 = Index Array(array=w1788) -> (element #1=w1787:dbl, element #2=w1786:dbl, element #3=w1785:dbl, element #4=w1784:dbl, element #5=w1783:dbl, element #6=w1782:dbl, element #7=w1781:dbl, element #8=w1780:dbl, element #9=w1779:dbl)  [unwired: 9 in]
                n1014 = local write "D1扭矩给定"(w1787) -> ()
                n1015 = local write "D2扭矩给定"(w1786) -> ()
                n1016 = local write "D3扭矩给定"(w1785) -> ()
                n1017 = local write "D4扭矩给定"(w1784) -> ()
                n1018 = local write "D5扭矩给定"(w1783) -> ()
                n1019 = local write "D6扭矩给定"(w1782) -> ()
                n1020 = local write "R1扭矩给定"(w1781) -> ()
                n1021 = local write "R2扭矩给定"(w1780) -> ()
                n1022 = local write "R3扭矩给定"(w1779) -> ()
              }
              frame 1 {
                n1023 = local read "D1"() -> (w1820:dbl)
                n1024 = local read "D2"() -> (w1819:dbl)
                n1025 = local read "D3"() -> (w1818:dbl)
                n1026 = local read "D4"() -> (w1817:dbl)
                n1027 = local read "D5"() -> (w1816:dbl)
                n1028 = local read "D6"() -> (w1815:dbl)
                n1029 = local read "R1"() -> (w1814:dbl)
                n1030 = local read "R2"() -> (w1813:dbl)
                n1031 = local read "R3"() -> (w1812:dbl)
                n1032 = local read "SG14百分比"() -> (w1802:dbl)
                n1033 = Build Array(w1820, w1819, w1818, w1817, w1816, w1815, w1814, w1813, w1812) -> (w1822:dbl[])
                n1034 = for {
                  tunnel: w1822 -> [w1824] mode=indexing
                  tunnel: [w1825] -> w1821 mode=indexing
                  tunnel: w1802 -> [w1823]
                  n1035 = call "档位加载比例 (子VI).vi"("更换车型加载比例"=w1823, "D1-D3/R1/R2加载比例"=w1824) -> ("数值"=w1825:dbl)  [unwired: 9 in]
                }
                n1036 = Index Array(array=w1821) -> (element #1=w1811:dbl, element #2=w1810:dbl, element #3=w1809:dbl, element #4=w1808:dbl, element #5=w1807:dbl, element #6=w1806:dbl, element #7=w1805:dbl, element #8=w1804:dbl, element #9=w1803:dbl)  [unwired: 9 in]
                n1037 = local write "D1扭矩给定"(w1811) -> ()
                n1038 = local write "D2扭矩给定"(w1810) -> ()
                n1039 = local write "D3扭矩给定"(w1809) -> ()
                n1040 = local write "D4扭矩给定"(w1808) -> ()
                n1041 = local write "D5扭矩给定"(w1807) -> ()
                n1042 = local write "D6扭矩给定"(w1806) -> ()
                n1043 = local write "R1扭矩给定"(w1805) -> ()
                n1044 = local write "R2扭矩给定"(w1804) -> ()
                n1045 = local write "R3扭矩给定"(w1803) -> ()
              }
              frame 2 {
                n1046 = local read "D1"() -> (w1844:dbl)
                n1047 = local read "D2"() -> (w1843:dbl)
                n1048 = local read "D3"() -> (w1842:dbl)
                n1049 = local read "D4"() -> (w1841:dbl)
                n1050 = local read "D5"() -> (w1840:dbl)
                n1051 = local read "D6"() -> (w1839:dbl)
                n1052 = local read "R1"() -> (w1838:dbl)
                n1053 = local read "R2"() -> (w1837:dbl)
                n1054 = local read "R3"() -> (w1836:dbl)
                n1055 = local read "SG16-3百分比"() -> (w1826:dbl)
                n1056 = Build Array(w1844, w1843, w1842, w1841, w1840, w1839, w1838, w1837, w1836) -> (w1846:dbl[])
                n1057 = for {
                  tunnel: w1846 -> [w1848] mode=indexing
                  tunnel: [w1849] -> w1845 mode=indexing
                  tunnel: w1826 -> [w1847]
                  n1058 = call "档位加载比例 (子VI).vi"("更换车型加载比例"=w1847, "D1-D3/R1/R2加载比例"=w1848) -> ("数值"=w1849:dbl)  [unwired: 9 in]
                }
                n1059 = Index Array(array=w1845) -> (element #1=w1835:dbl, element #2=w1834:dbl, element #3=w1833:dbl, element #4=w1832:dbl, element #5=w1831:dbl, element #6=w1830:dbl, element #7=w1829:dbl, element #8=w1828:dbl, element #9=w1827:dbl)  [unwired: 9 in]
                n1060 = local write "D2扭矩给定"(w1834) -> ()
                n1061 = local write "D3扭矩给定"(w1833) -> ()
                n1062 = local write "R1扭矩给定"(w1829) -> ()
                n1063 = local write "R2扭矩给定"(w1828) -> ()
                n1064 = local write "D1扭矩给定"(w1835) -> ()
                n1065 = local write "R3扭矩给定"(w1827) -> ()
                n1066 = local write "D4扭矩给定"(w1832) -> ()
                n1067 = local write "D5扭矩给定"(w1831) -> ()
                n1068 = local write "D6扭矩给定"(w1830) -> ()
              }
              frame 3 {
                n1069 = local read "D1"() -> (w1868:dbl)
                n1070 = local read "D2"() -> (w1867:dbl)
                n1071 = local read "D3"() -> (w1866:dbl)
                n1072 = local read "D4"() -> (w1865:dbl)
                n1073 = local read "D5"() -> (w1864:dbl)
                n1074 = local read "D6"() -> (w1863:dbl)
                n1075 = local read "R1"() -> (w1862:dbl)
                n1076 = local read "R2"() -> (w1861:dbl)
                n1077 = local read "R3"() -> (w1860:dbl)
                n1078 = local read "SG18-3百分比"() -> (w1850:dbl)
                n1079 = Build Array(w1868, w1867, w1866, w1865, w1864, w1863, w1862, w1861, w1860) -> (w1870:dbl[])
                n1080 = for {
                  tunnel: w1870 -> [w1872] mode=indexing
                  tunnel: [w1873] -> w1869 mode=indexing
                  tunnel: w1850 -> [w1871]
                  n1081 = call "档位加载比例 (子VI).vi"("更换车型加载比例"=w1871, "D1-D3/R1/R2加载比例"=w1872) -> ("数值"=w1873:dbl)  [unwired: 9 in]
                }
                n1082 = Index Array(array=w1869) -> (element #1=w1859:dbl, element #2=w1858:dbl, element #3=w1857:dbl, element #4=w1856:dbl, element #5=w1855:dbl, element #6=w1854:dbl, element #7=w1853:dbl, element #8=w1852:dbl, element #9=w1851:dbl)  [unwired: 9 in]
                n1083 = local write "D4扭矩给定"(w1856) -> ()
                n1084 = local write "D5扭矩给定"(w1855) -> ()
                n1085 = local write "D6扭矩给定"(w1854) -> ()
                n1086 = local write "R1扭矩给定"(w1853) -> ()
                n1087 = local write "R2扭矩给定"(w1852) -> ()
                n1088 = local write "D2扭矩给定"(w1858) -> ()
                n1089 = local write "D3扭矩给定"(w1857) -> ()
                n1090 = local write "R3扭矩给定"(w1851) -> ()
                n1091 = local write "D1扭矩给定"(w1859) -> ()
              }
            }
            n1092 = for {
              N: 8 -> [_]
              tunnel: w1754 -> [w1777] mode=indexing
              tunnel: [w1776] -> w1753 mode=indexing
              n1093 = call "温度标定.vi"("输入电压"=w1777) -> ("输出温度"=w1776:dbl)  [unwired: 10 in]
            }
            n1094 = Index Array(array=w1753) -> (element #1=→"前左滚筒左轴承":dbl, element #2=→"前左滚筒右轴承":dbl, element #3=→"前左电机左轴承":dbl, element #4=→"前左电机右轴承":dbl, element #5=→"前左电机绕组" →"前左":dbl, element #6=→"前右滚筒左轴承":dbl, element #7=→"前左滚筒右轴承":dbl, element #8=→"前右滚筒左轴承":dbl)  [unwired: 8 in]
            n1095 = for {
              N: 8 -> [_]
              tunnel: w1743 -> [w1775] mode=indexing
              tunnel: [w1774] -> w1745 mode=indexing
              n1096 = call "温度标定.vi"("输入电压"=w1775) -> ("输出温度"=w1774:dbl)  [unwired: 10 in]
            }
            n1097 = Index Array(array=w1745) -> (element #1=→"前右电机右轴承":dbl, element #2=→"前右电机绕组" →"前右":dbl, element #3=→"中左滚筒左轴承":dbl, element #4=→"中左滚筒右轴承":dbl, element #5=→"中左电机左轴承":dbl, element #6=→"中左电机右轴承":dbl, element #7=→"中左电机绕组" →"中左":dbl, element #8=→"中右滚筒左轴承":dbl)  [unwired: 8 in]
            n1098 = local read "输出数组右"() -> (w1719:dbl[][])
            n1099 = Index Array(array=w1719) -> (element #1=w1718:dbl[], element #2=w1680:dbl[], element #3=w1705:dbl[], element #4=w1692:dbl[])  [unwired: 8 in]
            n1100 = for {
              N: 8 -> [_]
              tunnel: w1734 -> [w1773] mode=indexing
              tunnel: [w1772] -> w1735 mode=indexing
              n1101 = call "温度标定.vi"("输入电压"=w1773) -> ("输出温度"=w1772:dbl)  [unwired: 10 in]
            }
            n1102 = Index Array(array=w1718) -> (element #1=w1717:dbl, element #2=w1716:dbl, element #3=w1714:dbl, element #4=w1713:dbl, element #5=w1712:dbl, element #6=w1711:dbl, element #7=w1710:dbl, element #8=w1709:dbl)  [unwired: 8 in]
            n1103 = Build Array(w1714, w1713, w1712, w1711, w1710, w1709) -> (w1671:dbl[])
            n1104 = Index Array(array=w1671, index=2 ("索引")) -> (element=w1668:dbl)
            n1105 = call "泵压力标定.vi"("振动泵信号输入"=w1717) -> ("振动泵压力输出"=w1704:dbl)  [unwired: 10 in]
            n1106 = Subtract(x=w1668, y=0.0) -> (x-y=→"中左电机左轴承振动":dbl)
            n1107 = for {
              N: 6 -> [_]
              tunnel: w1671 -> [w1769] mode=indexing
              tunnel: [w1769] -> w1708 mode=indexing
            }
            n1108 = Index Array(array=w1735) -> (element #1=→"中右滚筒右轴承":dbl, element #2=→"中右电机左轴承":dbl, element #3=→"中右电机右轴承":dbl, element #4=→"中右电机绕组" →"中右":dbl, element #5=→"后左滚筒左轴承":dbl, element #6=→"后左滚筒右轴承":dbl, element #7=→"后左电机左轴承":dbl, element #8=→"后左电机右轴承":dbl)  [unwired: 8 in]
            n1109 = call "泵压力标定.vi"("振动泵信号输入"=w1716) -> ("振动泵压力输出"=w1701:dbl)  [unwired: 10 in]
            n1110 = Index Array(array=w1708) -> (element #1=w1570:dbl, element #2=w1568:dbl, element #4=w1565:dbl, element #5=w1562:dbl, element #6=w1559:dbl)  [unwired: 6 in, 1 out]
            n1111 = Divide(x=w1704, y=10.0) -> (x/y=→"振动泵压力":dbl)
            n1112 = Divide(x=w1701, y=10.0) -> (x/y=→"转向泵压力":dbl)
            n1113 = Add(x=w1570, y=920.0) -> (x+y=→"中左滚筒左轴承振动":dbl)
            n1114 = Add(x=w1568, y=1000.0) -> (x+y=→"中左滚筒右轴承振动":dbl)
            n1115 = Add(x=w1565, y=1000.0) -> (x+y=→"中左电机右轴承振动":dbl)
            n1116 = for {
              N: 8 -> [_]
              tunnel: w1724 -> [w1771] mode=indexing
              tunnel: [w1770] -> w1726 mode=indexing
              n1117 = call "温度标定.vi"("输入电压"=w1771) -> ("输出温度"=w1770:dbl)  [unwired: 10 in]
            }
            n1118 = Add(x=w1562, y=1000.0) -> (x+y=→"中右滚筒左振动":dbl)
            n1119 = Add(x=w1559, y=1000.0) -> (x+y=→"中右滚筒右振动":dbl)
            n1120 = Index Array(array=w1680, index #1=1 ("索引"), index #2=4 ("索引")) -> (element #1=w1677:dbl, element #2=w1673:dbl)
            n1121 = for {
              N: 8 -> [_]
              tunnel: w1680 -> [w1768] mode=indexing
              tunnel: [w1768] -> w1706 mode=indexing
            }
            n1122 = Index Array(array=w1726) -> (element #1=→"后左电机绕组" →"后左":dbl, element #2=→"后右滚筒左轴承":dbl, element #3=→"后左滚筒右轴承":dbl, element #4=→"后右滚筒左轴承":dbl, element #5=→"后右电机右轴承":dbl, element #6=→"后右电机绕组" →"后右":dbl)  [unwired: 6 in]
            n1123 = Subtract(x=w1673, y=0.0) -> (x-y=→"后左电机左振动":dbl)
            n1124 = Subtract(x=w1677, y=0.0) -> (x-y=→"中右电机右振动":dbl)
            n1125 = Index Array(array=w1706) -> (element #1=w1550:dbl, element #3=w1556:dbl, element #4=w1553:dbl, element #6=w1583:dbl, element #7=w1580:dbl, element #8=w1577:dbl)  [unwired: 8 in, 2 out]
            n1126 = Index Array(array=w1705) -> (element #1=w1574:dbl, element #2=w1683:dbl, element #3=w1593:dbl, element #4=w1591:dbl, element #5=w1589:dbl, element #6=w1588:dbl, element #7=w1586:dbl, element #8=→"前左滚筒左轴承振动":dbl)  [unwired: 8 in]
            n1127 = Add(x=w1583, y=1000.0) -> (x+y=→"后左电机右振动":dbl)
            n1128 = Add(x=w1550, y=1000.0) -> (x+y=→"中右电机左振动":dbl)
            n1129 = Add(x=w1577, y=1000.0) -> (x+y=→"后右滚筒右振动":dbl)
            n1130 = Add(x=w1580, y=950.0) -> (x+y=→"后右滚筒左振动":dbl)
            n1131 = Add(x=w1556, y=1000.0) -> (x+y=→"后左滚筒左振动":dbl)
            n1132 = Add(x=w1553, y=1000.0) -> (x+y=→"后左滚筒右振动":dbl)
            n1133 = for {
              tunnel: w1692 -> [w1767] mode=indexing
              tunnel: [w1767] -> w1691 mode=indexing
            }
            n1134 = Subtract(x=w1683, y=0.0) -> (x-y=→"后右电机右振动":dbl)
            n1135 = call "变矩器及前轮左右温度标定.vi"("变矩器，前轮左和右信号输入"=w1588) -> ("变矩器，前轮左和右信号输出"=→"右前轮轴承温度标定":dbl)  [unwired: 10 in]
            n1136 = call "温度标定.vi"("输入电压"=w1586) -> ("输出温度"=→"左前轮轴承温度标定":dbl)  [unwired: 10 in]
            n1137 = call "温度标定.vi"("输入电压"=w1589) -> ("输出温度"=→"变矩器出口温度标定":dbl)  [unwired: 10 in]
            n1138 = call "温度标定.vi"("输入电压"=w1591) -> ("输出温度"=→"液压油箱温度标定":dbl)  [unwired: 10 in]
            n1139 = call "环境温度标定.vi"("环境温度信号输入"=w1593) -> ("环境温度输出"=→"环境温度标定":dbl)  [unwired: 10 in]
            n1140 = Add(x=w1574, y=900.0) -> (x+y=→"后右电机左振动":dbl)
            n1141 = Index Array(array=w1691) -> (element #1=→"前左滚筒右轴承振动":dbl, element #2=→"前左电机左轴承振动":dbl, element #3=→"前左电机右轴承振动":dbl, element #4=→"前右滚筒左轴承振动":dbl, element #5=→"前右滚筒右轴承振动":dbl, element #6=→"前右电机左轴承振动":dbl, element #7=→"前右电机右轴承振动":dbl)  [unwired: 8 in, 1 out]
            n1142 = local read "中右电机绕组"() -> (w1662:dbl)
            n1143 = local read "中左电机绕组"() -> (w1656:dbl)
            n1144 = local read "前右电机绕组"() -> (w1651:dbl)
            n1145 = local read "前左电机绕组"() -> (w1646:dbl)
            n1146 = local read "后左滚筒右轴承"() -> (w1666:dbl)
            n1147 = local read "后左滚筒左轴承"() -> (w1665:dbl)
            n1148 = local read "后左电机右轴承"() -> (w1664:dbl)
            n1149 = local read "后左电机左轴承"() -> (w1663:dbl)
            n1150 = local read "液压油箱温度标定"() -> (w1643:dbl)
            n1151 = local read "变矩器出口温度标定"() -> (w1642:dbl)
            n1152 = local read "右前轮轴承温度标定"() -> (w1641:dbl)
            n1153 = local read "中右电机右轴承"() -> (w1661:dbl)
            n1154 = local read "中右电机左轴承"() -> (w1660:dbl)
            n1155 = local read "中右滚筒右轴承"() -> (w1659:dbl)
            n1156 = local read "中右滚筒左轴承"() -> (w1658:dbl)
            n1157 = local read "前右滚筒左轴承"() -> (w1657:dbl)
            n1158 = local read "中左电机右轴承"() -> (w1655:dbl)
            n1159 = local read "中左电机左轴承"() -> (w1654:dbl)
            n1160 = local read "中左滚筒左轴承"() -> (w1653:dbl)
            n1161 = local read "中左滚筒右轴承"() -> (w1652:dbl)
            n1162 = local read "前右电机右轴承"() -> (w1650:dbl)
            n1163 = local read "前左滚筒右轴承"() -> (w1649:dbl)
            n1164 = local read "前右滚筒左轴承"() -> (w1648:dbl)
            n1165 = local read "前左电机左轴承"() -> (w1647:dbl)
            n1166 = local read "前左电机右轴承"() -> (w1645:dbl)
            n1167 = local read "前左滚筒左轴承"() -> (w1644:dbl)
            n1168 = local read "左前轮轴承温度标定"() -> (w1600:dbl)
            n1169 = local read "前左滚筒右轴承"() -> (w1598:dbl)
            n1170 = local read "前左"() -> (w1640:dbl)
            n1171 = local read "中左"() -> (w1639:dbl)
            n1172 = local read "后右"() -> (w1638:dbl)
            n1173 = local read "后左"() -> (w1637:dbl)
            n1174 = local read "后右"() -> (w1636:dbl)
            n1175 = local read "中右"() -> (w1635:dbl)
            n1176 = Build Array(w1666, w1665, w1664, w1663, w1662, w1661, w1660, w1659, w1658, w1657, w1656, w1655, w1654, w1653, w1652, w1651, w1650, w1649, w1648, w1647, w1646, w1645, w1644, w1643, w1642, w1641, w1640, w1639, w1638, w1637, w1636, w1635, w1600, w1598) -> (w1634:dbl[])
            n1177 = for {
              tunnel: w1634 -> [w1766] mode=indexing
              tunnel: [w1765] -> w1633 mode=indexing
              n1178 = call "报警判断 (子VI).vi"("后左滚筒右轴承"=w1766) -> ("布尔"=w1765:bool)  [unwired: 10 in]
            }
            n1179 = Index Array(array=w1633) -> (element #1=w1632:bool, element #2=w1631:bool, element #3=w1630:bool, element #4=w1629:bool, element #5=w1628:bool, element #6=w1627:bool, element #7=w1626:bool, element #8=w1625:bool, element #9=w1624:bool, element #10=w1623:bool, element #11=w1622:bool, element #12=w1621:bool, element #13=w1620:bool, element #14=w1619:bool, element #15=w1618:bool, element #16=w1617:bool, element #17=w1616:bool, element #18=w1615:bool, element #19=w1614:bool, element #20=w1613:bool, element #21=w1612:bool, element #22=w1611:bool, element #23=w1610:bool, element #24=w1609:bool, element #25=w1608:bool, element #26=w1607:bool, element #27=w1606:bool, element #28=w1605:bool, element #29=w1604:bool, element #30=w1603:bool, element #31=w1602:bool, element #32=w1601:bool, element #33=w1599:bool, element #34=w1597:bool)  [unwired: 34 in]
            n1180 = Compound Arithmetic op=OR ("复合运算")(w1632, w1631, w1630, w1629, w1628, w1627, w1626, w1625, w1624, w1623, w1622, w1621, w1620, w1619, w1618, w1617, w1616, w1615, w1614, w1613, w1612, w1611, w1610, w1609, w1608, w1607, w1606, w1605, w1604, w1603, w1602, w1601, w1599, w1597) -> (w1594:bool)
            n1181 = case shown="真" w1594 {
              frame False {
                n1182 = local write "超温报警"(FALSE ("超温报警")) -> ()
              }
              frame True {
                "超温报警" <- TRUE ("超温报警")
              }
            }
            n1183 = call <vilib>:"Boolean Crossing PtByPt.vi"("direction"=enum16{"either", "false-true", "true-false"}."false-true", "input"=w1594) -> ("crossing"=w1596:bool)  [unwired: 1 in]
            n1184 = case shown="真" w1596 {
              frame False {
              }
              frame True {
                "对话框传递" <- TRUE ("对话框传递")
              }
            }
          }
          frame "退出" {
          }
        }
      }
    }
    frame #2 {
    }
  }
  n1185 = while "主线程" {
    shift-right: [w2218] -> _
    shift-left: enum16{"Init", "Wait", "Run", "Exit"}."Init" -> [w2208]
    shift-right: [w2219] -> _
    shift-left: _ -> [w2220]
    shift-right: [w2217] -> _
    shift-left: _ -> [w2216]
    shift-right: [w2215] -> _
    shift-left: _ -> [w2214]
    shift-right: [w2213] -> _
    shift-left: _ -> [w2212]
    shift-right: [w2210] -> _
    shift-left: u32 0 -> [w2211]
    tunnel: [w2209] -> w4
    stop <- w2206 stop-if-true
    # "CAN Status"
    # "Config"
    # "EventReg"
    # "UpdateUIEvent"
    # "SendCnt"
    n1186 = Equal?(x=w2208, y=enum16{"Init", "Wait", "Run", "Exit"}."Exit") -> (x = y?=w2206:bool)
    n1187 = case shown="\"Init\", 默认" w2208 {
      tunnel: w2220 -> [_ w2252 w2362 w2632]
      tunnel: [w2243 w2251 w2361 w2632] -> w2219
      tunnel: [enum16{"Init", "Wait", "Run", "Exit"}."Wait" w2248 w2363 enum16{"Init", "Wait", "Run", "Exit"}."Exit"] -> w2218
      tunnel: [w2239 w2249 w2360 w2630] -> w2217
      tunnel: w2216 -> [_ w2250 w2360 w2630]
      tunnel: [w2231 w2247 w2358 w2635] -> w2215
      tunnel: w2214 -> [_ w2247 w2359 w2635]
      tunnel: [w2230 w2246 w2357 w2633] -> w2213
      tunnel: w2212 -> [_ w2246 w2357 w2633]
      tunnel: w2211 -> [w2228 w2245 w2356 w2628]
      tunnel: [w2228 w2245 w2355 w2628] -> w2210
      tunnel: [_ _ _ errorcluster {"status"=FALSE, "code"=0, "source"=""} ("error constant")] -> w2209
      frame "Init", Default {
        w2232 = cluster{"CANOpen":bool} {"CANOpen"=FALSE}  # UpdateUI
        w2242 = T9 {"DevType"=2, "DevIndex"=0, "CanIndex"=0, "VCI_INIT_CONFIG"={"AccCode"=0, "AccMask"=0, "InitFlag"=0, "Fliter"=0, "Timing0"=0, "Timing1"=0, "Mode"=0}}  # Config
        w2243 = cluster{"Open":bool, "SendCnt":u32} {"Open"=FALSE, "SendCnt"=0}  # CAN Status
        n1188 = local write "comcnt"(u16 0 ("comcnt")) -> ()
        n1189 = local write "停止"(FALSE ("停止")) -> ()
        n1190 = local write "Open"(FALSE ("Open")) -> ()
        n1191 = property class="VI"("Front Panel.Closeable"=TRUE ("前面板窗口:可关闭")) -> ()  [unwired: 2 in, 2 out]
        n1192 = call "Demo_GetT0T1.vi"("kBaudRate"="kBaudRate") -> ("Timing0"=w2225:u8, "Timing1"=w2224:u8)
        n1193 = Bundle By Name(cluster=w2242, "DevType"="DevType", "CanIndex"="Channel", "VCI_INIT_CONFIG.AccCode"="AccCode", "VCI_INIT_CONFIG.AccMask"="AccMask", "VCI_INIT_CONFIG.InitFlag"="InitFlag", "VCI_INIT_CONFIG.Fliter"="Fliter", "VCI_INIT_CONFIG.Timing0"=w2225, "VCI_INIT_CONFIG.Timing1"=w2224, "VCI_INIT_CONFIG.Mode"="Mode") -> (w2239:T9)
        n1194 = local write "RcvEnable"(TRUE ("RcvEnable")) -> ()
        n1195 = Create User Event(user event datatype=w2232) -> (user event=w2230:refnum<user-event>)  [unwired: 1 in, 1 out]
        n1196 = register-events(w2230) -> (reference out=w2231:refnum<event-registration>)  [unwired: 2 in, 1 out]
        "Config" <- w2242
      }
      frame "Wait" {
        n1197 = event shown="[10] 超时" {
          selector: _ -> [_ _ _ _ _ _ _ _ _ _ _]
          dyn-events: _ -> [_ _ _ _ _ _ _ _ _ _ _]
          timeout: 50 -> [_ _ _ _ _ _ _ _ _ _ _]
          tunnel: w2252 -> [w2256 w2310 w2313 w2318 w2323 w2328 w2333 w2338 w2345 w2350 w2353]
          tunnel: [w2255 w2310 w2313 w2318 w2323 w2328 w2333 w2338 w2345 w2350 w2353] -> w2251
          tunnel: w2250 -> [w2258 w2309 w2312 w2317 w2322 w2327 w2332 w2337 w2344 w2349 w2352]
          tunnel: [w2258 w2308 w2312 w2315 w2320 w2325 w2330 w2335 w2343 w2347 w2352] -> w2249
          tunnel: [w2257 enum16{"Init", "Wait", "Run", "Exit"}."Wait" enum16{"Init", "Wait", "Run", "Exit"}."Exit" enum16{"Init", "Wait", "Run", "Exit"}."Wait" enum16{"Init", "Wait", "Run", "Exit"}."Wait" enum16{"Init", "Wait", "Run", "Exit"}."Wait" enum16{"Init", "Wait", "Run", "Exit"}."Wait" enum16{"Init", "Wait", "Run", "Exit"}."Wait" enum16{"Init", "Wait", "Run", "Exit"}."Wait" enum16{"Init", "Wait", "Run", "Exit"}."Wait" enum16{"Init", "Wait", "Run", "Exit"}."Wait"] -> w2248
          tunnel: w2246 -> [w2254 _ _ _ _ _ _ _ _ _ _]
          event Menu Selection (User) {
            n1198 = event-data() -> ("ItemTag"=w2253:string)  [unwired: 8 out]
            n1199 = case shown="\"遥控器\"" w2253 {
              tunnel: w2258 -> [_ w2274]
              tunnel: [enum16{"Init", "Wait", "Run", "Exit"}."Wait" w2265] -> w2257
              tunnel: w2256 -> [w2260 w2264]
              tunnel: [w2260 w2263] -> w2255
              tunnel: w2254 -> [_ w2262]
              frame "假", Default {
              }
              frame "遥控器" {
                w2268 = T21 1 items=["OK"=1, "ERROR1"=0, "ERROR2"=-1] ("y")
                # "打开CAN的步骤：\n1.Open\n2.Init\n3.Start"
                n1200 = Unbundle By Name(w2274) -> ("DevType"=w2273:T3, "DevIndex"=w2272:u32)
                n1201 = call "VCI_OpenDevice.vi"("DevIndex"=w2272, "DevType"=w2273) -> ("error out"=w2269:errorcluster, "Return Val"=w2271:T21)  [unwired: 2 in, 6 out]
                n1202 = Equal?(x=w2271, y=w2268) -> (x = y?=w2270:bool)
                n1203 = case shown="真" w2270 {
                  tunnel: w2269 -> [_ w2289]
                  tunnel: w2274 -> [_ w2288]
                  tunnel: w2268 -> [_ w2280]
                  tunnel: [_ w2279] -> w2261
                  frame False {
                  }
                  frame True {
                    n1204 = Unbundle By Name(w2288) -> ("VCI_INIT_CONFIG"=w2287:T5, "DevType"=w2283:T3, "DevIndex"=w2282:u32, "CanIndex"=w2281:T4)
                    n1205 = call "VCI_InitCAN.vi"("VCI_INIT_CONFIG"=w2287, "error in (no error)"=w2289, "CANIndex"=w2281, "DevIndex"=w2282, "DevType"=w2283) -> ("error out"=w2284:errorcluster, "Return Val"=w2286:T21)  [unwired: 5 out]
                    n1206 = Equal?(x=w2280, y=w2286) -> (x = y?=w2285:bool)
                    n1207 = case shown="真" w2285 {
                      tunnel: w2284 -> [_ w2300]
                      tunnel: w2283 -> [_ w2299]
                      tunnel: w2282 -> [_ w2298]
                      tunnel: w2281 -> [_ w2297]
                      tunnel: w2280 -> [_ w2295]
                      tunnel: [_ w2291] -> w2279
                      frame False {
                      }
                      frame True {
                        n1208 = call "VCI_StartCAN.vi"("error in (no error)"=w2300, "CANIndex"=w2297, "DevIndex"=w2298, "DevType"=w2299) -> ("error out"=w2293:errorcluster, "Return Val"=w2296:T21)  [unwired: 6 out]
                        n1209 = Unbundle By Name(w2293) -> ("status"=w2290:bool)
                        n1210 = Equal?(x=w2295, y=w2296) -> (x = y?=w2294:bool)
                        n1211 = Not(x=w2290) -> (.not. x?=w2292:bool)
                        n1212 = And(x=w2294, y=w2292) -> (x .and. y?=w2291:bool)
                      }
                    }
                  }
                }
                n1213 = case shown="真" w2261 {
                  tunnel: w2262 -> [_ w2278]
                  tunnel: w2261 -> [_ w2276]
                  frame False {
                  }
                  frame True {
                    n1214 = Bundle By Name(cluster=cluster{"CANOpen":bool} {"CANOpen"=FALSE} ("事件数据"), "CANOpen"=w2276) -> (w2275:cluster{"CANOpen":bool})
                    n1215 = Generate User Event(user event=w2278, event data cluster=w2275) -> ()  [unwired: 2 in, 2 out]
                  }
                }
                n1216 = Select(t=enum16{"Init", "Wait", "Run", "Exit"}."Run", s=w2261, f=enum16{"Init", "Wait", "Run", "Exit"}."Wait") -> (s? t:f=w2265:enum16{"Init", "Wait", "Run", "Exit"})
                n1217 = Bundle By Name(cluster=w2264, "Open"=w2261) -> (w2263:cluster{"Open":bool, "SendCnt":u32})
              }
            }
          }
          event Value Change {
            w2306 = T3 3 items=["USB-CAN"=2, "USB-CAN2"=3] ("y")
            n1218 = event-data() -> ("NewVal"=w2307:T3)  [unwired: 1 out]
            n1219 = Equal?(x=w2307, y=w2306) -> (x = y?=w2305:bool)
            n1220 = Bundle By Name(cluster=w2309, "DevType"=w2307) -> (w2308:T9)
            n1221 = Select(t=i32[] [] ("禁用项[]"), s=w2305, f=i32[] [1] ("禁用项[]")) -> (s? t:f=w2304:i32[])
            n1222 = property on="Channel" class="Ring (严格)"("Disabled Items []"=w2304) -> ()  [unwired: 2 in, 2 out]
          }
          event "停止": Value Change {
            n1223 = event-data() -> ()  [unwired: 7 out]
          }
          event Value Change {
            n1224 = event-data() -> ("NewVal"=w2316:T4)  [unwired: 1 out]
            n1225 = Bundle By Name(cluster=w2317, "CanIndex"=w2316) -> (w2315:T9)
          }
          event "AccCode": Value Change {
            n1226 = event-data() -> ("NewVal"=w2321:u32)  [unwired: 1 out]
            n1227 = Bundle By Name(cluster=w2322, "VCI_INIT_CONFIG.AccCode"=w2321) -> (w2320:T9)
          }
          event "AccMask": Value Change {
            n1228 = event-data() -> ("NewVal"=w2326:u32)  [unwired: 1 out]
            n1229 = Bundle By Name(cluster=w2327, "VCI_INIT_CONFIG.AccMask"=w2326) -> (w2325:T9)
          }
          event Value Change {
            n1230 = event-data() -> ("NewVal"=w2331:T6)  [unwired: 1 out]
            n1231 = Bundle By Name(cluster=w2332, "VCI_INIT_CONFIG.InitFlag"=w2331) -> (w2330:T9)
          }
          event Value Change {
            n1232 = event-data() -> ("NewVal"=w2336:T8)  [unwired: 1 out]
            n1233 = Bundle By Name(cluster=w2337, "VCI_INIT_CONFIG.Mode"=w2336) -> (w2335:T9)
          }
          event "kBaudRate": Value Change {
            n1234 = event-data() -> ("NewVal"=w2341:u8)  [unwired: 1 out]
            n1235 = call "Demo_GetT0T1.vi"("kBaudRate"=w2341) -> ("Timing0"=w2340:u8, "Timing1"=w2339:u8)
            n1236 = Bundle By Name(cluster=w2344, "VCI_INIT_CONFIG.Timing0"=w2340, "VCI_INIT_CONFIG.Timing1"=w2339) -> (w2343:T9)
          }
          event Value Change {
            n1237 = event-data() -> ("NewVal"=w2348:T7)  [unwired: 1 out]
            n1238 = Bundle By Name(cluster=w2349, "VCI_INIT_CONFIG.Fliter"=w2348) -> (w2347:T9)
          }
          event Timeout {
            n1239 = event-data() -> ()  [unwired: 4 out]
          }
        }
      }
      frame "Run" {
        n1240 = event shown="[0] 超时" {
          selector: w2359 -> [_ _ _ _]
          dyn-events: [_ _ _ _] -> w2358
          timeout: 100 -> [_ _ _ _]
          tunnel: [enum16{"Init", "Wait", "Run", "Exit"}."Run" enum16{"Init", "Wait", "Run", "Exit"}."Run" enum16{"Init", "Wait", "Run", "Exit"}."Run" w2621] -> w2363
          tunnel: [w2368 w2595 w2604 w2622] -> w2361
          tunnel: w2362 -> [w2368 w2595 w2606 w2622]
          tunnel: w2360 -> [w2367 w2590 w2611 _]
          tunnel: w2357 -> [_ _ w2603 _]
          tunnel: w2356 -> [w2365 w2580 w2599 w2620]
          tunnel: [w2366 w2579 w2599 w2620] -> w2355
          event Timeout {
            n1241 = event-data() -> ()  [unwired: 4 out]
            n1242 = local read "Open"() -> (w2364:bool)
            n1243 = case shown="真" w2364 {
              tunnel: w2367 -> [_ w2385]
              tunnel: [w2370 w2384] -> w2366
              tunnel: w2365 -> [w2370 w2383]
              frame False {
              }
              frame True {
                n1244 = local read "发送左侧字符"() -> (w2372:bool)
                n1245 = case shown="假" w2372 {
                  tunnel: [w2474 w2525] -> w2382
                  tunnel: [w2472 w2524] -> w2375
                  tunnel: [w2471 w2523] -> w2374
                  tunnel: [w2468 w2522] -> w2373
                  tunnel: [w2387 w2476] -> w2371
                  frame False {
                    # "扭矩"
                    # "功率"
                    # "车速"
                    # "档位"
                    # "右侧数据"
                    n1246 = Build Array("0byte 8", "1byte 8", "2byte 8", "3byte 8", "4byte 8", "5byte 8", "6byte 8", "7byte 8") -> (w2431:u8[])
                    n1247 = Build Array("0byte 5", "1byte 5", "2byte 5", "3byte 5", "4byte 5", "5byte 5", "6byte 5", "7byte 5") -> (w2404:u8[])
                    n1248 = Build Array("0byte 6", "1byte 6", "2byte 6", "3byte 6", "4byte 6", "5byte 6", "6byte 6", "7byte 6") -> (w2413:u8[])
                    n1249 = Build Array("0byte 7", "1byte 7", "2byte 7", "3byte 7", "4byte 7", "5byte 7", "6byte 7", "7byte 7") -> (w2422:u8[])
                    n1250 = call "遥控器IP地址参数.vi"("数组"=w2404, "ID_VCU_MCU_1输入"="ID_VCU_MCU_1 5") -> ("Send"=w2391:T12)  [unwired: 9 in]
                    n1251 = call "遥控器IP地址参数.vi"("数组"=w2413, "ID_VCU_MCU_1输入"="ID_VCU_MCU_1 6") -> ("Send"=w2390:T12)  [unwired: 9 in]
                    n1252 = call "遥控器IP地址参数.vi"("数组"=w2422, "ID_VCU_MCU_1输入"="ID_VCU_MCU_2 4") -> ("Send"=w2389:T12)  [unwired: 9 in]
                    n1253 = call "遥控器IP地址参数.vi"("数组"=w2431, "ID_VCU_MCU_1输入"="ID_VCU_MCU_33 3") -> ("Send"=w2388:T12)  [unwired: 9 in]
                    n1254 = Build Array(w2391, w2390, w2389, w2388) -> (w2387:T12[])
                    n1255 = Build Array("0byte 4", "1byte 4", "2byte 4", "3byte 4", "4byte 4", "5byte 4", "6byte 4", "7byte 4") -> (w2432:u8[])
                    n1256 = Build Array("0byte", "1byte", "2byte", "3byte", "4byte", "5byte", "6byte", "7byte") -> (w2459:u8[])
                    n1257 = Build Array("0byte 2", "1byte 2", "2byte 2", "3byte 2", "4byte 2", "5byte 2", "6byte 2", "7byte 2") -> (w2450:u8[])
                    n1258 = Build Array("0byte 3", "1byte 3", "2byte 3", "3byte 3", "4byte 3", "5byte 3", "6byte 3", "7byte 3") -> (w2441:u8[])
                    n1259 = call "遥控器IP地址参数.vi"("数组"=w2459, "ID_VCU_MCU_1输入"="ID_VCU_MCU_1 2") -> ("Send"=w2474:T12)  [unwired: 9 in]
                    n1260 = call "遥控器IP地址参数.vi"("数组"=w2450, "ID_VCU_MCU_1输入"="ID_VCU_MCU_1") -> ("Send"=w2472:T12)  [unwired: 9 in]
                    n1261 = call "遥控器IP地址参数.vi"("数组"=w2441, "ID_VCU_MCU_1输入"="ID_VCU_MCU_2 2") -> ("Send"=w2471:T12)  [unwired: 9 in]
                    n1262 = call "遥控器IP地址参数.vi"("数组"=w2432, "ID_VCU_MCU_1输入"="ID_VCU_MCU_33") -> ("Send"=w2468:T12)  [unwired: 9 in]
                    "发送左侧字符" <- TRUE ("发送左侧字符")
                  }
                  frame True {
                    # "左侧字符串"
                    n1263 = Build Array("0byte 16", "1byte 16", "2byte 16", "3byte 16", "4byte 16", "5byte 16", "6byte 16", "7byte 16") -> (w2520:u8[])
                    n1264 = Build Array("0byte 13", "1byte 13", "2byte 13", "3byte 13", "4byte 13", "5byte 13", "6byte 13", "7byte 13") -> (w2493:u8[])
                    n1265 = Build Array("0byte 14", "1byte 14", "2byte 14", "3byte 14", "4byte 14", "5byte 14", "6byte 14", "7byte 14") -> (w2502:u8[])
                    n1266 = Build Array("0byte 15", "1byte 15", "2byte 15", "3byte 15", "4byte 15", "5byte 15", "6byte 15", "7byte 15") -> (w2511:u8[])
                    n1267 = call "遥控器IP地址参数.vi"("数组"=w2493, "ID_VCU_MCU_1输入"="ID_VCU_MCU_1 7") -> ("Send"=w2480:T12)  [unwired: 9 in]
                    n1268 = call "遥控器IP地址参数.vi"("数组"=w2502, "ID_VCU_MCU_1输入"="ID_VCU_MCU_1 8") -> ("Send"=w2479:T12)  [unwired: 9 in]
                    n1269 = call "遥控器IP地址参数.vi"("数组"=w2511, "ID_VCU_MCU_1输入"="ID_VCU_MCU_2 5") -> ("Send"=w2478:T12)  [unwired: 9 in]
                    n1270 = call "遥控器IP地址参数.vi"("数组"=w2520, "ID_VCU_MCU_1输入"="ID_VCU_MCU_33 4") -> ("Send"=w2477:T12)  [unwired: 9 in]
                    n1271 = Build Array(w2480, w2479, w2478, w2477) -> (w2476:T12[])
                    n1272 = Build Array("0byte 12", "1byte 12", "2byte 12", "3byte 12", "4byte 12", "5byte 12", "6byte 12", "7byte 12") -> (w2526:u8[])
                    n1273 = Build Array("0byte 9", "1byte 9", "2byte 9", "3byte 9", "4byte 9", "5byte 9", "6byte 9", "7byte 9") -> (w2553:u8[])
                    n1274 = Build Array("0byte 10", "1byte 10", "2byte 10", "3byte 10", "4byte 10", "5byte 10", "6byte 10", "7byte 10") -> (w2544:u8[])
                    n1275 = Build Array("0byte 11", "1byte 11", "2byte 11", "3byte 11", "4byte 11", "5byte 11", "6byte 11", "7byte 11") -> (w2535:u8[])
                    n1276 = flat-sequence {
                      tunnel: FALSE ("发送左侧字符") -> [w2567]
                      frame #0 {
                        n1277 = local write "发送左侧字符"(w2567) -> ()
                        n1278 = Wait (ms)(milliseconds to wait=u32 100 ("等待时间（毫秒）")) -> ()  [unwired: 1 out]
                      }
                    }
                    n1279 = call "遥控器IP地址参数.vi"("数组"=w2553, "ID_VCU_MCU_1输入"="ID_VCU_MCU_1 3") -> ("Send"=w2525:T12)  [unwired: 9 in]
                    n1280 = call "遥控器IP地址参数.vi"("数组"=w2544, "ID_VCU_MCU_1输入"="ID_VCU_MCU_1 4") -> ("Send"=w2524:T12)  [unwired: 9 in]
                    n1281 = call "遥控器IP地址参数.vi"("数组"=w2526, "ID_VCU_MCU_1输入"="ID_VCU_MCU_33 2") -> ("Send"=w2522:T12)  [unwired: 9 in]
                    n1282 = call "遥控器IP地址参数.vi"("数组"=w2535, "ID_VCU_MCU_1输入"="ID_VCU_MCU_2 3") -> ("Send"=w2523:T12)  [unwired: 9 in]
                  }
                }
                n1283 = Build Array (concatenate)(w2382, w2375, w2374, w2373, w2371) -> (w2376:T12[])
                n1284 = Unbundle By Name(w2385) -> ("DevType"=w2381:T3, "DevIndex"=w2380:u32, "CanIndex"=w2378:T4)
                n1285 = Get Date/Time In Seconds() -> (seconds since 1Jan1904=w2377:timestamp)
                n1286 = disable-structure shown="禁用" {
                  disable-tunnel: _ -> [w2575 _]
                  disable-tunnel: enum16{"接收", "发送"}."发送" ("Type") -> [w2573 _]
                  disable-tunnel: w2378 -> [w2572 _]
                  disable-tunnel: w2377 -> [w2571 _]
                  disable-tunnel: w2376 -> [w2568 _]
                  frame Disabled {
                    n1287 = Bundle By Name(cluster=T20 {"Type"=enum."发送", "Channel"=0, "Time"=timestamp(0 s since 1904-01-01), "VCI_CAN_OBJ"={"ID"=0, "TimeStamp"=0, "TimeFlag"=0, "SendType"=0, "RemoteFlag"=0, "ExternFlag"=0, "DataLen"=0, "Data"=[], "Reserved"=[]}}, "Type"=w2573, "Channel"=w2572, "Time"=w2571, "VCI_CAN_OBJ"=w2568) -> (w2570:T20)
                    n1288 = Build Array(w2570) -> (w2569:T13)
                    n1289 = Enqueue Element(queue=w2575, element=w2569) -> ()  [unwired: 1 in, 4 out]
                  }
                  frame Enabled {
                  }
                }
                n1290 = call "VCI_Transmit.vi"("Buffer"=w2376, "CANIndex"=w2378, "DevIndex"=w2380, "DevType"=w2381) -> ()  [unwired: 1 in, 7 out]
                n1291 = Increment(x=w2383) -> (x+1=w2384:u32)
                n1292 = local write "SendCnt"(w2384) -> ()
              }
            }
          }
          event "Send": Value Change {
            n1293 = event-data() -> ()  [unwired: 2 out]
            n1294 = Increment(x=w2580) -> (x+1=w2579:u32)
            "SendCnt" <- w2579
            n1295 = call "Demo_MakeData.vi"("DataString"="Data") -> ("Data"=w2585:u8[], "DataLen"=w2586:u8)  [unwired: 9 out]
            n1296 = Bundle By Name(cluster=T12 {"ID"=0, "TimeStamp"=0, "TimeFlag"=0, "SendType"=0, "RemoteFlag"=0, "ExternFlag"=0, "DataLen"=0, "Data"=[], "Reserved"=[]} ("Send"), "ID"="ID", "RemoteFlag"="Type", "ExternFlag"="Format", "DataLen"=w2586, "Data"=w2585) -> (w2577:T12)
            n1297 = Build Array(w2577) -> (w2578:T12[])
            n1298 = Get Date/Time In Seconds() -> (seconds since 1Jan1904=w2581:timestamp)
            n1299 = Unbundle By Name(w2590) -> ("DevType"=w2589:T3, "DevIndex"=w2588:u32, "CanIndex"=w2582:T4)
            n1300 = Bundle By Name(cluster=T20 {"Type"=enum."发送", "Channel"=0, "Time"=timestamp(0 s since 1904-01-01), "VCI_CAN_OBJ"={"ID"=0, "TimeStamp"=0, "TimeFlag"=0, "SendType"=0, "RemoteFlag"=0, "ExternFlag"=0, "DataLen"=0, "Data"=[], "Reserved"=[]}}, "Type"=enum16{"接收", "发送"}."发送", "Channel"=w2582, "Time"=w2581, "VCI_CAN_OBJ"=w2577) -> (w2576:T20)
            n1301 = call "VCI_Transmit.vi"("Buffer"=w2578, "CANIndex"=w2582, "DevIndex"=w2588, "DevType"=w2589) -> ()  [unwired: 1 in, 7 out]
            n1302 = disable-structure shown="禁用" {
              disable-tunnel: w2576 -> [w2598 _]
              frame Disabled {
                n1303 = Build Array(w2598) -> (w2597:T13)
                n1304 = Enqueue Element(element=w2597) -> ()  [unwired: 2 in, 4 out]
              }
              frame Enabled {
              }
            }
          }
          event "停止": Value Change {
            w2607 = T21 1 items=["OK"=1, "ERROR1"=0, "ERROR2"=-1] ("y")
            n1305 = event-data() -> ()  [unwired: 7 out]
            n1306 = Unbundle By Name(w2611) -> ("DevType"=w2610:T3, "DevIndex"=w2609:u32)
            n1307 = call "VCI_CloseDevice.vi"("DevIndex"=w2609, "DevType"=w2610) -> ("Return Val"=w2608:T21)  [unwired: 1 in, 8 out]
            n1308 = Equal?(x=w2608, y=w2607) -> (x = y?=w2605:bool)
            n1309 = Not(x=w2605) -> (.not. x?=w2601:bool)
            n1310 = Bundle By Name(cluster=cluster{"CANOpen":bool} {"CANOpen"=FALSE} ("事件数据"), "CANOpen"=w2601) -> (w2600:cluster{"CANOpen":bool})
            n1311 = Bundle By Name(cluster=w2606, "Open"=w2601) -> (w2604:cluster{"Open":bool, "SendCnt":u32})
            n1312 = local write "Open"(w2601) -> ()
            n1313 = Generate User Event(user event=w2603, event data cluster=w2600) -> ()  [unwired: 2 in, 2 out]
          }
          event User Event {
            w2617 = 0
            w2616 = 2
            n1314 = event-data() -> ("CANOpen"=w2619:bool)  [unwired: 1 out]
            "Open" <- w2619
            n1315 = disable-structure shown="禁用" {
              disable-tunnel: w2619 -> [w2624 _]
              frame Disabled {
                n1316 = Not(x=w2624) -> (.not. x?=w2623:bool)
                n1317 = property class="VI"("Front Panel.Closeable"=w2623) -> ()  [unwired: 2 in, 2 out]
              }
              frame Enabled {
              }
            }
            n1318 = Select(t=w2616, s=w2619, f=w2617) -> (s? t:f=w2618:i32)
            n1319 = Select(t=w2617, s=w2619, f=w2616) -> (s? t:f=w2613:i32)
            n1320 = Select(t=enum16{"Init", "Wait", "Run", "Exit"}."Run", s=w2619, f=enum16{"Init", "Wait", "Run", "Exit"}."Wait") -> (s? t:f=w2621:enum16{"Init", "Wait", "Run", "Exit"})
            n1321 = disable-structure shown="禁用" {
              disable-tunnel: w2618 -> [w2626 _]
              disable-tunnel: w2613 -> [w2625 _]
              frame Disabled {
                n1322 = property on="Close" class="Bool"("DisabledEnum"=w2625) -> ()  [unwired: 2 in, 2 out]
                n1323 = property on="ID" class="DigNum (严格)"("DisabledEnum"=w2625) -> ()  [unwired: 2 in, 2 out]
                n1324 = property on="Data" class="Str"("DisabledEnum"=w2625) -> ()  [unwired: 2 in, 2 out]
                n1325 = property on="Format" class="Ring (严格)"("DisabledEnum"=w2625) -> ()  [unwired: 2 in, 2 out]
                n1326 = property on="Type" class="Ring (严格)"("DisabledEnum"=w2625) -> ()  [unwired: 2 in, 2 out]
                n1327 = property on="Send" class="Bool"("DisabledEnum"=w2625) -> ()  [unwired: 2 in, 2 out]
                n1328 = property on="Clear" class="Bool"("DisabledEnum"=w2625) -> ()  [unwired: 2 in, 2 out]
                n1329 = property on="Fliter" class="Ring (严格)"("DisabledEnum"=w2626) -> ()  [unwired: 2 in, 2 out]
                n1330 = property on="DevType" class="Ring (严格)"("DisabledEnum"=w2626) -> ()  [unwired: 2 in, 2 out]
                n1331 = property on="Channel" class="Ring (严格)"("DisabledEnum"=w2626) -> ()  [unwired: 2 in, 2 out]
                n1332 = property on="AccCode" class="DigNum (严格)"("DisabledEnum"=w2626) -> ()  [unwired: 2 in, 2 out]
                n1333 = property on="AccMask" class="DigNum (严格)"("DisabledEnum"=w2626) -> ()  [unwired: 2 in, 2 out]
                n1334 = property on="InitFlag" class="Ring (严格)"("DisabledEnum"=w2626) -> ()  [unwired: 2 in, 2 out]
                n1335 = property on="Mode" class="Ring (严格)"("DisabledEnum"=w2626) -> ()  [unwired: 2 in, 2 out]
                n1336 = property on="kBaudRate" class="Ring (严格)"("DisabledEnum"=w2626) -> ()  [unwired: 2 in, 2 out]
                n1337 = property on="Open 2" class="Bool"("DisabledEnum"=w2626) -> ()  [unwired: 2 in, 2 out]
              }
              frame Enabled {
              }
            }
          }
        }
      }
      frame "Exit" {
        n1338 = Unregister For Events(event registration refnum=w2635) -> (error out=w2634:errorcluster)  [unwired: 1 in]
        n1339 = Destroy User Event(user event=w2633, error in=w2634) -> ()  [unwired: 1 out]
        n1340 = Unbundle By Name(w2632) -> ("Open"=w2631:bool)
        n1341 = local write "RcvEnable"(FALSE ("RcvEnable")) -> ()
        n1342 = case shown="真" w2631 {
          tunnel: w2630 -> [_ w2639]
          frame False {
          }
          frame True {
            n1343 = Unbundle By Name(w2639) -> ("DevType"=w2638:T3, "DevIndex"=w2637:u32)
            n1344 = call "VCI_CloseDevice.vi"("DevIndex"=w2637, "DevType"=w2638) -> ()  [unwired: 1 in, 9 out]
          }
        }
      }
    }
  }
  n1345 = flat-sequence {
    frame #0 {
      "启动布尔" <- TRUE ("启动布尔")
      "停止布尔" <- TRUE ("停止布尔")
    }
    frame #1 {
      n1346 = while {
        stop <- w2647 stop-if-true
        n1347 = local read "停止布尔"() -> (→"停止布尔 2":bool)
        n1348 = local read "当前试验档位"() -> (w2645:string)
        n1349 = local read "485启动给遥控器布尔"() -> (w2648:bool)
        n1350 = String Length(string=w2645) -> (length=w2644:i32)
        n1351 = local read "Open"() -> (w2650:bool)
        n1352 = local read "试验开始"() -> (w2642:bool)
        n1353 = Not Equal To 0?(x=w2644) -> (x != 0?=w2643:bool)
        n1354 = Not Equal?(x="无效档" ("y"), y=w2645) -> (x != y?=w2651:bool)
        n1355 = Not Equal?(x=w2645, y="N") -> (x != y?=w2652:bool)
        n1356 = Compound Arithmetic op=AND ("复合运算")(w2652, w2651, w2643, w2650, w2648, w2642) -> (w2649:bool)
        n1357 = case shown="真" w2649 {
          tunnel: w2645 -> [_ w2670]
          frame False {
          }
          frame True {
            n1358 = case shown="\"R3\"" w2670 {
              frame "D1" {
                n1359 = local write "加载电机右上转矩给定"("D1扭矩给定") -> ()
                n1360 = local write "加载电机右下转矩给定"("D1扭矩给定") -> ()
                n1361 = local write "加载电机左下转矩给定"("D1扭矩给定") -> ()
                n1362 = local write "加载电机左上转矩给定"("D1扭矩给定") -> ()
              }
              frame "D2" {
                n1363 = local write "加载电机右上转矩给定"("D2扭矩给定") -> ()
                n1364 = local write "加载电机右下转矩给定"("D2扭矩给定") -> ()
                n1365 = local write "加载电机左下转矩给定"("D2扭矩给定") -> ()
                n1366 = local write "加载电机左上转矩给定"("D2扭矩给定") -> ()
              }
              frame "D3" {
                n1367 = local write "加载电机右上转矩给定"("D3扭矩给定") -> ()
                n1368 = local write "加载电机右下转矩给定"("D3扭矩给定") -> ()
                n1369 = local write "加载电机左下转矩给定"("D3扭矩给定") -> ()
                n1370 = local write "加载电机左上转矩给定"("D3扭矩给定") -> ()
              }
              frame "D4" {
                n1371 = local write "加载电机右上转矩给定"("D4扭矩给定") -> ()
                n1372 = local write "加载电机右下转矩给定"("D4扭矩给定") -> ()
                n1373 = local write "加载电机左下转矩给定"("D4扭矩给定") -> ()
                n1374 = local write "加载电机左上转矩给定"("D4扭矩给定") -> ()
                "ini_D5" <- TRUE ("ini_D56")
              }
              frame "D5" {
                n1375 = flat-sequence {
                  frame #0 {
                    n1376 = local read "ini_D5"() -> (w2691:bool)
                    n1377 = case shown="真" w2691 {
                      frame False {
                      }
                      frame True {
                        n1378 = local write "ini_D5"(FALSE ("ini_D5")) -> ()
                        n1379 = local read "D5扭矩给定"() -> (w2694:i16)
                        n1380 = local write "加载电机左上转矩给定"(w2694) -> ()
                        n1381 = local write "加载电机左下转矩给定"(w2694) -> ()
                        n1382 = local write "加载电机右上转矩给定"(w2694) -> ()
                        n1383 = local write "加载电机右下转矩给定"(w2694) -> ()
                        n1384 = Wait (ms)(milliseconds to wait=u32 1800 ("等待时间（毫秒）")) -> ()  [unwired: 1 out]
                      }
                    }
                  }
                  frame #1 {
                    n1385 = local read "加载左上转矩监控"() -> (w2699:i16)
                    n1386 = local read "加载左下转矩监控"() -> (w2698:i16)
                    n1387 = local read "加载转矩右上监控"() -> (w2697:i16)
                    n1388 = local read "加载右下转矩监控"() -> (w2696:i16)
                    n1389 = Compound Arithmetic op=ADD(w2699, w2698, w2697, w2696) -> (w2701:i16)
                    n1390 = Not Equal To 0?(x=w2701) -> (x != 0?=w2700:bool)
                    n1391 = case shown="假" w2700 {
                      tunnel: w2699 -> [_ w2711]
                      tunnel: w2698 -> [_ w2710]
                      tunnel: w2697 -> [_ w2709]
                      tunnel: w2696 -> [_ w2708]
                      tunnel: "D5扭矩给定" -> [w2702 _]
                      frame False {
                        n1392 = local write "加载电机左上转矩给定"(w2702) -> ()
                        n1393 = local write "加载电机左下转矩给定"(w2702) -> ()
                        n1394 = local write "加载电机右上转矩给定"(w2702) -> ()
                        n1395 = local write "加载电机右下转矩给定"(w2702) -> ()
                      }
                      frame True {
                        w2707 = 0
                        n1396 = Subtract(x=w2707, y=w2711) -> (x-y=w2706:i32)
                        n1397 = Subtract(x=w2707, y=w2708) -> (x-y=w2703:i32)
                        n1398 = Subtract(x=w2707, y=w2709) -> (x-y=w2704:i32)
                        n1399 = Subtract(x=w2707, y=w2710) -> (x-y=w2705:i32)
                        n1400 = local write "加载电机左上转矩给定"(w2706) -> ()
                        n1401 = local write "加载电机右下转矩给定"(w2703) -> ()
                        n1402 = local write "加载电机右上转矩给定"(w2704) -> ()
                        n1403 = local write "加载电机左下转矩给定"(w2705) -> ()
                      }
                    }
                  }
                }
                "ini_D6" <- TRUE ("ini_D6")
              }
              frame "D6" {
                n1404 = flat-sequence {
                  frame #0 {
                    n1405 = local read "ini_D6"() -> (w2712:bool)
                    n1406 = case shown="真" w2712 {
                      frame False {
                      }
                      frame True {
                        n1407 = local read "D6扭矩给定"() -> (w2713:i16)
                        n1408 = local write "ini_D6"(FALSE ("ini_D5")) -> ()
                        n1409 = local write "加载电机左上转矩给定"(w2713) -> ()
                        n1410 = local write "加载电机左下转矩给定"(w2713) -> ()
                        n1411 = local write "加载电机右上转矩给定"(w2713) -> ()
                        n1412 = local write "加载电机右下转矩给定"(w2713) -> ()
                        n1413 = Wait (ms)(milliseconds to wait=u32 1800 ("等待时间（毫秒）")) -> ()  [unwired: 1 out]
                      }
                    }
                  }
                  frame #1 {
                    n1414 = local read "加载左上转矩监控"() -> (w2720:i16)
                    n1415 = local read "加载左下转矩监控"() -> (w2719:i16)
                    n1416 = local read "加载转矩右上监控"() -> (w2718:i16)
                    n1417 = local read "加载右下转矩监控"() -> (w2717:i16)
                    n1418 = Compound Arithmetic op=ADD(w2720, w2719, w2718, w2717) -> (w2722:i16)
                    n1419 = Not Equal To 0?(x=w2722) -> (x != 0?=w2721:bool)
                    n1420 = case shown="真" w2721 {
                      tunnel: w2720 -> [_ w2732]
                      tunnel: w2719 -> [_ w2731]
                      tunnel: w2718 -> [_ w2730]
                      tunnel: w2717 -> [_ w2729]
                      tunnel: "D6扭矩给定" -> [w2723 _]
                      frame False {
                        n1421 = local write "加载电机左上转矩给定"(w2723) -> ()
                        n1422 = local write "加载电机左下转矩给定"(w2723) -> ()
                        n1423 = local write "加载电机右上转矩给定"(w2723) -> ()
                        n1424 = local write "加载电机右下转矩给定"(w2723) -> ()
                      }
                      frame True {
                        w2728 = 0
                        n1425 = Subtract(x=w2728, y=w2732) -> (x-y=w2727:i32)
                        n1426 = Subtract(x=w2728, y=w2729) -> (x-y=w2724:i32)
                        n1427 = Subtract(x=w2728, y=w2730) -> (x-y=w2725:i32)
                        n1428 = Subtract(x=w2728, y=w2731) -> (x-y=w2726:i32)
                        n1429 = local write "加载电机左上转矩给定"(w2727) -> ()
                        n1430 = local write "加载电机右下转矩给定"(w2724) -> ()
                        n1431 = local write "加载电机右上转矩给定"(w2725) -> ()
                        n1432 = local write "加载电机左下转矩给定"(w2726) -> ()
                      }
                    }
                  }
                }
              }
              frame "R1" {
                n1433 = Multiply(x="R1扭矩给定", y=i16 -1) -> (x*y=w2733:i16)
                n1434 = local write "加载电机右上转矩给定"(w2733) -> ()
                n1435 = local write "加载电机右下转矩给定"(w2733) -> ()
                n1436 = local write "加载电机左下转矩给定"(w2733) -> ()
                n1437 = local write "加载电机左上转矩给定"(w2733) -> ()
              }
              frame "R2" {
                n1438 = Multiply(x="R2扭矩给定", y=i16 -1) -> (x*y=w2737:i16)
                n1439 = local write "加载电机右上转矩给定"(w2737) -> ()
                n1440 = local write "加载电机右下转矩给定"(w2737) -> ()
                n1441 = local write "加载电机左下转矩给定"(w2737) -> ()
                n1442 = local write "加载电机左上转矩给定"(w2737) -> ()
                "ini_R3" <- TRUE ("ini_R3")
              }
              frame "R3" {
                n1443 = flat-sequence {
                  frame #0 {
                    n1444 = local read "ini_R3"() -> (w2740:bool)
                    n1445 = case shown="真" w2740 {
                      frame False {
                      }
                      frame True {
                        n1446 = local read "R3扭矩给定"() -> (w2743:i16)
                        n1447 = local write "ini_R3"(FALSE ("ini_D5")) -> ()
                        n1448 = Multiply(x=w2743, y=i16 -1) -> (x*y=w2741:i16)
                        n1449 = local write "加载电机左上转矩给定"(w2741) -> ()
                        n1450 = local write "加载电机左下转矩给定"(w2741) -> ()
                        n1451 = local write "加载电机右上转矩给定"(w2741) -> ()
                        n1452 = local write "加载电机右下转矩给定"(w2741) -> ()
                        n1453 = Wait (ms)(milliseconds to wait=u32 1800 ("等待时间（毫秒）")) -> ()  [unwired: 1 out]
                      }
                    }
                  }
                  frame #1 {
                    n1454 = local read "加载左上转矩监控"() -> (w2752:i16)
                    n1455 = local read "加载左下转矩监控"() -> (w2751:i16)
                    n1456 = local read "加载转矩右上监控"() -> (w2750:i16)
                    n1457 = local read "加载右下转矩监控"() -> (w2749:i16)
                    n1458 = Compound Arithmetic op=ADD(w2752, w2751, w2750, w2749) -> (w2754:i16)
                    n1459 = Multiply(x="R3扭矩给定", y=i16 -1) -> (x*y=w2746:i16)
                    n1460 = Not Equal To 0?(x=w2754) -> (x != 0?=w2753:bool)
                    n1461 = case shown="假" w2753 {
                      tunnel: w2752 -> [_ w2764]
                      tunnel: w2751 -> [_ w2763]
                      tunnel: w2750 -> [_ w2762]
                      tunnel: w2749 -> [_ w2761]
                      tunnel: w2746 -> [w2755 _]
                      frame False {
                        n1462 = local write "加载电机左上转矩给定"(w2755) -> ()
                        n1463 = local write "加载电机左下转矩给定"(w2755) -> ()
                        n1464 = local write "加载电机右上转矩给定"(w2755) -> ()
                        n1465 = local write "加载电机右下转矩给定"(w2755) -> ()
                      }
                      frame True {
                        w2760 = 0
                        n1466 = Subtract(x=w2760, y=w2764) -> (x-y=w2759:i32)
                        n1467 = Subtract(x=w2760, y=w2761) -> (x-y=w2756:i32)
                        n1468 = Subtract(x=w2760, y=w2762) -> (x-y=w2757:i32)
                        n1469 = Subtract(x=w2760, y=w2763) -> (x-y=w2758:i32)
                        n1470 = local write "加载电机左上转矩给定"(w2759) -> ()
                        n1471 = local write "加载电机右下转矩给定"(w2756) -> ()
                        n1472 = local write "加载电机右上转矩给定"(w2757) -> ()
                        n1473 = local write "加载电机左下转矩给定"(w2758) -> ()
                      }
                    }
                  }
                }
              }
              frame "假", Default {
              }
            }
            n1474 = local read "启动布尔"() -> (w2669:bool)
            n1475 = case shown="真" w2669 {
              frame False {
              }
              frame True {
                n1476 = stacked-sequence {
                  frame #0 {
                    n1477 = property on="加载电机左上启动" class="Bool (严格)"("Val(Sgnl)"=TRUE ("值(信号)")) -> ()  [unwired: 2 in, 2 out]
                    n1478 = Wait (ms)(milliseconds to wait=u32 10 ("等待时间（毫秒）")) -> ()  [unwired: 1 out]
                  }
                  frame #1 {
                    n1479 = property on="加载电机左下启动" class="Bool (严格)"("Val(Sgnl)"=TRUE ("值(信号)")) -> ()  [unwired: 2 in, 2 out]
                    n1480 = Wait (ms)(milliseconds to wait=u32 10 ("等待时间（毫秒）")) -> ()  [unwired: 1 out]
                  }
                  frame #2 {
                    n1481 = property on="加载电机右上启动" class="Bool (严格)"("Val(Sgnl)"=TRUE ("值(信号)")) -> ()  [unwired: 2 in, 2 out]
                    n1482 = Wait (ms)(milliseconds to wait=u32 10 ("等待时间（毫秒）")) -> ()  [unwired: 1 out]
                  }
                  frame #3 {
                    n1483 = property on="加载电机右下启动" class="Bool (严格)"("Val(Sgnl)"=TRUE ("值(信号)")) -> ()  [unwired: 2 in, 2 out]
                    n1484 = Wait (ms)(milliseconds to wait=u32 10 ("等待时间（毫秒）")) -> ()  [unwired: 1 out]
                  }
                  frame #4 {
                    n1485 = property on="驱动电机上启动" class="Bool (严格)"("Val(Sgnl)"=TRUE ("值(信号)")) -> ()  [unwired: 2 in, 2 out]
                    n1486 = Wait (ms)(milliseconds to wait=u32 10 ("等待时间（毫秒）")) -> ()  [unwired: 1 out]
                  }
                  frame #5 {
                    n1487 = property on="驱动电机下启动" class="Bool (严格)"("Val(Sgnl)"=TRUE ("值(信号)")) -> ()  [unwired: 2 in, 2 out]
                    n1488 = Wait (ms)(milliseconds to wait=u32 10 ("等待时间（毫秒）")) -> ()  [unwired: 1 out]
                  }
                  frame #6 {
                    n1489 = local write "启动布尔"(FALSE ("启动布尔")) -> ()
                    n1490 = local write "停止布尔"(TRUE ("停止布尔")) -> ()
                  }
                }
              }
            }
          }
        }
        n1491 = case shown="\"N\"" w2645 {
          frame "假", Default {
          }
          frame "N" {
            n1492 = local read "停止布尔"() -> (w2656:bool)
            n1493 = case shown="真" w2656 {
              frame False {
              }
              frame True {
                n1494 = stacked-sequence {
                  frame #0 {
                    n1495 = local write "加载电机左上转矩给定"(i16 0 ("加载电机左上转矩给定")) -> ()
                    n1496 = Wait (ms)(milliseconds to wait=u32 10 ("等待时间（毫秒）")) -> ()  [unwired: 1 out]
                  }
                  frame #1 {
                    n1497 = local write "加载电机左下转矩给定"(i16 0 ("加载电机左下转矩给定")) -> ()
                    n1498 = Wait (ms)(milliseconds to wait=u32 10 ("等待时间（毫秒）")) -> ()  [unwired: 1 out]
                  }
                  frame #2 {
                    n1499 = local write "加载电机右上转矩给定"(i16 0 ("加载电机右上转矩给定")) -> ()
                    n1500 = Wait (ms)(milliseconds to wait=u32 10 ("等待时间（毫秒）")) -> ()  [unwired: 1 out]
                  }
                  frame #3 {
                    n1501 = local write "加载电机右下转矩给定"(i16 0 ("加载电机右下转矩给定")) -> ()
                    n1502 = Wait (ms)(milliseconds to wait=u32 10 ("等待时间（毫秒）")) -> ()  [unwired: 1 out]
                  }
                  frame #4 {
                    n1503 = Wait (ms)(milliseconds to wait=u32 10 ("等待时间（毫秒）")) -> ()  [unwired: 1 out]
                  }
                  frame #5 {
                    n1504 = Wait (ms)(milliseconds to wait=u32 10 ("等待时间（毫秒）")) -> ()  [unwired: 1 out]
                  }
                  frame #6 {
                    n1505 = local write "启动布尔"(TRUE ("启动布尔")) -> ()
                    n1506 = local write "停止布尔"(FALSE ("停止布尔")) -> ()
                  }
                }
              }
            }
          }
        }
        n1507 = local read "停止"() -> (w2647:bool)
        n1508 = Wait (ms)(milliseconds to wait=u32 50 ("等待时间（毫秒）")) -> ()  [unwired: 1 out]
      }
    }
  }
  n1509 = stacked-sequence {
    frame #0 {
      n1510 = stacked-sequence {
        frame #0 {
          w2767 = FALSE ("AD开始采集")
          n1511 = local write "AD开始采集"(w2767) -> ()
          n1512 = local write "PWM输出"(w2767) -> ()
          n1513 = local write "布尔"(FALSE ("布尔")) -> ()
          n1514 = local write "采集卡左"(FALSE ("采集卡左")) -> ()
          n1515 = local write "停止"(FALSE ("停止")) -> ()
          n1516 = local write "close"(FALSE ("close")) -> ()
        }
        frame #1 {
          n1517 = flat-sequence {
            tunnel: [w2780] -> w2777
            tunnel: [w2779] -> w2776
            tunnel: w2777 -> [w2785]
            tunnel: w2776 -> [w2784]
            tunnel: [w2783] -> w2775
            tunnel: [w2782] -> w2774
            tunnel: w2775 -> [w2792]
            tunnel: w2774 -> [w2791]
            tunnel: [w2790] -> w2773
            tunnel: [w2789] -> w2772
            tunnel: w2773 -> [w2798]
            tunnel: w2772 -> [w2797]
            tunnel: [w2796] -> w2771
            tunnel: [w2795] -> w2770
            tunnel: w2771 -> [w2802]
            tunnel: w2770 -> [w2801]
            frame #0 {
              n1518 = call "建立设备.vi"() -> ("错误输出"=w2779:errorcluster, "设备句柄"=w2780:i32)  [unwired: 10 in]
              n1519 = Wait (ms)(milliseconds to wait=u32 10 ("等待时间（毫秒）")) -> ()  [unwired: 1 out]
            }
            frame #1 {
              n1520 = Wait (ms)(milliseconds to wait=u32 10 ("等待时间（毫秒）")) -> ()  [unwired: 1 out]
              n1521 = call "建立命令连接.vi"("IP地址"="IP地址", "错误输入"=w2784, "端口号"="命令端口", "设备句柄入"=w2785) -> ("错误输出"=w2782:errorcluster, "设备句柄"=w2783:i32)  [unwired: 6 in]
            }
            frame #2 {
              n1522 = Wait (ms)(milliseconds to wait=u32 10 ("等待时间（毫秒）")) -> ()  [unwired: 1 out]
              n1523 = call "建立数据连接.vi"("错误输入"=w2791, "端口号"="数据端口", "设备句柄入"=w2792) -> ("错误输出"=w2789:errorcluster, "设备句柄"=w2790:i32)  [unwired: 7 in]
            }
            frame #3 {
              n1524 = local write "设置开关量方向"(cluster{"IO1~IO8":i8, "IO9~IO16":i8} {"IO1~IO8"=1, "IO9~IO16"=1} ("设置开关量方向")) -> ()
              n1525 = call "设置开关量方向.vi"("错误输入"=w2797, "方向"=i8[] [1, 1, 1, 1], "设备句柄入"=w2798) -> ("错误输出"=w2795:errorcluster, "设备句柄"=w2796:i32)  [unwired: 7 in]
              n1526 = Wait (ms)(milliseconds to wait=u32 10 ("等待时间（毫秒）")) -> ()  [unwired: 1 out]
            }
            frame #4 {
              n1527 = local write "错误输出"(w2801) -> ()
              "设备句柄" <- w2802
            }
          }
        }
        frame #2 {
        }
      }
    }
    frame #1 {
      n1528 = local read "错误输出"() -> (w2803:errorcluster)
      n1529 = while {
        shift-right: [w2805] -> _
        shift-left: w2803 -> [w2806]
        stop <- w2808 stop-if-true
        n1530 = local read "设备句柄"() -> (w2804:i32)
        n1531 = event shown="[1] 菜单选择(用户)" {
          selector: _ -> [_ _ _ _ _ _ _ _ _ _ _ _ _ _]
          dyn-events: _ -> [_ _ _ _ _ _ _ _ _ _ _ _ _ _]
          timeout: 100 -> [_ _ _ _ _ _ _ _ _ _ _ _ _ _]
          tunnel: w2804 -> [w2828 w2860 w2902 w2907 w2923 w2956 w2978 w2983 w2993 w3014 w3029 _ w3047 w3052]
          tunnel: w2806 -> [w2827 w2859 w2904 w2906 w2922 w2955 w2977 w2982 w2992 w3013 w3028 w3032 w3046 w3051]
          tunnel: [w2812 w2858 w2903 w2905 w2921 w2931 w2970 w2981 w2991 w2995 w3023 w3032 w3045 w3049] -> w2805
          event Timeout {
            n1532 = event-data() -> ()  [unwired: 1 in, 2 out]
            n1533 = call "得到所有通道开关量值.vi"("错误输入"=w2827, "设备句柄入"=w2828) -> ("错误输出"=w2810:errorcluster, "iStatus"=w2819:i8[], "设备句柄"=w2824:i32)  [unwired: 7 in]
            "错误输出 3" <- w2810
            n1534 = Array Subset(array=w2819, index=0 ("索引"), length=16 ("长度")) -> (w2816:i8[])
            n1535 = for {
              tunnel: w2816 -> [w2848] mode=indexing
              tunnel: [w2845] -> w2815 mode=indexing
              n1536 = Equal?(x=w2848, y=i8 1) -> (x = y?=w2846:bool)
              n1537 = case shown="假" w2846 {
                tunnel: [FALSE TRUE] -> w2845
                frame False {
                }
                frame True {
                }
              }
            }
            n1538 = Array Subset(array=w2819, index=16 ("索引"), length=8 ("长度")) -> (w2818:i8[])
            n1539 = for {
              tunnel: [w2852] -> w2817 mode=indexing
              tunnel: w2818 -> [w2851] mode=indexing
              n1540 = Equal?(x=w2851, y=i8 1) -> (x = y?=w2853:bool)
              n1541 = case shown="假" w2853 {
                tunnel: [FALSE TRUE] -> w2852
                frame False {
                }
                frame True {
                }
              }
            }
            "光隔离输入" <- w2817
            n1542 = Array To Cluster(array=w2815) -> (cluster=→"可编程数字量I/O(映射控件)--得到所有通道开关量值":T22)
            n1543 = call "读取编码器.vi"("错误输入"=w2810, "设备句柄入"=w2824) -> ("错误输出"=w2814:errorcluster, "编码器过零值"=→"编码器过零值":i16[], "编码器AB值"=→"编码器AB值":i32[], "设备句柄"=w2813:i32)  [unwired: 6 in]
            n1544 = local read "开启计数"() -> (w2811:bool)
            n1545 = case shown="真" w2811 {
              tunnel: w2814 -> [w2829 w2837]
              tunnel: w2813 -> [_ w2836]
              tunnel: [w2829 w2835] -> w2812
              frame False {
              }
              frame True {
                n1546 = call "读取所有路计数器的原码值.vi"("错误输入"=w2837, "设备句柄入"=w2836) -> ("错误输出"=w2833:errorcluster, "计数器的原码值"=w2830:u32[], "设备句柄"=w2834:i32)  [unwired: 7 in]
                n1547 = for {
                  N: 6 -> [_]
                  tunnel: w2834 -> [w2844]
                  tunnel: w2833 -> [w2843]
                  tunnel: [w2842] -> w2835
                  tunnel: [w2839] -> w2831 mode=indexing
                  tunnel: w2830 -> [w2838] mode=indexing
                  i -> [w2841]
                  n1548 = Increment(x=w2841) -> (x+1=w2840:i32)
                  n1549 = call "计数器值转换成对应的物理值.vi"("错误输入"=w2843, "ctCode"=w2838, "chNo"=w2840, "设备句柄入"=w2844) -> ("错误输出"=w2842:errorcluster, "ctValue"=w2839:dbl)  [unwired: 5 in, 1 out]
                }
                "计数/测频（Hz）值" <- w2831
              }
            }
          }
          event Menu Selection (User) {
            n1550 = event-data() -> ("ItemTag"=w2857:string)  [unwired: 1 in, 6 out]
            n1551 = case shown="\"采集卡左\"" w2857 {
              tunnel: w2860 -> [_ w2863]
              tunnel: w2859 -> [_ w2862]
              tunnel: [_ w2861] -> w2858
              frame "假", Default {
              }
              frame "采集卡左" {
                n1552 = flat-sequence {
                  tunnel: w2863 -> [w2867]
                  tunnel: w2862 -> [w2866]
                  tunnel: [w2865] -> w2864
                  tunnel: [w2901] -> w2861
                  tunnel: w2864 -> [w2901]
                  frame #0 {
                    n1553 = call "AD设置范围.vi"("错误输入"=w2866, "范围"="AD范围", "设备句柄入"=w2867) -> ("错误输出"=w2888:errorcluster, "设备句柄"=w2887:i32)  [unwired: 7 in]
                    n1554 = call "AD设置单双端.vi"("错误输入"=w2888, "单双端"="单双端", "设备句柄入"=w2887) -> ("错误输出"=w2890:errorcluster, "设备句柄"=w2889:i32)  [unwired: 7 in]
                    n1555 = call "AD设置增益.vi"("错误输入"=w2890, "增益"="增益", "设备句柄入"=w2889) -> ("错误输出"=w2897:errorcluster, "设备句柄"=w2896:i32)  [unwired: 7 in]
                    n1556 = call "AD设置通道范围.vi"("错误输入"=w2897, "起始通道"="AD起始通道", "终止通道"="AD终止通道", "设备句柄入"=w2896) -> ("错误输出"=w2891:errorcluster, "设备句柄"=w2892:i32)  [unwired: 6 in]
                    n1557 = Subtract(x="AD终止通道", y="AD起始通道") -> (x-y=w2875:i32)
                    n1558 = Increment(x=w2875) -> (x+1=w2893:i32)
                    "通道数量" <- w2893
                    n1559 = call "设定通道频率.vi"("错误输入"=w2891, "通道频率"="通道频率Hz", "设备句柄入"=w2892) -> ("错误输出"=w2879:errorcluster, "设备句柄"=w2878:i32)  [unwired: 7 in]
                    n1560 = local read "伪同步"() -> (w2884:i32)
                    n1561 = case shown="0, 默认" w2884 {
                      tunnel: "通道频率Hz" -> [w2898 _]
                      tunnel: [w2898 w2899] -> w2870
                      tunnel: "组频率Hz" -> [_ w2899]
                      frame 0, Default {
                      }
                      frame 1 {
                      }
                    }
                    n1562 = call "设定组频率.vi"("错误输入"=w2879, "组频率"="组频率Hz", "设备句柄入"=w2878) -> ("错误输出"=w2895:errorcluster, "设备句柄"=w2894:i32)  [unwired: 7 in]
                    n1563 = Divide(x=w2870, y=2.0 ("每秒刷新数据次数")) -> (x/y=w2868:dbl)
                    n1564 = To Long Integer(number=w2868) -> (32bit integer=w2873:i32)
                    n1565 = Quotient & Remainder(x=w2873, y=w2893) -> (floor(x/y)=w2872:i32)  [unwired: 1 out]
                    "每通道数据量" <- w2872
                    n1566 = Multiply(x=w2872, y=w2893) -> (x*y=→"每次总数据量":i32)
                    n1567 = call "启动采集(M系列).vi"("错误输入"=w2895, "时钟源"="时钟源", "伪同步"="伪同步", "设备句柄入"=w2894) -> ("错误输出"=w2865:errorcluster)  [unwired: 6 in, 1 out]
                  }
                  frame #1 {
                    n1568 = local write "布尔"(TRUE ("布尔")) -> ()
                  }
                }
              }
            }
          }
          event "AD停止采集": Value Change {
            n1569 = event-data() -> ()  [unwired: 1 in, 5 out]
            n1570 = call "停止采集(M).vi"("错误输入"=w2904, "设备句柄入"=w2902) -> ("错误输出"=w2903:errorcluster)  [unwired: 8 in, 1 out]
          }
          event "开启计数": Value Change {
            n1571 = event-data() -> ()  [unwired: 1 in, 5 out]
            n1572 = Initialize Array("工作方式", 6 ("维数大小")) -> (w2911:u16[])
            n1573 = call "设置所有路计数器的工作方式.vi"("错误输入"=w2906, "ctMode"=w2911, "设备句柄入"=w2907) -> ("错误输出"=w2910:errorcluster, "设备句柄"=w2909:i32)  [unwired: 7 in]
            n1574 = for {
              N: 6 -> [_]
              tunnel: w2910 -> [w2919]
              tunnel: w2909 -> [w2918]
              tunnel: [w2914] -> w2905
              i -> [w2916]
              n1575 = Increment(x=w2916) -> (x+1=w2915:i32)
              n1576 = call "设置指定通道的测频基准脉冲周期.vi"("错误输入"=w2919, "freqBase_ms"=1000.0, "chNo"=w2915, "设备句柄入"=w2918) -> ("错误输出"=w2914:errorcluster)  [unwired: 5 in, 2 out]
            }
          }
          event "计数器清零": Value Change {
            n1577 = event-data() -> ()  [unwired: 1 in, 5 out]
            n1578 = for {
              N: 6 -> [_]
              tunnel: w2923 -> [w2928]
              tunnel: w2922 -> [w2927]
              tunnel: [w2926] -> w2921
              i -> [w2925]
              n1579 = Increment(x=w2925) -> (x+1=w2924:i32)
              n1580 = call "指定通道计数器清零.vi"("错误输入"=w2927, "chNo"=w2924, "设备句柄入"=w2928) -> ("错误输出"=w2926:errorcluster)  [unwired: 7 in, 1 out]
            }
          }
          event "PWM输出": Value Change {
            n1581 = event-data() -> ("OldVal"=w2929:bool)  [unwired: 1 in, 4 out]
            n1582 = local write "PWM输出"(w2929) -> ()
            n1583 = call "设置开关量方向.vi"("错误输入"=w2955, "方向"=i8[] [1, 1], "设备句柄入"=w2956) -> ("错误输出"=w2953:errorcluster, "设备句柄"=w2954:i32)  [unwired: 7 in]
            n1584 = call "设置PWM频率和占空比.vi"("占空比(0~1)"="占空比(0~1)", "频率"="频率1", "错误输入"=w2953, "通道号"=1, "设备句柄入"=w2954) -> ("错误输出"=w2945:errorcluster, "设备句柄"=w2939:i32, "实际占空比"=→"实际占空比":dbl, "实际频率"=→"实际频率":dbl)  [unwired: 3 in]
            n1585 = call "设置PWM频率和占空比.vi"("占空比(0~1)"="占空比(0~1) 2", "频率"="频率2", "错误输入"=w2945, "通道号"=2, "设备句柄入"=w2939) -> ("错误输出"=w2938:errorcluster, "设备句柄"=w2940:i32, "实际占空比"=→"实际占空比 2":dbl, "实际频率"=→"实际频率 2":dbl)  [unwired: 3 in]
            n1586 = call "设置PWM频率和占空比.vi"("占空比(0~1)"="占空比(0~1) 3", "频率"="频率3", "错误输入"=w2938, "通道号"=3, "设备句柄入"=w2940) -> ("错误输出"=w2932:errorcluster, "设备句柄"=w2933:i32, "实际占空比"=→"实际占空比 3":dbl, "实际频率"=→"实际频率 3":dbl)  [unwired: 3 in]
            n1587 = call "使能或禁止PWM输出.vi"("错误输入"=w2932, "所用PWM使能"=i8 1, "设备句柄入"=w2933) -> ("错误输出"=w2931:errorcluster)  [unwired: 7 in, 1 out]
          }
          event "M系列PWM输出": Value Change {
            w2965 = 2 ("通道号")
            w2960 = 0.5 ("占空比(0~1)")
            w2961 = 2000.0 ("频率")
            w2973 = 1 ("通道号")
            n1588 = event-data() -> ()  [unwired: 1 in, 5 out]
            n1589 = call "设置开关量方向.vi"("错误输入"=w2977, "方向"=i8[] [1, 1], "设备句柄入"=w2978) -> ("错误输出"=w2975:errorcluster, "设备句柄"=w2976:i32)  [unwired: 7 in]
            n1590 = call "设置PWM频率和占空比.vi"("占空比(0~1)"=w2960, "频率"=w2961, "错误输入"=w2975, "通道号"=w2973, "设备句柄入"=w2976) -> ("错误输出"=w2971:errorcluster, "设备句柄"=w2974:i32)  [unwired: 3 in, 2 out]
            n1591 = call "设定输出脉冲个数.vi"("错误输入"=w2971, "脉冲个数"="设定输出脉冲个数", "通道号"=w2973, "设备句柄入"=w2974) -> ("错误输出"=w2963:errorcluster, "设备句柄"=w2962:i32)  [unwired: 2 in]
            n1592 = call "设置PWM频率和占空比.vi"("占空比(0~1)"=w2960, "频率"=w2961, "错误输入"=w2963, "通道号"=w2965, "设备句柄入"=w2962) -> ("错误输出"=w2964:errorcluster, "设备句柄"=w2966:i32)  [unwired: 3 in, 2 out]
            n1593 = call "设定输出脉冲个数.vi"("错误输入"=w2964, "通道号"=w2965, "设备句柄入"=w2966) -> ("错误输出"=w2958:errorcluster, "设备句柄"=w2959:i32)  [unwired: 3 in]
            n1594 = call "使能或禁止PWM输出(只支持EM9636M).vi"("错误输入"=w2958, "相位设置数组"=i8[] [1, 0, 0] ("PWM使能"), "PWM使能"=i8[] [1, 1, 0], "设备句柄入"=w2959) -> ("错误输出"=w2970:errorcluster)  [unwired: 6 in, 1 out]
          }
          event "设置开关量方向": Value Change {
            n1595 = event-data() -> ()  [unwired: 1 in, 5 out]
            n1596 = Cluster To Array(cluster="设置开关量方向") -> (array=w2979:i8[])
            "数组 4" <- w2979
            n1597 = call "设置开关量方向.vi"("错误输入"=w2982, "方向"=w2979, "设备句柄入"=w2983) -> ("错误输出"=w2981:errorcluster)  [unwired: 7 in, 1 out]
          }
          event "光隔离输出", "可编程数字量I/O": Value Change {
            n1598 = event-data() -> ()  [unwired: 1 in, 5 out]
            n1599 = local read "光隔离输入"() -> (w2990:bool[])
            n1600 = Cluster To Array(cluster="可编程数字量I/O") -> (array=w2984:bool[])
            n1601 = Build Array (concatenate)(w2984, w2990, "光隔离输出") -> (w2988:bool[])
            n1602 = Boolean To (0,1)(Boolean=w2988) -> (0, 1=w2987:i16[])
            n1603 = To Byte Integer(number=w2987) -> (8bit integer=w2986:i8[])
            n1604 = call "设置所有通道开关量值.vi"("错误输入"=w2992, "oStatus"=w2986, "设备句柄入"=w2993) -> ("错误输出"=w2991:errorcluster)  [unwired: 7 in, 1 out]
          }
          event "DA输出", "CH1", "CH2", "CH3", "CH4": Value Change {
            n1605 = event-data() -> ()  [unwired: 1 in, 5 out]
            n1606 = for {
              N: 4 -> [_]
              tunnel: w3014 -> [w3022]
              tunnel: w3013 -> [w3021]
              tunnel: "DA输出范围" -> [w3017]
              tunnel: [w3016] -> w3011
              tunnel: [w3015] -> w3010
              i -> [w3019]
              n1607 = Increment(x=w3019) -> (x+1=w3020:i32)
              n1608 = call "DA输出方式.vi"("输出范围"=w3017, "错误输入"=w3021, "输出值方式"=i16 1, "通道号"=w3020, "设备句柄入"=w3022) -> ("错误输出"=w3016:errorcluster, "设备句柄"=w3015:i32)  [unwired: 5 in]
            }
            n1609 = call "设置DA输出值.vi"("错误输入"=w3011, "输出值"="CH1", "通道号"=1, "设备句柄入"=w3010) -> ("错误输出"=w3004:errorcluster, "设备句柄"=w3006:i32)  [unwired: 6 in]
            n1610 = call "设置DA输出值.vi"("错误输入"=w3004, "输出值"="CH2", "通道号"=2, "设备句柄入"=w3006) -> ("错误输出"=w2998:errorcluster, "设备句柄"=w3003:i32)  [unwired: 6 in]
            n1611 = call "设置DA输出值.vi"("错误输入"=w2998, "输出值"="CH3", "通道号"=3, "设备句柄入"=w3003) -> ("错误输出"=w2997:errorcluster, "设备句柄"=w3002:i32)  [unwired: 6 in]
            n1612 = call "设置DA输出值.vi"("错误输入"=w2997, "输出值"="CH4", "通道号"=4, "设备句柄入"=w3002) -> ("错误输出"=w2995:errorcluster)  [unwired: 6 in, 1 out]
          }
          event "编码器清零": Value Change {
            n1613 = event-data() -> ()  [unwired: 1 in, 5 out]
            n1614 = call "编码器清零.vi"("错误输入"=w3028, "通道号"=1, "设备句柄入"=w3029) -> ("错误输出"=w3024:errorcluster, "设备句柄"=w3025:i32)  [unwired: 7 in]
            n1615 = call "编码器清零.vi"("错误输入"=w3024, "通道号"=2, "设备句柄入"=w3025) -> ("错误输出"=w3023:errorcluster)  [unwired: 7 in, 1 out]
          }
          event "DA输出范围": Value Change {
            n1616 = event-data() -> ()  [unwired: 1 in, 5 out]
            n1617 = local read "DA输出范围"() -> (w3033:i32)
            n1618 = case shown="4" w3033 {
              tunnel: [10000.0 ("标尺.范围:最大值") 5000.0 ("标尺.范围:最大值") 10000.0 ("标尺.范围:最大值") 5000.0 ("标尺.范围:最大值") 20000.0 ("标尺.范围:最大值")] -> w3031
              tunnel: [-10000.0 ("标尺.范围:最大值") -5000.0 ("标尺.范围:最大值") 0.0 ("标尺.范围:最大值") 0.0 ("标尺.范围:最大值") 0.0 ("标尺.范围:最大值")] -> w3030
              frame 0, Default {
              }
              frame 1 {
              }
              frame 2 {
              }
              frame 3 {
              }
              frame 4 {
              }
            }
            n1619 = property on="CH1" class="Slide (严格)"("Scale.Maximum"=w3031, "Scale.Minimum"=w3030) -> ()  [unwired: 2 in, 2 out]
            n1620 = property on="CH2" class="Slide (严格)"("Scale.Maximum"=w3031, "Scale.Minimum"=w3030) -> ()  [unwired: 2 in, 2 out]
            n1621 = property on="CH3" class="Slide (严格)"("Scale.Maximum"=w3031, "Scale.Minimum"=w3030) -> ()  [unwired: 2 in, 2 out]
            n1622 = property on="CH4" class="Slide (严格)"("Scale.Maximum"=w3031, "Scale.Minimum"=w3030) -> ()  [unwired: 2 in, 2 out]
          }
          event "M系列PWM停止": Value Change {
            n1623 = event-data() -> ()  [unwired: 1 in, 5 out]
            n1624 = call "使能或禁止PWM输出(只支持EM9636M).vi"("错误输入"=w3046, "相位设置数组"=i8[] [0, 0, 0] ("PWM使能"), "PWM使能"=i8[] [0, 0, 0], "设备句柄入"=w3047) -> ("错误输出"=w3045:errorcluster)  [unwired: 6 in, 1 out]
          }
          event "PWM停止": Value Change {
            n1625 = event-data() -> ()  [unwired: 1 in, 5 out]
            n1626 = call "使能或禁止PWM输出.vi"("错误输入"=w3051, "所用PWM使能"=i8 0, "设备句柄入"=w3052) -> ("错误输出"=w3049:errorcluster)  [unwired: 7 in, 1 out]
          }
        }
        "错误输出 2" <- w2805
        n1627 = local read "停止"() -> (w2808:bool)
      }
      n1628 = while {
        stop <- "停止" stop-if-true
        n1629 = local read "布尔"() -> (w3055:bool)
        n1630 = Wait (ms)(milliseconds to wait=u32 10 ("等待时间（毫秒）")) -> ()  [unwired: 1 out]
        n1631 = case shown="真" w3055 {
          frame False {
          }
          frame True {
            n1632 = local read "设备句柄"() -> (w3066:i32)
            n1633 = local read "每次总数据量"() -> (w3064:i32)
            n1634 = call "得到上位机软件缓冲区数据个数(M).vi"("设备句柄入"=w3066) -> ("错误输出"=w3062:errorcluster, "可读数据个数"=w3065:i32, "设备句柄"=w3063:i32)  [unwired: 8 in]
            n1635 = call <vilib>:"Clear Errors.vi"("error in (no error)"=w3062) -> ()  [unwired: 5 in, 2 out]
            n1636 = Not(x=w3062) -> (.not. x?=→"采集卡左":bool)
            n1637 = Greater Or Equal?(x=w3065, y=w3064) -> (x >= y?=w3061:bool)
            n1638 = case shown="真" w3061 {
              tunnel: w3064 -> [_ w3078]
              tunnel: w3063 -> [_ w3077]
              frame False {
              }
              frame True {
                n1639 = call "读取高速数据(M).vi"("数据个数"=w3078, "设备句柄入"=w3077) -> ("错误输出"=w3084:errorcluster, "返回数据个数"=w3085:i32, "原码值"=w3086:u16[], "设备句柄"=w3087:i32)  [unwired: 6 in]
                "错误输出" <- w3084
                n1640 = local read "每次总数据量"() -> (w3082:i32)
                n1641 = local read "通道数量"() -> (w3071:i32)
                n1642 = Divide(x=w3082, y=w3071) -> (x/y=w3081:dbl)
                n1643 = call "AD原码转物理.vi"("设备句柄入"=w3087, "原码值"=w3086, "个数"=w3085, "错误输入"=w3084) -> ("物理值"=w3083:dbl[])  [unwired: 4 in, 2 out]
                n1644 = To Long Integer(number=w3081) -> (32bit integer=w3080:i32)
                n1645 = Reshape Array "重排数组维数"(w3083, w3080, w3071) -> (w3079:dbl[][])
                n1646 = Transpose 2D Array(2D array=w3079) -> (transposed array=w3075:dbl[][])
                n1647 = Array Size(array=w3075) -> (size(s)=w3074:i32[])
                n1648 = for {
                  tunnel: w3075 -> [w3089] mode=indexing
                  tunnel: [w3088] -> w3076 mode=indexing
                  n1649 = Add Array Elements(numeric array=w3089) -> (sum=w3088:dbl)
                }
                n1650 = Index Array(array=w3074, index=1 ("索引")) -> (element=w3072:i32)
                n1651 = Divide(x=w3076, y=w3072) -> (x/y=w3070:dbl[])
                "AD均值数据" <- w3070
                n1652 = Reshape Array(w3070, 4 ("维数大小"), 8 ("维数大小")) -> (→"输出数组左":dbl[][])
              }
            }
          }
        }
        n1653 = local read "设备句柄"() -> (w3053:i32)
        n1654 = case shown="真" "停止" {
          tunnel: w3053 -> [_ w3057]
          frame False {
          }
          frame True {
            n1655 = flat-sequence {
              tunnel: w3057 -> [w3058]
              frame #0 {
                n1656 = call "停止采集(M).vi"("设备句柄入"=w3058) -> ()  [unwired: 9 in, 2 out]
              }
              frame #1 {
                "布尔" <- FALSE ("布尔")
              }
            }
          }
        }
      }
    }
    frame #2 {
      n1657 = flat-sequence {
        tunnel: [w3100] -> w3096
        tunnel: [w3098] -> w3095
        tunnel: w3096 -> [w3106]
        tunnel: [w3105] -> w3094
        tunnel: w3095 -> [w3104]
        tunnel: [w3103] -> w3093
        tunnel: w3094 -> [w3112]
        tunnel: [w3111] -> w3092
        tunnel: w3093 -> [w3110]
        tunnel: [w3109] -> w3091
        tunnel: w3092 -> [w3117]
        tunnel: [w3116] -> w3090
        tunnel: w3091 -> [w3115]
        tunnel: w3090 -> [w3118]
        frame #0 {
          n1658 = local read "设备句柄"() -> (w3101:i32)
          n1659 = local read "错误输出"() -> (w3099:errorcluster)
          n1660 = call "停止采集(M).vi"("错误输入"=w3099, "设备句柄入"=w3101) -> ("错误输出"=w3098:errorcluster, "设备句柄"=w3100:i32)  [unwired: 8 in]
          n1661 = Wait (ms)(milliseconds to wait=u32 10 ("等待时间（毫秒）")) -> ()  [unwired: 1 out]
        }
        frame #1 {
          n1662 = call "使能或禁止PWM输出.vi"("错误输入"=w3104, "所用PWM使能"=i8 0, "设备句柄入"=w3106) -> ("错误输出"=w3103:errorcluster, "设备句柄"=w3105:i32)  [unwired: 7 in]
          n1663 = Wait (ms)(milliseconds to wait=u32 10 ("等待时间（毫秒）")) -> ()  [unwired: 1 out]
        }
        frame #2 {
          n1664 = call "关闭数据连接.vi"("错误输入"=w3110, "设备句柄入"=w3112) -> ("错误输出"=w3109:errorcluster, "设备句柄"=w3111:i32)  [unwired: 8 in]
          n1665 = Wait (ms)(milliseconds to wait=u32 10 ("等待时间（毫秒）")) -> ()  [unwired: 1 out]
        }
        frame #3 {
          n1666 = call "关闭命令连接.vi"("错误输入"=w3115, "设备句柄入"=w3117) -> ("错误输出"=w3114:errorcluster, "设备句柄"=w3116:i32)  [unwired: 8 in]
          n1667 = Wait (ms)(milliseconds to wait=u32 10 ("等待时间（毫秒）")) -> ()  [unwired: 1 out]
          n1668 = local write "错误输出"(w3114) -> ()
        }
        frame #4 {
          n1669 = call "关闭设备.vi"("设备句柄"=w3118) -> ()  [unwired: 10 in]
        }
        frame #5 {
          "close" <- TRUE ("close")
        }
      }
    }
  }
  n1670 = while {
    stop <- w3210 stop-if-true
    # "原本以为返回的是百分比，要\n重新标定"
    # "4"
    # "3"
    # "2"
    # "1"
    # "档位"
    # "功率"
    # "扭矩"
    # "车速"
    n1671 = local read "加载功率"() -> (w3165:dbl)
    n1672 = call "asc转换.vi"("输入数据"=w3165) -> ("数值位 5"=w3176:u8, "数值位 4"=w3177:u8, "数值位 3"=w3178:u8, "数值位 2"=w3179:u8)  [unwired: 7 in]
    n1673 = local write "0byte 5"(u8 80 ("6byte 3")) -> ()
    n1674 = local write "1byte 5"(u8 6 ("7byte 3")) -> ()
    n1675 = local write "2byte 5"(u8 32 ("7byte 3")) -> ()
    n1676 = local write "3byte 5"(w3179) -> ()
    n1677 = local write "4byte 5"(w3178) -> ()
    n1678 = local write "5byte 5"(w3177) -> ()
    n1679 = local write "6byte 5"(w3176) -> ()
    n1680 = local write "7byte 5"(u8 32 ("7byte 3")) -> ()
    n1681 = local write "0byte"(u8 16 ("6byte 3")) -> ()
    n1682 = local write "1byte"(u8 6 ("7byte 3")) -> ()
    n1683 = local write "2byte"("左1字符") -> ()
    n1684 = local write "3byte"("左2字符") -> ()
    n1685 = local write "4byte"("左3字符") -> ()
    n1686 = local write "5byte"("左4字符") -> ()
    n1687 = local write "6byte"("左5字符") -> ()
    n1688 = local write "7byte"(u8 32 ("7byte 3")) -> ()
    n1689 = local read "加载左上转速监控"() -> (w3166:dbl)
    n1690 = local read "加载左上转矩监控"() -> (w3191:i16)
    n1691 = Greater Or Equal?(x=w3166, y=0.0) -> (x >= y?=w3202:bool)
    n1692 = Absolute Value(x=w3166) -> (abs(x)=w3195:dbl)
    n1693 = Greater Or Equal?(x=w3191, y=0.0) -> (x >= y?=w3194:bool)
    n1694 = Absolute Value(x=w3191) -> (abs(x)=w3180:i16)
    n1695 = case shown="真" w3202 {
      tunnel: w3195 -> [w3275 w3277]
      tunnel: [w3275 w3277] -> w3197
      tunnel: [u8 45 ("6byte 3") u8 32 ("6byte 3")] -> w3196
      frame False {
      }
      frame True {
      }
    }
    n1696 = case shown="假" w3194 {
      tunnel: w3180 -> [w3271 w3273]
      tunnel: [w3271 w3273] -> w3192
      tunnel: [u8 45 ("6byte 3") u8 32 ("6byte 3")] -> w3186
      frame False {
      }
      frame True {
      }
    }
    n1697 = call <vilib>:"Boolean Crossing PtByPt.vi"("direction"=enum16{"either", "false-true", "true-false"}."false-true", "input"="加载电机复位") -> ("crossing"=w3140:bool)  [unwired: 1 in]
    n1698 = call "asc转换.vi"("输入数据"=w3197) -> ("数值位 5"=w3198:u8, "数值位 4"=w3199:u8, "数值位 3"=w3200:u8, "数值位 2"=w3201:u8)  [unwired: 7 in]
    n1699 = case shown="真" w3140 {
      frame False {
      }
      frame True {
        w3212 = TRUE
        n1700 = local write "变频6"(w3212) -> ()
        n1701 = local write "变频5"(w3212) -> ()
        n1702 = local write "变频4"(w3212) -> ()
        n1703 = local write "变频3"(w3212) -> ()
        n1704 = local write "变频2"(w3212) -> ()
        n1705 = local write "变频1"(w3212) -> ()
      }
    }
    n1706 = call "asc转换.vi"("输入数据"=w3192) -> ("数值位 5"=w3187:u8, "数值位 4"=w3188:u8, "数值位 3"=w3189:u8, "数值位 2"=w3190:u8)  [unwired: 7 in]
    n1707 = local write "0byte 3"(u8 48 ("6byte 3")) -> ()
    n1708 = local write "1byte 3"(u8 6 ("7byte 3")) -> ()
    n1709 = local write "2byte 3"(w3196) -> ()
    n1710 = local write "3byte 3"(w3201) -> ()
    n1711 = local write "4byte 3"(w3200) -> ()
    n1712 = local write "5byte 3"(w3199) -> ()
    n1713 = local write "6byte 3"(w3198) -> ()
    n1714 = local write "7byte 3"(u8 82 ("7byte 3")) -> ()
    n1715 = local write "0byte 7"(u8 112 ("6byte 3")) -> ()
    n1716 = local write "1byte 7"(u8 6 ("7byte 3")) -> ()
    n1717 = local write "2byte 7"(w3186) -> ()
    n1718 = local write "3byte 7"(w3190) -> ()
    n1719 = local write "4byte 7"(w3189) -> ()
    n1720 = local write "5byte 7"(w3188) -> ()
    n1721 = local write "6byte 7"(w3187) -> ()
    n1722 = local write "7byte 7"(u8 32 ("7byte 3")) -> ()
    n1723 = local read "加载右上转速监控"() -> (w3123:dbl)
    n1724 = local read "加载左上转速监控"() -> (w3122:dbl)
    n1725 = local read "加载转速右下监控"() -> (w3121:dbl)
    n1726 = local read "加载左下转速监控"() -> (w3120:dbl)
    n1727 = local read "加载转矩右上监控"() -> (w3153:i16)
    n1728 = local read "加载右下转矩监控"() -> (w3148:i16)
    n1729 = local read "加载左下转矩监控"() -> (w3147:i16)
    n1730 = local read "加载左上转矩监控"() -> (w3149:i16)
    n1731 = local read "加载左上转速监控"() -> (w3175:dbl)
    n1732 = Multiply(x=w3153, y=0.1) -> (x*y=w3139:dbl)
    n1733 = Multiply(x=w3149, y=0.1) -> (x*y=w3138:dbl)
    n1734 = Multiply(x=w3147, y=0.1) -> (x*y=w3136:dbl)
    n1735 = Multiply(x=w3148, y=0.1) -> (x*y=w3137:dbl)
    n1736 = Compound Arithmetic op=MULTIPLY(w3175, 0.52 ("值"), 3.141592653589793, 60.0 ("值")) -> (w3171:dbl)
    n1737 = Multiply(x=w3139, y=w3123) -> (x*y=w3132:dbl)
    n1738 = Multiply(x=w3138, y=w3122) -> (x*y=w3131:dbl)
    n1739 = Multiply(x=w3137, y=w3121) -> (x*y=w3130:dbl)
    n1740 = Multiply(x=w3136, y=w3120) -> (x*y=w3129:dbl)
    n1741 = local read "元素 4"() -> (w3155:bool)
    n1742 = Divide(x=w3171, y=1000.0) -> (x/y=w3145:dbl)
    n1743 = local read "布尔数组"() -> (w3168:bool[])
    n1744 = local write "遥控器按钮确认"(w3155) -> ()
    n1745 = Multiply(x=w3145, y=-1.0) -> (x*y=→"车速":dbl)
    n1746 = Divide(x=w3129, y=9550.0) -> (x/y=w3125:dbl)
    n1747 = Divide(x=w3132, y=9550.0) -> (x/y=w3128:dbl)
    n1748 = Divide(x=w3131, y=9550.0) -> (x/y=w3127:dbl)
    n1749 = Divide(x=w3130, y=9550.0) -> (x/y=w3126:dbl)
    n1750 = Index Array(array=w3168) -> (element #1=→"元素 3":bool, element #2=→"元素 4":bool, element #5=w3167:bool)  [unwired: 8 in, 5 out]
    n1751 = Compound Arithmetic op=ADD(w3128, w3127, w3126, w3125) -> (w3124:dbl)
    n1752 = Absolute Value(x=w3124) -> (abs(x)=→"加载功率":dbl)
    n1753 = case shown="假" w3167 {
      frame False {
        w3226 = u8 32 ("左1字符")
        n1754 = local read "布尔数组 2"() -> (w3239:bool[])
        n1755 = local read "布尔数组"() -> (w3240:bool[])
        n1756 = local write "左3字符"(w3226) -> ()
        n1757 = local write "左4字符"(w3226) -> ()
        n1758 = local write "左5字符"(w3226) -> ()
        n1759 = Index Array(array=w3239) -> (element #1=w3231:bool, element #2=w3230:bool, element #3=w3229:bool, element #4=w3228:bool)  [unwired: 8 in, 4 out]
        n1760 = Index Array(array=w3240) -> (element #2=→"元素":bool, element #3=→"元素 2":bool, element #4=w3238:bool, element #6=w3227:bool, element #7=w3237:bool, element #8=w3236:bool)  [unwired: 8 in, 2 out]
        n1761 = And(x=w3227, y=w3231) -> (x .and. y?=w3218:bool)
        n1762 = And(x=w3227, y=w3236) -> (x .and. y?=w3217:bool)
        n1763 = And(x=w3227, y=w3237) -> (x .and. y?=w3216:bool)
        n1764 = Compound Arithmetic op=OR ("复合运算")(w3216, w3217, w3218) -> (w3215:bool)
        n1765 = case shown="真" w3215 {
          frame False {
          }
          frame True {
            n1766 = local write "左1字符"(u8 82 ("左1字符")) -> ()
          }
        }
        n1767 = And(x=w3227, y=w3230) -> (x .and. y?=w3234:bool)
        n1768 = And(x=w3227, y=w3229) -> (x .and. y?=w3233:bool)
        n1769 = And(x=w3227, y=w3228) -> (x .and. y?=w3232:bool)
        n1770 = And(x=w3238, y=w3237) -> (x .and. y?=w3225:bool)
        n1771 = And(x=w3238, y=w3236) -> (x .and. y?=w3224:bool)
        n1772 = And(x=w3238, y=w3231) -> (x .and. y?=w3223:bool)
        n1773 = And(x=w3238, y=w3230) -> (x .and. y?=w3222:bool)
        n1774 = And(x=w3238, y=w3229) -> (x .and. y?=w3221:bool)
        n1775 = And(x=w3238, y=w3228) -> (x .and. y?=w3220:bool)
        n1776 = Compound Arithmetic op=OR ("复合运算")(w3225, w3224, w3223, w3222, w3221, w3220) -> (w3219:bool)
        n1777 = case shown="假" w3219 {
          frame False {
          }
          frame True {
            n1778 = local write "左1字符"(u8 68 ("左1字符")) -> ()
          }
        }
        n1779 = Compound Arithmetic op=OR ("复合运算")(w3234, w3233, w3232) -> (w3235:bool)
        n1780 = case shown="真" w3235 {
          frame False {
          }
          frame True {
            n1781 = local write "左1字符"(u8 69 ("左1字符")) -> ()
            n1782 = local write "左2字符"(u8 82 ("左1字符")) -> ()
            n1783 = local write "左3字符"(u8 82 ("左1字符")) -> ()
            n1784 = local write "左4字符"(u8 79 ("左1字符")) -> ()
            n1785 = local write "左5字符"(u8 82 ("左1字符")) -> ()
            n1786 = local write "当前试验档位"("无效档" ("当前试验档位")) -> ()
          }
        }
        n1787 = case shown="真" w3218 {
          frame False {
          }
          frame True {
            n1788 = local write "当前试验档位"("R3" ("当前试验档位")) -> ()
            n1789 = local write "左2字符"(u8 51 ("左1字符")) -> ()
          }
        }
        n1790 = case shown="真" w3217 {
          frame False {
          }
          frame True {
            n1791 = local write "当前试验档位"("R2" ("当前试验档位")) -> ()
            n1792 = local write "左2字符"(u8 50 ("左1字符")) -> ()
          }
        }
        n1793 = case shown="真" w3221 {
          frame False {
          }
          frame True {
            n1794 = local write "当前试验档位"("D5" ("当前试验档位")) -> ()
            n1795 = local write "左2字符"(u8 53 ("左1字符")) -> ()
          }
        }
        n1796 = case shown="真" w3222 {
          frame False {
          }
          frame True {
            n1797 = local write "当前试验档位"("D4" ("当前试验档位")) -> ()
            n1798 = local write "左2字符"(u8 52 ("左1字符")) -> ()
          }
        }
        n1799 = case shown="真" w3216 {
          frame False {
          }
          frame True {
            n1800 = local write "当前试验档位"("R1" ("当前试验档位")) -> ()
            n1801 = local write "左2字符"(u8 49 ("左1字符")) -> ()
          }
        }
        n1802 = case shown="真" w3225 {
          frame False {
          }
          frame True {
            n1803 = local write "当前试验档位"("D1" ("当前试验档位")) -> ()
            n1804 = local write "左2字符"(u8 49 ("左1字符")) -> ()
          }
        }
        n1805 = case shown="真" w3223 {
          frame False {
          }
          frame True {
            n1806 = local write "当前试验档位"("D3" ("当前试验档位")) -> ()
            n1807 = local write "左2字符"(u8 51 ("左1字符")) -> ()
          }
        }
        n1808 = case shown="真" w3220 {
          frame False {
          }
          frame True {
            n1809 = local write "当前试验档位"("D6" ("当前试验档位")) -> ()
            n1810 = local write "左2字符"(u8 54 ("左1字符")) -> ()
          }
        }
        n1811 = case shown="真" w3224 {
          frame False {
          }
          frame True {
            n1812 = local write "当前试验档位"("D2" ("当前试验档位")) -> ()
            n1813 = local write "左2字符"(u8 50 ("左1字符")) -> ()
          }
        }
      }
      frame True {
        w3267 = u8 32 ("左1字符")
        n1814 = local write "当前试验档位"("N" ("当前试验档位")) -> ()
        n1815 = local write "左2字符"(w3267) -> ()
        n1816 = local write "左3字符"(w3267) -> ()
        n1817 = local write "左4字符"(w3267) -> ()
        n1818 = local write "左5字符"(w3267) -> ()
        n1819 = local write "左1字符"(u8 78 ("左1字符")) -> ()
      }
    }
    n1820 = local read "停止"() -> (w3210:bool)
    n1821 = Wait (ms)(milliseconds to wait=u32 50 ("等待时间（毫秒）")) -> ()  [unwired: 1 out]
  }
  n1822 = stacked-sequence {
    frame #0 {
      n1823 = stacked-sequence {
        frame #0 {
          w3281 = FALSE ("AD开始采集")
          n1824 = local write "AD开始采集 2"(w3281) -> ()
          n1825 = local write "PWM输出 2"(w3281) -> ()
          n1826 = local write "布尔 2"(FALSE ("布尔")) -> ()
          n1827 = local write "采集卡右"(FALSE ("采集卡右")) -> ()
          n1828 = local write "停止"(FALSE ("停止")) -> ()
          n1829 = local write "close2"(FALSE ("close2")) -> ()
        }
        frame #1 {
          n1830 = flat-sequence {
            tunnel: [w3293] -> w3290
            tunnel: [w3292] -> w3289
            tunnel: w3290 -> [w3298]
            tunnel: w3289 -> [w3297]
            tunnel: [w3296] -> w3288
            tunnel: [w3295] -> w3287
            tunnel: w3288 -> [w3305]
            tunnel: w3287 -> [w3304]
            tunnel: [w3303] -> w3286
            tunnel: [w3302] -> w3285
            tunnel: w3286 -> [w3311]
            tunnel: w3285 -> [w3310]
            tunnel: [w3309] -> w3284
            tunnel: [w3308] -> w3283
            tunnel: w3284 -> [w3315]
            tunnel: w3283 -> [w3314]
            frame #0 {
              n1831 = call "建立设备.vi"() -> ("错误输出"=w3292:errorcluster, "设备句柄"=w3293:i32)  [unwired: 10 in]
              n1832 = Wait (ms)(milliseconds to wait=u32 10 ("等待时间（毫秒）")) -> ()  [unwired: 1 out]
            }
            frame #1 {
              n1833 = Wait (ms)(milliseconds to wait=u32 10 ("等待时间（毫秒）")) -> ()  [unwired: 1 out]
              n1834 = call "建立命令连接.vi"("IP地址"="192.168.1.126" ("IP地址 2"), "错误输入"=w3297, "端口号"=8000 ("命令端口 2"), "设备句柄入"=w3298) -> ("错误输出"=w3295:errorcluster, "设备句柄"=w3296:i32)  [unwired: 6 in]
            }
            frame #2 {
              n1835 = Wait (ms)(milliseconds to wait=u32 10 ("等待时间（毫秒）")) -> ()  [unwired: 1 out]
              n1836 = call "建立数据连接.vi"("错误输入"=w3304, "端口号"=8001 ("数据端口 2"), "设备句柄入"=w3305) -> ("错误输出"=w3302:errorcluster, "设备句柄"=w3303:i32)  [unwired: 7 in]
            }
            frame #3 {
              n1837 = local write "设置开关量方向 2"(cluster{"IO1~IO8":i8, "IO9~IO16":i8} {"IO1~IO8"=1, "IO9~IO16"=1} ("设置开关量方向")) -> ()
              n1838 = call "设置开关量方向.vi"("错误输入"=w3310, "方向"=i8[] [1, 1, 1, 1], "设备句柄入"=w3311) -> ("错误输出"=w3308:errorcluster, "设备句柄"=w3309:i32)  [unwired: 7 in]
              n1839 = Wait (ms)(milliseconds to wait=u32 10 ("等待时间（毫秒）")) -> ()  [unwired: 1 out]
            }
            frame #4 {
              n1840 = local write "错误输出 6"(w3314) -> ()
              "设备句柄 2" <- w3315
            }
          }
        }
        frame #2 {
        }
      }
    }
    frame #1 {
      n1841 = local read "错误输出 6"() -> (w3316:errorcluster)
      n1842 = while {
        stop <- w3567 stop-if-true
        n1843 = local read "布尔 2"() -> (w3568:bool)
        n1844 = Wait (ms)(milliseconds to wait=u32 10 ("等待时间（毫秒）")) -> ()  [unwired: 1 out]
        n1845 = case shown="真" w3568 {
          frame False {
          }
          frame True {
            n1846 = local read "设备句柄 2"() -> (w3579:i32)
            n1847 = local read "每次总数据量 2"() -> (w3577:i32)
            n1848 = call "得到上位机软件缓冲区数据个数(M).vi"("设备句柄入"=w3579) -> ("错误输出"=w3575:errorcluster, "可读数据个数"=w3578:i32, "设备句柄"=w3576:i32)  [unwired: 8 in]
            n1849 = call <vilib>:"Clear Errors.vi"("error in (no error)"=w3575) -> ()  [unwired: 5 in, 2 out]
            n1850 = Not(x=w3575) -> (.not. x?=→"采集卡右":bool)
            n1851 = Greater Or Equal?(x=w3578, y=w3577) -> (x >= y?=w3574:bool)
            n1852 = case shown="真" w3574 {
              tunnel: w3577 -> [_ w3591]
              tunnel: w3576 -> [_ w3590]
              frame False {
              }
              frame True {
                n1853 = local read "每次总数据量 2"() -> (w3595:i32)
                n1854 = local read "通道数量 2"() -> (w3584:i32)
                n1855 = call "读取高速数据(M).vi"("数据个数"=w3591, "设备句柄入"=w3590) -> ("错误输出"=w3597:errorcluster, "返回数据个数"=w3598:i32, "原码值"=w3599:u16[], "设备句柄"=w3600:i32)  [unwired: 6 in]
                "错误输出 6" <- w3597
                n1856 = Divide(x=w3595, y=w3584) -> (x/y=w3594:dbl)
                n1857 = call "AD原码转物理.vi"("设备句柄入"=w3600, "原码值"=w3599, "个数"=w3598, "错误输入"=w3597) -> ("物理值"=w3596:dbl[])  [unwired: 4 in, 2 out]
                n1858 = To Long Integer(number=w3594) -> (32bit integer=w3593:i32)
                n1859 = Reshape Array "重排数组维数"(w3596, w3593, w3584) -> (w3592:dbl[][])
                n1860 = Transpose 2D Array(2D array=w3592) -> (transposed array=w3588:dbl[][])
                n1861 = Array Size(array=w3588) -> (size(s)=w3587:i32[])
                n1862 = for {
                  tunnel: w3588 -> [w3602] mode=indexing
                  tunnel: [w3601] -> w3589 mode=indexing
                  n1863 = Add Array Elements(numeric array=w3602) -> (sum=w3601:dbl)
                }
                n1864 = Index Array(array=w3587, index=1 ("索引")) -> (element=w3585:i32)
                n1865 = Divide(x=w3589, y=w3585) -> (x/y=w3583:dbl[])
                "AD均值数据 2" <- w3583
                n1866 = Reshape Array(w3583, 4 ("维数大小"), 8 ("维数大小")) -> (→"输出数组右":dbl[][])
              }
            }
          }
        }
        n1867 = local read "设备句柄 2"() -> (w3566:i32)
        n1868 = local read "停止"() -> (w3567:bool)
        n1869 = case shown="真" w3567 {
          tunnel: w3566 -> [_ w3570]
          frame False {
          }
          frame True {
            n1870 = flat-sequence {
              tunnel: w3570 -> [w3571]
              frame #0 {
                n1871 = call "停止采集(M).vi"("设备句柄入"=w3571) -> ()  [unwired: 9 in, 2 out]
              }
              frame #1 {
                "布尔 2" <- FALSE ("布尔")
              }
            }
          }
        }
      }
      n1872 = while {
        shift-right: [w3318] -> _
        shift-left: w3316 -> [w3319]
        stop <- w3321 stop-if-true
        n1873 = local read "设备句柄 2"() -> (w3317:i32)
        n1874 = event shown="[1] 菜单选择(用户)" {
          selector: _ -> [_ _ _ _ _ _ _ _ _ _ _ _ _ _]
          dyn-events: _ -> [_ _ _ _ _ _ _ _ _ _ _ _ _ _]
          timeout: 100 -> [_ _ _ _ _ _ _ _ _ _ _ _ _ _]
          tunnel: w3317 -> [w3341 w3373 w3415 w3420 w3436 w3469 w3491 w3496 w3506 w3527 w3542 _ w3560 w3565]
          tunnel: w3319 -> [w3340 w3372 w3417 w3419 w3435 w3468 w3490 w3495 w3505 w3526 w3541 w3545 w3559 w3564]
          tunnel: [w3325 w3371 w3416 w3418 w3434 w3444 w3483 w3494 w3504 w3508 w3536 w3545 w3558 w3562] -> w3318
          event Timeout {
            n1875 = event-data() -> ()  [unwired: 1 in, 2 out]
            n1876 = call "得到所有通道开关量值.vi"("错误输入"=w3340, "设备句柄入"=w3341) -> ("错误输出"=w3323:errorcluster, "iStatus"=w3332:i8[], "设备句柄"=w3337:i32)  [unwired: 7 in]
            "错误输出 5" <- w3323
            n1877 = Array Subset(array=w3332, index=0 ("索引"), length=16 ("长度")) -> (w3329:i8[])
            n1878 = for {
              tunnel: w3329 -> [w3361] mode=indexing
              tunnel: [w3358] -> w3328 mode=indexing
              n1879 = Equal?(x=w3361, y=i8 1) -> (x = y?=w3359:bool)
              n1880 = case shown="假" w3359 {
                tunnel: [FALSE TRUE] -> w3358
                frame False {
                }
                frame True {
                }
              }
            }
            n1881 = Array Subset(array=w3332, index=16 ("索引"), length=8 ("长度")) -> (w3331:i8[])
            n1882 = for {
              tunnel: [w3365] -> w3330 mode=indexing
              tunnel: w3331 -> [w3364] mode=indexing
              n1883 = Equal?(x=w3364, y=i8 1) -> (x = y?=w3366:bool)
              n1884 = case shown="假" w3366 {
                tunnel: [FALSE TRUE] -> w3365
                frame False {
                }
                frame True {
                }
              }
            }
            "光隔离输入 2" <- w3330
            n1885 = Array To Cluster(array=w3328) -> (cluster=→"可编程数字量I/O(映射控件)--得到所有通道开关量值 2":T22)
            n1886 = call "读取编码器.vi"("错误输入"=w3323, "设备句柄入"=w3337) -> ("错误输出"=w3327:errorcluster, "编码器过零值"=→"编码器过零值 2":i16[], "编码器AB值"=→"编码器AB值 2":i32[], "设备句柄"=w3326:i32)  [unwired: 6 in]
            n1887 = local read "开启计数 2"() -> (w3324:bool)
            n1888 = case shown="真" w3324 {
              tunnel: w3327 -> [w3342 w3350]
              tunnel: w3326 -> [_ w3349]
              tunnel: [w3342 w3348] -> w3325
              frame False {
              }
              frame True {
                n1889 = call "读取所有路计数器的原码值.vi"("错误输入"=w3350, "设备句柄入"=w3349) -> ("错误输出"=w3346:errorcluster, "计数器的原码值"=w3343:u32[], "设备句柄"=w3347:i32)  [unwired: 7 in]
                n1890 = for {
                  N: 6 -> [_]
                  tunnel: w3347 -> [w3357]
                  tunnel: w3346 -> [w3356]
                  tunnel: [w3355] -> w3348
                  tunnel: [w3352] -> w3344 mode=indexing
                  tunnel: w3343 -> [w3351] mode=indexing
                  i -> [w3354]
                  n1891 = Increment(x=w3354) -> (x+1=w3353:i32)
                  n1892 = call "计数器值转换成对应的物理值.vi"("错误输入"=w3356, "ctCode"=w3351, "chNo"=w3353, "设备句柄入"=w3357) -> ("错误输出"=w3355:errorcluster, "ctValue"=w3352:dbl)  [unwired: 5 in, 1 out]
                }
                "计数/测频（Hz）值 2" <- w3344
              }
            }
          }
          event Menu Selection (User) {
            n1893 = event-data() -> ("ItemTag"=w3370:string)  [unwired: 1 in, 6 out]
            n1894 = case shown="\"采集卡右\"" w3370 {
              tunnel: w3373 -> [_ w3376]
              tunnel: w3372 -> [_ w3375]
              tunnel: [_ w3374] -> w3371
              frame "假", Default {
              }
              frame "采集卡右" {
                n1895 = flat-sequence {
                  tunnel: w3376 -> [w3380]
                  tunnel: w3375 -> [w3379]
                  tunnel: [w3378] -> w3377
                  tunnel: [w3414] -> w3374
                  tunnel: w3377 -> [w3414]
                  frame #0 {
                    n1896 = call "AD设置范围.vi"("错误输入"=w3379, "范围"="AD范围 2", "设备句柄入"=w3380) -> ("错误输出"=w3401:errorcluster, "设备句柄"=w3400:i32)  [unwired: 7 in]
                    n1897 = call "AD设置单双端.vi"("错误输入"=w3401, "单双端"="单双端 2", "设备句柄入"=w3400) -> ("错误输出"=w3403:errorcluster, "设备句柄"=w3402:i32)  [unwired: 7 in]
                    n1898 = call "AD设置增益.vi"("错误输入"=w3403, "增益"="增益 2", "设备句柄入"=w3402) -> ("错误输出"=w3410:errorcluster, "设备句柄"=w3409:i32)  [unwired: 7 in]
                    n1899 = call "AD设置通道范围.vi"("错误输入"=w3410, "起始通道"="AD起始通道 2", "终止通道"="AD终止通道 2", "设备句柄入"=w3409) -> ("错误输出"=w3404:errorcluster, "设备句柄"=w3405:i32)  [unwired: 6 in]
                    n1900 = Subtract(x="AD终止通道 2", y="AD起始通道 2") -> (x-y=w3388:i32)
                    n1901 = Increment(x=w3388) -> (x+1=w3406:i32)
                    "通道数量 2" <- w3406
                    n1902 = call "设定通道频率.vi"("错误输入"=w3404, "通道频率"="通道频率Hz 2", "设备句柄入"=w3405) -> ("错误输出"=w3392:errorcluster, "设备句柄"=w3391:i32)  [unwired: 7 in]
                    n1903 = local read "伪同步 2"() -> (w3397:i32)
                    n1904 = case shown="0, 默认" w3397 {
                      tunnel: "通道频率Hz 2" -> [w3411 _]
                      tunnel: [w3411 w3412] -> w3383
                      tunnel: "组频率Hz 2" -> [_ w3412]
                      frame 0, Default {
                      }
                      frame 1 {
                      }
                    }
                    n1905 = call "设定组频率.vi"("错误输入"=w3392, "组频率"="组频率Hz 2", "设备句柄入"=w3391) -> ("错误输出"=w3408:errorcluster, "设备句柄"=w3407:i32)  [unwired: 7 in]
                    n1906 = Divide(x=w3383, y=2.0 ("每秒刷新数据次数")) -> (x/y=w3381:dbl)
                    n1907 = To Long Integer(number=w3381) -> (32bit integer=w3386:i32)
                    n1908 = Quotient & Remainder(x=w3386, y=w3406) -> (floor(x/y)=w3385:i32)  [unwired: 1 out]
                    "每通道数据量 2" <- w3385
                    n1909 = Multiply(x=w3385, y=w3406) -> (x*y=→"每次总数据量 2":i32)
                    n1910 = call "启动采集(M系列).vi"("错误输入"=w3408, "时钟源"="时钟源 2", "伪同步"="伪同步 2", "设备句柄入"=w3407) -> ("错误输出"=w3378:errorcluster)  [unwired: 6 in, 1 out]
                  }
                  frame #1 {
                    n1911 = local write "布尔 2"(TRUE ("布尔")) -> ()
                  }
                }
              }
            }
          }
          event "AD停止采集 2": Value Change {
            n1912 = event-data() -> ()  [unwired: 1 in, 5 out]
            n1913 = call "停止采集(M).vi"("错误输入"=w3417, "设备句柄入"=w3415) -> ("错误输出"=w3416:errorcluster)  [unwired: 8 in, 1 out]
          }
          event "开启计数 2": Value Change {
            n1914 = event-data() -> ()  [unwired: 1 in, 5 out]
            n1915 = Initialize Array("工作方式 2", 6 ("维数大小")) -> (w3424:u16[])
            n1916 = call "设置所有路计数器的工作方式.vi"("错误输入"=w3419, "ctMode"=w3424, "设备句柄入"=w3420) -> ("错误输出"=w3423:errorcluster, "设备句柄"=w3422:i32)  [unwired: 7 in]
            n1917 = for {
              N: 6 -> [_]
              tunnel: w3423 -> [w3432]
              tunnel: w3422 -> [w3431]
              tunnel: [w3427] -> w3418
              i -> [w3429]
              n1918 = Increment(x=w3429) -> (x+1=w3428:i32)
              n1919 = call "设置指定通道的测频基准脉冲周期.vi"("错误输入"=w3432, "freqBase_ms"=1000.0, "chNo"=w3428, "设备句柄入"=w3431) -> ("错误输出"=w3427:errorcluster)  [unwired: 5 in, 2 out]
            }
          }
          event "计数器清零 2": Value Change {
            n1920 = event-data() -> ()  [unwired: 1 in, 5 out]
            n1921 = for {
              N: 6 -> [_]
              tunnel: w3436 -> [w3441]
              tunnel: w3435 -> [w3440]
              tunnel: [w3439] -> w3434
              i -> [w3438]
              n1922 = Increment(x=w3438) -> (x+1=w3437:i32)
              n1923 = call "指定通道计数器清零.vi"("错误输入"=w3440, "chNo"=w3437, "设备句柄入"=w3441) -> ("错误输出"=w3439:errorcluster)  [unwired: 7 in, 1 out]
            }
          }
          event "PWM输出 2": Value Change {
            n1924 = event-data() -> ("OldVal"=w3442:bool)  [unwired: 1 in, 4 out]
            n1925 = local write "PWM输出 2"(w3442) -> ()
            n1926 = call "设置开关量方向.vi"("错误输入"=w3468, "方向"=i8[] [1, 1], "设备句柄入"=w3469) -> ("错误输出"=w3466:errorcluster, "设备句柄"=w3467:i32)  [unwired: 7 in]
            n1927 = call "设置PWM频率和占空比.vi"("占空比(0~1)"="占空比(0~1) 6", "频率"="频率1 2", "错误输入"=w3466, "通道号"=1, "设备句柄入"=w3467) -> ("错误输出"=w3458:errorcluster, "设备句柄"=w3452:i32, "实际占空比"=→"实际占空比 6":dbl, "实际频率"=→"实际频率 6":dbl)  [unwired: 3 in]
            n1928 = call "设置PWM频率和占空比.vi"("占空比(0~1)"="占空比(0~1) 5", "频率"="频率2 2", "错误输入"=w3458, "通道号"=2, "设备句柄入"=w3452) -> ("错误输出"=w3451:errorcluster, "设备句柄"=w3453:i32, "实际占空比"=→"实际占空比 5":dbl, "实际频率"=→"实际频率 5":dbl)  [unwired: 3 in]
            n1929 = call "设置PWM频率和占空比.vi"("占空比(0~1)"="占空比(0~1) 4", "频率"="频率3 2", "错误输入"=w3451, "通道号"=3, "设备句柄入"=w3453) -> ("错误输出"=w3445:errorcluster, "设备句柄"=w3446:i32, "实际占空比"=→"实际占空比 4":dbl, "实际频率"=→"实际频率 4":dbl)  [unwired: 3 in]
            n1930 = call "使能或禁止PWM输出.vi"("错误输入"=w3445, "所用PWM使能"=i8 1, "设备句柄入"=w3446) -> ("错误输出"=w3444:errorcluster)  [unwired: 7 in, 1 out]
          }
          event "M系列PWM输出 2": Value Change {
            w3478 = 2 ("通道号")
            w3473 = 0.5 ("占空比(0~1)")
            w3474 = 2000.0 ("频率")
            w3486 = 1 ("通道号")
            n1931 = event-data() -> ()  [unwired: 1 in, 5 out]
            n1932 = call "设置开关量方向.vi"("错误输入"=w3490, "方向"=i8[] [1, 1], "设备句柄入"=w3491) -> ("错误输出"=w3488:errorcluster, "设备句柄"=w3489:i32)  [unwired: 7 in]
            n1933 = call "设置PWM频率和占空比.vi"("占空比(0~1)"=w3473, "频率"=w3474, "错误输入"=w3488, "通道号"=w3486, "设备句柄入"=w3489) -> ("错误输出"=w3484:errorcluster, "设备句柄"=w3487:i32)  [unwired: 3 in, 2 out]
            n1934 = call "设定输出脉冲个数.vi"("错误输入"=w3484, "脉冲个数"="设定输出脉冲个数 2", "通道号"=w3486, "设备句柄入"=w3487) -> ("错误输出"=w3476:errorcluster, "设备句柄"=w3475:i32)  [unwired: 2 in]
            n1935 = call "设置PWM频率和占空比.vi"("占空比(0~1)"=w3473, "频率"=w3474, "错误输入"=w3476, "通道号"=w3478, "设备句柄入"=w3475) -> ("错误输出"=w3477:errorcluster, "设备句柄"=w3479:i32)  [unwired: 3 in, 2 out]
            n1936 = call "设定输出脉冲个数.vi"("错误输入"=w3477, "通道号"=w3478, "设备句柄入"=w3479) -> ("错误输出"=w3471:errorcluster, "设备句柄"=w3472:i32)  [unwired: 3 in]
            n1937 = call "使能或禁止PWM输出(只支持EM9636M).vi"("错误输入"=w3471, "相位设置数组"=i8[] [1, 0, 0] ("PWM使能"), "PWM使能"=i8[] [1, 1, 0], "设备句柄入"=w3472) -> ("错误输出"=w3483:errorcluster)  [unwired: 6 in, 1 out]
          }
          event "设置开关量方向 3": Value Change {
            n1938 = event-data() -> ()  [unwired: 1 in, 5 out]
            n1939 = Cluster To Array(cluster="设置开关量方向 2") -> (array=w3492:i8[])
            "数组 7" <- w3492
            n1940 = call "设置开关量方向.vi"("错误输入"=w3495, "方向"=w3492, "设备句柄入"=w3496) -> ("错误输出"=w3494:errorcluster)  [unwired: 7 in, 1 out]
          }
          event "光隔离输出 2", "可编程数字量I/O 2": Value Change {
            n1941 = event-data() -> ()  [unwired: 1 in, 5 out]
            n1942 = local read "光隔离输入 2"() -> (w3503:bool[])
            n1943 = Cluster To Array(cluster="可编程数字量I/O 2") -> (array=w3497:bool[])
            n1944 = Build Array (concatenate)(w3497, w3503, "光隔离输出 2") -> (w3501:bool[])
            n1945 = Boolean To (0,1)(Boolean=w3501) -> (0, 1=w3500:i16[])
            n1946 = To Byte Integer(number=w3500) -> (8bit integer=w3499:i8[])
            n1947 = call "设置所有通道开关量值.vi"("错误输入"=w3505, "oStatus"=w3499, "设备句柄入"=w3506) -> ("错误输出"=w3504:errorcluster)  [unwired: 7 in, 1 out]
          }
          event "DA输出 2", "CH1 2", "CH2 2", "CH3 2", "CH4 2": Value Change {
            n1948 = event-data() -> ()  [unwired: 1 in, 5 out]
            n1949 = for {
              N: 4 -> [_]
              tunnel: w3527 -> [w3535]
              tunnel: w3526 -> [w3534]
              tunnel: "DA输出范围 2" -> [w3530]
              tunnel: [w3529] -> w3524
              tunnel: [w3528] -> w3523
              i -> [w3532]
              n1950 = Increment(x=w3532) -> (x+1=w3533:i32)
              n1951 = call "DA输出方式.vi"("输出范围"=w3530, "错误输入"=w3534, "输出值方式"=i16 1, "通道号"=w3533, "设备句柄入"=w3535) -> ("错误输出"=w3529:errorcluster, "设备句柄"=w3528:i32)  [unwired: 5 in]
            }
            n1952 = call "设置DA输出值.vi"("错误输入"=w3524, "输出值"="CH1 2", "通道号"=1, "设备句柄入"=w3523) -> ("错误输出"=w3517:errorcluster, "设备句柄"=w3519:i32)  [unwired: 6 in]
            n1953 = call "设置DA输出值.vi"("错误输入"=w3517, "输出值"="CH2 2", "通道号"=2, "设备句柄入"=w3519) -> ("错误输出"=w3511:errorcluster, "设备句柄"=w3516:i32)  [unwired: 6 in]
            n1954 = call "设置DA输出值.vi"("错误输入"=w3511, "输出值"="CH3 2", "通道号"=3, "设备句柄入"=w3516) -> ("错误输出"=w3510:errorcluster, "设备句柄"=w3515:i32)  [unwired: 6 in]
            n1955 = call "设置DA输出值.vi"("错误输入"=w3510, "输出值"="CH4 2", "通道号"=4, "设备句柄入"=w3515) -> ("错误输出"=w3508:errorcluster)  [unwired: 6 in, 1 out]
          }
          event "编码器清零 2": Value Change {
            n1956 = event-data() -> ()  [unwired: 1 in, 5 out]
            n1957 = call "编码器清零.vi"("错误输入"=w3541, "通道号"=1, "设备句柄入"=w3542) -> ("错误输出"=w3537:errorcluster, "设备句柄"=w3538:i32)  [unwired: 7 in]
            n1958 = call "编码器清零.vi"("错误输入"=w3537, "通道号"=2, "设备句柄入"=w3538) -> ("错误输出"=w3536:errorcluster)  [unwired: 7 in, 1 out]
          }
          event "DA输出范围 2": Value Change {
            n1959 = event-data() -> ()  [unwired: 1 in, 5 out]
            n1960 = local read "DA输出范围 2"() -> (w3546:i32)
            n1961 = case shown="4" w3546 {
              tunnel: [10000.0 ("标尺.范围:最大值") 5000.0 ("标尺.范围:最大值") 10000.0 ("标尺.范围:最大值") 5000.0 ("标尺.范围:最大值") 20000.0 ("标尺.范围:最大值")] -> w3544
              tunnel: [-10000.0 ("标尺.范围:最大值") -5000.0 ("标尺.范围:最大值") 0.0 ("标尺.范围:最大值") 0.0 ("标尺.范围:最大值") 0.0 ("标尺.范围:最大值")] -> w3543
              frame 0, Default {
              }
              frame 1 {
              }
              frame 2 {
              }
              frame 3 {
              }
              frame 4 {
              }
            }
            n1962 = property on="CH1 2" class="Slide (严格)"("Scale.Maximum"=w3544, "Scale.Minimum"=w3543) -> ()  [unwired: 2 in, 2 out]
            n1963 = property on="CH2 2" class="Slide (严格)"("Scale.Maximum"=w3544, "Scale.Minimum"=w3543) -> ()  [unwired: 2 in, 2 out]
            n1964 = property on="CH3 2" class="Slide (严格)"("Scale.Maximum"=w3544, "Scale.Minimum"=w3543) -> ()  [unwired: 2 in, 2 out]
            n1965 = property on="CH4 2" class="Slide (严格)"("Scale.Maximum"=w3544, "Scale.Minimum"=w3543) -> ()  [unwired: 2 in, 2 out]
          }
          event "M系列PWM停止 2": Value Change {
            n1966 = event-data() -> ()  [unwired: 1 in, 5 out]
            n1967 = call "使能或禁止PWM输出(只支持EM9636M).vi"("错误输入"=w3559, "相位设置数组"=i8[] [0, 0, 0] ("PWM使能"), "PWM使能"=i8[] [0, 0, 0], "设备句柄入"=w3560) -> ("错误输出"=w3558:errorcluster)  [unwired: 6 in, 1 out]
          }
          event "PWM停止 2": Value Change {
            n1968 = event-data() -> ()  [unwired: 1 in, 5 out]
            n1969 = call "使能或禁止PWM输出.vi"("错误输入"=w3564, "所用PWM使能"=i8 0, "设备句柄入"=w3565) -> ("错误输出"=w3562:errorcluster)  [unwired: 7 in, 1 out]
          }
        }
        "错误输出 4" <- w3318
        n1970 = local read "停止"() -> (w3321:bool)
      }
    }
    frame #2 {
      n1971 = flat-sequence {
        tunnel: [w3613] -> w3609
        tunnel: [w3611] -> w3608
        tunnel: w3609 -> [w3619]
        tunnel: [w3618] -> w3607
        tunnel: w3608 -> [w3617]
        tunnel: [w3616] -> w3606
        tunnel: w3607 -> [w3625]
        tunnel: [w3624] -> w3605
        tunnel: w3606 -> [w3623]
        tunnel: [w3622] -> w3604
        tunnel: w3605 -> [w3630]
        tunnel: [w3629] -> w3603
        tunnel: w3604 -> [w3628]
        tunnel: w3603 -> [w3631]
        frame #0 {
          n1972 = local read "设备句柄 2"() -> (w3614:i32)
          n1973 = local read "错误输出 6"() -> (w3612:errorcluster)
          n1974 = call "停止采集(M).vi"("错误输入"=w3612, "设备句柄入"=w3614) -> ("错误输出"=w3611:errorcluster, "设备句柄"=w3613:i32)  [unwired: 8 in]
          n1975 = Wait (ms)(milliseconds to wait=u32 10 ("等待时间（毫秒）")) -> ()  [unwired: 1 out]
        }
        frame #1 {
          n1976 = call "使能或禁止PWM输出.vi"("错误输入"=w3617, "所用PWM使能"=i8 0, "设备句柄入"=w3619) -> ("错误输出"=w3616:errorcluster, "设备句柄"=w3618:i32)  [unwired: 7 in]
          n1977 = Wait (ms)(milliseconds to wait=u32 10 ("等待时间（毫秒）")) -> ()  [unwired: 1 out]
        }
        frame #2 {
          n1978 = call "关闭数据连接.vi"("错误输入"=w3623, "设备句柄入"=w3625) -> ("错误输出"=w3622:errorcluster, "设备句柄"=w3624:i32)  [unwired: 8 in]
          n1979 = Wait (ms)(milliseconds to wait=u32 10 ("等待时间（毫秒）")) -> ()  [unwired: 1 out]
        }
        frame #3 {
          n1980 = call "关闭命令连接.vi"("错误输入"=w3628, "设备句柄入"=w3630) -> ("错误输出"=w3627:errorcluster, "设备句柄"=w3629:i32)  [unwired: 8 in]
          n1981 = Wait (ms)(milliseconds to wait=u32 10 ("等待时间（毫秒）")) -> ()  [unwired: 1 out]
          n1982 = local write "错误输出 6"(w3627) -> ()
        }
        frame #4 {
          n1983 = call "关闭设备.vi"("设备句柄"=w3631) -> ()  [unwired: 10 in]
        }
        frame #5 {
          "close2" <- TRUE ("close2")
        }
      }
    }
  }
  n1984 = local read "平均速度数组"() -> (w15:dbl[])
  n1985 = local read "D1平均速度"() -> (w16:dbl)
  n1986 = Build Array (concatenate)(w15, w16) -> (→"平均速度数组":dbl[])
  n1987 = disable-structure shown="启用" {
    disable-tunnel: w26 -> [w3634 _]
    disable-tunnel: 0 -> [w3633 _]
    frame Disabled {
      n1988 = while "数据更新线程" {
        tunnel: w3634 -> [w3648]
        shift-right: [w3639] -> _
        shift-left: _ -> [w3644]
        shift-right: [w3640] -> _
        shift-left: w3633 -> [w3643]
        stop <- w3646 stop-if-true
        n1989 = Dequeue Element(queue=w3648, timeout in ms (-1)=5 ("超时毫秒(-1)")) -> (element=w3645:T13, timed out?=w3638:bool, error out=w3646:errorcluster)  [unwired: 1 in, 1 out]
        n1990 = case shown="假" w3638 {
          tunnel: w3645 -> [w3659 _]
          tunnel: w3644 -> [w3662 w3670]
          tunnel: [w3655 w3670] -> w3642
          tunnel: w3643 -> [w3658 w3669]
          tunnel: [w3656 w3669] -> w3641
          frame False {
            n1991 = Insert Into Array(array=w3662, new element=w3659) -> (w3660:T13)  [unwired: 1 in]
            n1992 = Array Size(array=w3660) -> (size(s)=w3661:i32)
            n1993 = case "最多保存500帧" shown="501.." w3661 {
              selector: w3661 -> [_ w3667]
              tunnel: w3660 -> [w3663 w3668]
              tunnel: [w3663 w3665] -> w3655
              tunnel: [_ w3664] -> w3657
              frame 0, Default {
              }
              frame 501.. {
                n1994 = Subtract(x=w3667, y=500) -> (x-y=w3664:i32)
                n1995 = Array Subset(array=w3668, index=w3664) -> (w3665:T13)  [unwired: 1 in]
              }
            }
            n1996 = Add(x=w3658, y=w3657) -> (x+y=w3656:i32)
          }
          frame True {
          }
        }
        n1997 = Not(x=w3638) -> (.not. x?=w3637:bool)
        n1998 = case shown="真" "Clear" {
          tunnel: w3641 -> [w3653 _]
          tunnel: w3642 -> [w3654 _]
          tunnel: [w3654 _] -> w3639
          tunnel: [w3653 _] -> w3640
          frame False {
          }
          frame True {
          }
        }
        n1999 = Or(x="Clear", y=w3637) -> (x .or. y?=w3636:bool)
        n2000 = case shown="真" w3636 {
          tunnel: w3640 -> [_ w3650]
          tunnel: w3639 -> [_ w3649]
          frame False {
          }
          frame True {
            n2001 = control-ref of="本VI"() -> (w3651:refnum<vi>)
            n2002 = control-ref of="list"() -> (w3652:refnum<vi>)
            n2003 = call "Demo_UpdateList.vi"("Offset"=w3650, "Buffer"=w3649, "list"=w3652, "MainVi"=w3651) -> ()  [unwired: 8 out]
          }
        }
      }
    }
    frame Enabled {
    }
  }
  n2004 = while "接收线程" {
    tunnel: w26 -> [w3677]
    shift-right: [w3675] -> _
    shift-left: u32 0 ("RecvCnt") -> [w3676]
    shift-right: [w3673] -> _
    shift-left: "" ("档位") -> [w3674]
    stop <- w3672 stop-if-true
    n2005 = local read "Open"() -> (w3678:bool)
    n2006 = case shown="真" w3678 {
      tunnel: w3677 -> [_ w3688]
      tunnel: w3676 -> [w3680 w3687]
      tunnel: [w3680 w3686] -> w3675
      tunnel: w3674 -> [w3679 w3683]
      tunnel: [w3679 w3682] -> w3673
      frame False {
        # "CAN未打开，延时50ms"
        n2007 = Wait (ms)(milliseconds to wait=u32 50 ("等待时间（毫秒）")) -> ()  [unwired: 1 out]
      }
      frame True {
        n2008 = local read "DevType"() -> (w3691:T3)
        n2009 = local read "Channel"() -> (w3685:T4)
        n2010 = call "VCI_Receive.vi"("CANIndex"=w3685, "DevIndex"=u32 0, "DevType"=w3691) -> ("Recieve"=w3684:T12[])  [unwired: 3 in, 5 out]
        n2011 = Empty Array?(array=w3684) -> (empty?=w3689:bool)
        n2012 = case shown="假" w3689 {
          tunnel: w3688 -> [w3704 _]
          tunnel: w3684 -> [w3696 _]
          tunnel: [w3701 _] -> _
          tunnel: w3687 -> [w3699 w3723]
          tunnel: [w3698 w3723] -> w3686
          tunnel: w3685 -> [w3697 _]
          tunnel: w3683 -> [w3695 w3722]
          tunnel: [w3694 w3722] -> w3682
          frame False {
            n2013 = Array Size(array=w3696) -> (size(s)=w3700:i32)
            n2014 = call "Demo_MakeDispBuff.vi"("Channel"=w3697, "Type"=enum16{"接收", "发送"}."接收", "OBJs"=w3696) -> ("Buffer"=w3702:T13)
            n2015 = Add(x=w3700, y=w3699) -> (x+y=w3698:u32)
            "RecvCnt" <- w3698
            n2016 = for {
              tunnel: w3696 -> [w3712] mode=indexing
              tunnel: w3695 -> [w3709]
              tunnel: [w3708] -> w3694
              n2017 = Unbundle By Name(w3712) -> ("ID"=w3711:u32, "Data"=w3710:u8[])
              n2018 = case shown="18A" w3711 {
                tunnel: w3710 -> [_ w3718]
                tunnel: w3709 -> [w3713 _]
                tunnel: [w3713 _] -> w3708
                frame 0, Default {
                }
                frame 394 {
                  n2019 = Index Array(array=w3718) -> (element #3=w3717:u8, element #4=w3716:u8)  [unwired: 6 in, 4 out]
                  n2020 = Number To Boolean Array(number=w3716) -> (Boolean array=→"布尔数组 2":bool[])
                  n2021 = Number To Boolean Array(number=w3717) -> (Boolean array=→"布尔数组":bool[])
                }
              }
            }
            n2022 = disable-structure shown="禁用" {
              disable-tunnel: w3704 -> [w3707 _]
              disable-tunnel: w3702 -> [w3706 _]
              disable-tunnel: [w3705 _] -> w3701
              frame Disabled {
                n2023 = Enqueue Element(queue=w3707, element=w3706) -> (error out=w3705:errorcluster)  [unwired: 1 in, 3 out]
              }
              frame Enabled {
              }
            }
            n2024 = local write "comcnt"(u16 0 ("comcnt")) -> ()
            "遥控器通讯" <- FALSE ("遥控器通讯")
          }
          frame True {
            n2025 = local write "遥控器通讯"(TRUE ("遥控器通讯")) -> ()
            n2026 = property on="comcnt" class="DigNum (严格)"() -> ("Value"=w3719:u16)  [unwired: 2 in, 2 out]
            n2027 = Increment(x=w3719) -> (x+1=→"comcnt":u16)
          }
        }
      }
    }
    n2028 = local read "停止"() -> (w3672:bool)
    n2029 = Wait (ms)(milliseconds to wait=u32 50 ("等待时间（毫秒）")) -> ()  [unwired: 1 out]
  }
  n2030 = Release Queue(queue=w11) -> ()  [unwired: 2 in, 3 out]
  n2031 = disable-structure shown="禁用" {
    disable-tunnel: w4 -> [w3725 _]
    frame Disabled {
      n2032 = control-ref of="本应用程序"() -> (w3727:refnum<vi>)
      n2033 = invoke class="VI" method="FP.Close"(error in=w3725) -> (error out=w3724:errorcluster)  [unwired: 2 in, 2 out]
      n2034 = property class="App"(reference=w3727) -> ("App.Kind"=w3726:T19)  [unwired: 1 in, 2 out]
      n2035 = case shown="\"Development System\"" w3726 {
        tunnel: w3724 -> [_ _]
        frame "invalid app kind", Default {
          n2036 = Quit LabVIEW() -> ()  [unwired: 1 out]
        }
        frame "Development System" {
        }
      }
    }
    frame Enabled {
    }
  }
  n2037 = while {
    stop <- FALSE stop-if-true
    n2038 = local read "close2"() -> (w3730:bool)
    n2039 = local read "close"() -> (w3731:bool)
    n2040 = And(x=w3731, y=w3730) -> (x .and. y?=w3729:bool)
    n2041 = case shown="真" w3729 {
      frame False {
      }
      frame True {
        n2042 = flat-sequence {
          frame #0 {
            w3741 = FALSE ("close")
            n2043 = local read "Config"() -> (w3740:T9)
            n2044 = local write "close"(w3741) -> ()
            n2045 = local write "close2"(w3741) -> ()
            n2046 = Unbundle By Name(w3740) -> ("DevType"=w3739:T3, "DevIndex"=w3738:u32)
            n2047 = call "VCI_CloseDevice.vi"("DevIndex"=w3738, "DevType"=w3739) -> ()  [unwired: 1 in, 9 out]
            n2048 = Wait (ms)(milliseconds to wait=u32 50 ("等待时间（毫秒）")) -> ()  [unwired: 1 out]
          }
          frame #1 {
            n2049 = Stop(stop? (T)=TRUE ("停止？(T)")) -> ()
          }
        }
      }
    }
    n2050 = local read "对话框传递"() -> (w3728:bool)
    n2051 = Wait (ms)(milliseconds to wait=u32 5 ("等待时间（毫秒）")) -> ()  [unwired: 1 out]
    n2052 = case shown="真" w3728 {
      frame False {
      }
      frame True {
        n2053 = One Button Dialog(message="温度超过70℃\n请选择查看数据菜单确认" ("消息")) -> (true=w3735:bool)  [unwired: 1 in]
        n2054 = Not(x=w3735) -> (.not. x?=w3734:bool)
        n2055 = local write "对话框传递"(w3734) -> ()
      }
    }
  }
  n2056 = while {
    stop <- w3750 stop-if-true
    n2057 = local read "对话框"() -> (w3743:bool)
    n2058 = local read "到期了"() -> (w3747:bool)
    n2059 = call "初始化.vi"() -> ("first row"=w3751:dbl[], "最终选择的真实日期"=w3752:dbl[], "密码"=w3753:string[][])  [unwired: 3 in]
    n2060 = case shown="真" w3743 {
      frame False {
      }
      frame True {
        n2061 = flat-sequence {
          frame #0 {
            n2062 = One Button Dialog(message="试用期已到，电机将无法加载，请输入密码" ("消息")) -> ()  [unwired: 1 in, 1 out]
          }
          frame #1 {
            n2063 = local write "对话框"(FALSE ("对话框")) -> ()
          }
        }
      }
    }
    n2064 = case shown="真" w3747 {
      frame False {
        n2065 = property on="密码输入" class="Str"("Visible"=FALSE ("可见")) -> ()  [unwired: 2 in, 2 out]
      }
      frame True {
        w3758 = i16 0 ("驱动电机转速下给定")
        n2066 = property on="密码输入" class="Str"("Visible"=TRUE ("可见")) -> ()  [unwired: 2 in, 2 out]
        n2067 = local write "加载电机左下转矩给定"(w3758) -> ()
        n2068 = local write "加载电机右下转矩给定"(w3758) -> ()
        n2069 = local write "加载电机右上转矩给定"(w3758) -> ()
        n2070 = local write "驱动电机上转速给定"(w3758) -> ()
        n2071 = local write "驱动电机转速下给定"(w3758) -> ()
        n2072 = local write "加载电机左上转矩给定"(w3758) -> ()
      }
    }
    n2073 = Wait (ms)(milliseconds to wait=u32 500 ("等待时间（毫秒）")) -> ()  [unwired: 1 out]
    n2074 = call "到期.vi"("最终选择的真实的日期"=w3752, "加期限后的日期"=w3751, "密码和期限"=w3753, "密码输入"="密码输入") -> ("到期了"=w3746:bool)  [unwired: 1 out]
    "到期了" <- w3746
    n2075 = call <vilib>:"Boolean Crossing PtByPt.vi"("direction"=enum16{"either", "false-true", "true-false"}."false-true", "input"=w3746) -> ("crossing"=w3744:bool)  [unwired: 1 in]
    n2076 = case shown="真" w3744 {
      frame False {
      }
      frame True {
        "对话框" <- TRUE ("对话框")
      }
    }
    n2077 = local read "停止"() -> (w3750:bool)
  }
  n2078 = call-dynamic "Close.vi"("error in (no error)"=w25, "Modbus master in"=w24) -> ("error out"=w9:errorcluster)  [unwired: 9 in]
  n2079 = call <vilib>:"Clear Errors.vi"("error in (no error)"=w9) -> ()  [unwired: 5 in, 2 out]
